vi "WVDIAL_3A_Data_v1.vi"() -> ()   [LabVIEW 2012]
uses:
  C:/H2O_DIAL/LabVIEW-2012/Newport_LabVIEW_v3-0-2/LabVIEW 2009/PowerMeterCommands.dll
  H2O_DIAL/LabVIEW-2012/Newport_LabVIEW_v3-0-2/LabVIEW 2009/PowerMeterCommands.dll
  <vilib>/DAQmx/write.llb/DAQmx Write (Digital 1D Bool NChan 1Samp 1Line).vi
  <vilib>/DAQmx/miscellaneous.llb/DAQmx Fill In Error Info.vi
  <vilib>/Analysis/baseanly.llb/Mean (DBL).vi
  H2O_DIAL/LabVIEW-2012/Scalar_Data.vi
  H2O_DIAL/LabVIEW-2012/Bristol WM V2_31b/CLDevIFace.dll
  <vilib>/Analysis/NI_AALBase.lvlib
panel:
  out "FileHour":i32=18
  out "L_Count":i32=437
  out "sigma_off_total":dbl[](array[numeric])=[4.970068414914426e-25, 4.935109344576291e-25, 4.900296426937575e-25, 4.865629933162525e-25, 4.8311101300892405e-25, 4.796737279795042e-25, 4.762511639263623e-25, 4.728433460005277e-25, 4.694502987714828e-25, 4.66072046190942e-25, 4.627086115623767e-25, 4.5936001750771025e-25, 4.560262859388569e-25, 4.5270743802518285e-25, 4.494034941687391e-25, 4.4611447397771265e-25, 4.428403962379541e-25, 4.395812788908677e-25, 4.363371390116038e-25, 4.331079927877316e-25, 4.298938554952973e-25, 4.2669474148461465e-25, 4.235106641622183e-25, 4.203416359713408e-25, 4.171876683809042e-25, 4.14048771871945e-25, 4.1092495592023437e-25, 4.0781622899252965e-25, 4.047225985294158e-25, 4.016440709475411e-25, 3.9858065161821437e-25, 3.955323448748479e-25, 3.9249915399689097e-25, 3.8948108121823377e-25, 3.864781277119762e-25, 3.8349029359894115e-25, 3.8051757794122746e-25, 3.7755997874807175e-25, 3.7461749297351587e-25, 3.7169011652144367e-25, 3.687778442479969e-25, 3.6588066996856557e-25, 3.629985864619472e-25, 3.6013158547695413e-25, 3.572796577416277e-25, 3.544427929672661e-25, 3.516209798625218e-25, 3.488142061394692e-25, 3.460224585304242e-25, 3.432457227878348e-25, 3.4048398370653397e-25, 3.3773722513359157e-25, 3.350054299768194e-25, 3.3228858022516937e-25, 3.295866569574933e-25, 3.268996403598237e-25, 3.2422750973929355e-25, 3.21570243540853e-25, 3.189278193592863e-25, 3.163002139636937e-25, 3.136874033014969e-25, 3.110893625253726e-25, 3.085060660050822e-25, 3.059374873481082e-25, 3.0338359941112116e-25, 3.008443743235647e-25, 2.9831978349953457e-25, 2.95809797659182e-25, 2.9331438684538516e-25, 2.9083352043781934e-25, 2.8836716717543507e-25, 2.859152951716739e-25, 2.834778719288951e-25, 2.810548643615105e-25, 2.7864623880639067e-25, 2.7625196104499907e-25, 2.738719963159808e-25, 2.7150630933496113e-25, 2.691548643092545e-25, 2.6681762495199362e-25, 2.6449455450241973e-25, 2.6218561573515237e-25, 2.5989077097963764e-25, 2.5760998213569394e-25, 2.553432106812723e-25, 2.5309041769453305e-25, 2.508515638628236e-25, 2.486266094966773e-25, 2.4641551454270873e-25, 2.4421823859627355e-25, 2.4203474091280046e-25, 2.398649804208083e-25, 2.3770891573121883e-25, 2.3556650514992666e-25, 2.334377066857522e-25, 2.3132247806240595e-25, 2.292207767270247e-25, 2.2713255985837977e-25, 2.250577843763165e-25, 2.2299640695179534e-25, 2.209483840081283e-25, 2.1891367173745365e-25, 2.1689222609956e-25, 2.1488400283134808e-25, 2.1288895745535377e-25, 2.1090704528070817e-25, 2.089382214122218e-25, 2.0698244075371163e-25, 2.0503965801268946e-25, 2.0310982770672953e-25, 2.0119290416275883e-25, 1.9928884152720694e-25, 1.9739759376467061e-25, 1.9551911466442564e-25, 1.9365335784015228e-25, 1.9180027673647352e-25, 1.8995982463109612e-25, 1.8813195463488326e-25, 1.8631661969818019e-25, 1.8451377261048445e-25, 1.8272336600511332e-25, 1.8094535235979458e-25, 1.7917968400156795e-25, 1.774263131074251e-25, 1.7568519170769187e-25, 1.7395627168958116e-25, 1.7223950479810698e-25, 1.7053484264204325e-25, 1.6884223669495872e-25, 1.671616383006639e-25, 1.6549299867335668e-25, 1.6383626890674343e-25, 1.6219139997488532e-25, 1.6055834273756572e-25, 1.5893704794600627e-25, 1.573274662463159e-25, 1.5572954818878462e-25, 1.5414324422878638e-25, 1.5256850473874784e-25, 1.510052800101514e-25, 1.4945352026447543e-25, 1.4791317565791618e-25, 1.4638419629201228e-25, 1.448665322199304e-25, 1.4336013345653925e-25, 1.4186494998679763e-25, 1.403809317759688e-25, 1.3890802877992275e-25, 1.374461909533494e-25, 1.3599536826304997e-25, 1.3455551069680852e-25, 1.331265682750014e-25, 1.317084910617463e-25, 1.3030122917788643e-25, 1.2890473280950027e-25, 1.2751895222264232e-25, 1.261438377738064e-25, 1.247793399209599e-25, 1.2342540923695054e-25, 1.2208199641934536e-25, 1.207490523039559e-25, 1.194265278734551e-25, 1.1811437427102546e-25, 1.1681254280970297e-25, 1.1552098498187396e-25, 1.1423965247193127e-25, 1.129684971621386e-25, 1.1170747114439217e-25, 1.1045652672740435e-25, 1.0921561644348792e-25, 1.0798469305651514e-25, 1.0676370956928575e-25, 1.055526192264184e-25, 1.0435137552017687e-25, 1.0315993219529312e-25, 1.0197824325066935e-25, 1.0080626294155857e-25, 9.964394578070562e-26, 9.849124653878678e-26, 9.734812024396337e-26, 9.621452217958014e-26, 9.509040788153638e-26, 9.397573313474797e-26, 9.2870453969155e-26, 9.177452665388814e-26, 9.068790769077486e-26, 8.961055380771591e-26, 8.854242195025276e-26, 8.748346927326784e-26, 8.643365313126359e-26, 8.539293106813325e-26, 8.436126080659389e-26, 8.333860023704058e-26, 8.232490740501524e-26, 8.132014049957187e-26, 8.032425783987688e-26, 7.933721786336048e-26, 7.835897911055001e-26, 7.738950021374666e-26, 7.642873988181704e-26, 7.547665688745864e-26, 7.453321005260971e-26, 7.3598358236196e-26, 7.267206031959588e-26, 7.17542751940349e-26, 7.084496174723345e-26, 6.99440788514668e-26, 6.905158535007224e-26, 6.816744004751336e-26, 6.729160169573299e-26, 6.64240289857379e-26, 6.5564680535091e-26, 6.471351488011949e-26, 6.387049046546095e-26, 6.303556563639124e-26, 6.220869863111731e-26, 6.138984757339889e-26, 6.057897046626043e-26, 5.977602518710106e-26, 5.898096948146685e-26, 5.819376096018969e-26, 5.741435709543367e-26, 5.664271521783085e-26, 5.587879251486328e-26, 5.51225460295526e-26, 5.437393265946454e-26, 5.363290915754907e-26, 5.289943213256812e-26, 5.217345804999475e-26, 5.1454943235195867e-26, 5.074384387521688e-26, 5.0040116022138814e-26, 4.9343715597454284e-26, 4.8654598395691204e-26, 4.7972720089551445e-26, 4.729803623551307e-26, 4.663050227875443e-26, 4.597007356046831e-26, 4.531670532379107e-26, 4.4670352720694333e-26, 4.4030970819662006e-26, 4.3398514613184746e-26, 4.2772939025846054e-26, 4.215419892254647e-26, 4.154224911690283e-26, 4.093704438021407e-26, 4.0338539450472376e-26, 3.9746689041273814e-26, 3.916144785197283e-26, 3.8582770576425204e-26, 3.8010611913639447e-26, 3.74449265772608e-26, 3.6885669306098596e-26, 3.6332794874218655e-26, 3.578625810171199e-26, 3.5246013865492145e-26, 3.4712017109920907e-26, 3.418422285823819e-26, 3.3662586223724155e-26, 3.31470624215432e-26, 3.2637606780392576e-26, 3.2134174754533765e-26, 3.163672193659779e-26, 3.114520407010239e-26, 3.0659577062623985e-26, 3.017979699957737e-26, 2.970582015834633e-26, 2.9237603022681873e-26, 2.877510229831183e-26, 2.831827492878117e-26, 2.786707811220407e-26, 2.7421469318983614e-26, 2.698140631035692e-26, 2.6546847158190514e-26, 2.6117750266015116e-26, 2.56940743913942e-26, 2.527577866977577e-26]
  out "sigma_on_total":dbl[](array[numeric])=[3.533865838600727e-23, 3.533764161681225e-23, 3.5333977469404133e-23, 3.53276568192525e-23, 3.531867144357016e-23, 3.530701403122502e-23, 3.529267819280469e-23, 3.527565846749943e-23, 3.525595033343317e-23, 3.523355021225782e-23, 3.52084554780571e-23, 3.5180664458671094e-23, 3.5150176447433637e-23, 3.511699169858595e-23, 3.508111143749733e-23, 3.5042537860569434e-23, 3.5001274136929736e-23, 3.495732440751245e-23, 3.4910693790546564e-23, 3.486138837361377e-23, 3.4809415218446414e-23, 3.4754782353092596e-23, 3.4697498774262163e-23, 3.463757443779839e-23, 3.4575020259466816e-23, 3.450984810279872e-23, 3.444207077926451e-23, 3.4371702036366597e-23, 3.429875655153695e-23, 3.422324992434722e-23, 3.414519866506169e-23, 3.406462018237782e-23, 3.3981532779195215e-23, 3.3895955634047386e-23, 3.3807908790536376e-23, 3.371741314710812e-23, 3.3624490438242643e-23, 3.352916322385855e-23, 3.3431454873140853e-23, 3.3331389544696416e-23, 3.322899217813418e-23, 3.3124288469010065e-23, 3.301730485625495e-23, 3.2908068501003093e-23, 3.2796607270971934e-23, 3.268294971825446e-23, 3.256712506069342e-23, 3.244916316282518e-23, 3.2329094515384454e-23, 3.2206950210285986e-23, 3.208276192552656e-23, 3.1956561900495705e-23, 3.182838291197626e-23, 3.169825825503171e-23, 3.156622172157982e-23, 3.143230757250406e-23, 3.129655051889506e-23, 3.115898569897651e-23, 3.101964865071464e-23, 3.087857529576123e-23, 3.0735801908728846e-23, 3.059136509681361e-23, 3.0445301776261984e-23, 3.0297649149870386e-23, 3.014844467928977e-23, 2.9997726067801886e-23, 2.984553123065604e-23, 2.969189827592652e-23, 2.9536865479241003e-23, 2.938047126177763e-23, 2.922275416635555e-23, 2.906375283683212e-23, 2.8903505991494374e-23, 2.874205240602245e-23, 2.8579430887383764e-23, 2.8415680253195745e-23, 2.82508393124097e-23, 2.8084946841160186e-23, 2.791804156410952e-23, 2.775016213305788e-23, 2.758134710797806e-23, 2.741163493435856e-23, 2.7241063929107007e-23, 2.706967225870395e-23, 2.6897497917834795e-23, 2.67245787185707e-23, 2.6550952266852455e-23, 2.6376655947539815e-23, 2.6201726909898208e-23, 2.602620204658551e-23, 2.585011798410415e-23, 2.567351106279476e-23, 2.5496417325287913e-23, 2.5318872500516e-23, 2.5140911992175055e-23, 2.4962570863782866e-23, 2.478388382719878e-23, 2.4604885230681298e-23, 2.4425609047468987e-23, 2.4246088864884145e-23, 2.4066357872066157e-23, 2.3886448853935633e-23, 2.3706394178067187e-23, 2.3526225788721896e-23, 2.334597519574035e-23, 2.3165673470495877e-23, 2.2985351233053837e-23, 2.2805038652795363e-23, 2.2624765434766603e-23, 2.2444560819400773e-23, 2.2264453571767302e-23, 2.2084471983084252e-23, 2.1904643861833434e-23, 2.1724996530784972e-23, 2.1545556824440762e-23, 2.136635108601783e-23, 2.1187405163135526e-23, 2.100874440657105e-23, 2.0830393670250524e-23, 2.065237730648886e-23, 2.0474719169339744e-23, 2.0297442610630612e-23, 2.0120570479000407e-23, 1.99441251242831e-23, 1.9768128394698823e-23, 1.9592601638590192e-23, 1.9417565706452558e-23, 1.924304095004353e-23, 1.9069047227470338e-23, 1.8895603902907944e-23, 1.8722729850622773e-23, 1.8550443455314435e-23, 1.8378762617450945e-23, 1.820770475568794e-23, 1.8037286811080227e-23, 1.7867525247724614e-23, 1.7698436060480647e-23, 1.7530034776056003e-23, 1.7362336461037145e-23, 1.7195355721920076e-23, 1.7029106711306976e-23, 1.6863603134193034e-23, 1.6698858252916527e-23, 1.6534884890145584e-23, 1.63716954348968e-23, 1.6209301849331533e-23, 1.60477156721748e-23, 1.588694802641815e-23, 1.5727009624323412e-23, 1.5567910770556656e-23, 1.5409661373460546e-23, 1.5252270946308514e-23, 1.5095748614057346e-23, 1.4940103122680925e-23, 1.4785342840755586e-23, 1.4631475768885227e-23, 1.4478509545243766e-23, 1.4326451449334203e-23, 1.4175308413235602e-23, 1.4025087021701827e-23, 1.3875793525189545e-23, 1.3727433838876403e-23, 1.3580013555586498e-23, 1.343353794787248e-23, 1.3288011974928065e-23, 1.3143440291718864e-23, 1.2999827250041545e-23, 1.2857176909889406e-23, 1.2715493042210399e-23, 1.2574779136743427e-23, 1.2435038406476323e-23, 1.2296273795897267e-23, 1.2158487985896458e-23, 1.2021683398687662e-23, 1.188586220584104e-23, 1.1751026331530729e-23, 1.1617177461950758e-23, 1.1484317046447017e-23, 1.135244630728007e-23, 1.122156624270959e-23, 1.1091677634521571e-23, 1.0962781051059955e-23, 1.0834876854596991e-23, 1.0707965206168882e-23, 1.0582046069909467e-23, 1.0457119219651325e-23, 1.033318424310305e-23, 1.021024054690317e-23, 1.0088287362915885e-23, 9.967323750441938e-24, 9.847348603691572e-24, 9.728360654323054e-24, 9.610358478667504e-24, 9.493340499304087e-24, 9.377304991678786e-24, 9.262250087660485e-24, 9.148173779875396e-24, 9.035073926354827e-24, 8.922948254293509e-24, 8.811794363756489e-24, 8.701609733235274e-24, 8.592391720879678e-24, 8.484137572151639e-24, 8.376844418698043e-24, 8.270509287268366e-24, 8.165129099242811e-24, 8.060700676024721e-24, 7.957220741783683e-24, 7.854685928236838e-24, 7.75309277619759e-24, 7.652437739190472e-24, 7.552717187295178e-24, 7.453927410213606e-24, 7.3560646196222e-24, 7.259124952139626e-24, 7.163104472849435e-24, 7.067999177776843e-24, 6.973804996017076e-24, 6.880517793951143e-24, 6.788133375712249e-24, 6.696647487854966e-24, 6.606055820037511e-24, 6.5163540092020856e-24, 6.427537639899013e-24, 6.339602248315714e-24, 6.2525433236464834e-24, 6.1663563105506496e-24, 6.081036610732605e-24, 5.9965795860817225e-24, 5.912980559342424e-24, 5.8302348176413195e-24, 5.748337612314408e-24, 5.6672841625673986e-24, 5.5870696569818e-24, 5.507689254030517e-24, 5.4291380852561205e-24, 5.351411255705527e-24, 5.274503846722599e-24, 5.198410916550372e-24, 5.123127502086537e-24, 5.0486486205742874e-24, 4.974969270795588e-24, 4.90208443445557e-24, 4.829989077525111e-24, 4.758678151750343e-24, 4.688146595694665e-24, 4.618389335962424e-24, 4.549401288384449e-24, 4.481177359166858e-24, 4.413712446003614e-24, 4.347001439343344e-24, 4.281039222858322e-24, 4.215820675401598e-24, 4.1513406710368785e-24, 4.087594080368749e-24, 4.0245757716323364e-24, 3.9622806110463586e-24, 3.9007034643748235e-24, 3.839839197225054e-24, 3.779682676024476e-24, 3.720228768630579e-24, 3.661472345407886e-24, 3.603408279778253e-24, 3.5460314487618505e-24, 3.489336733660721e-24, 3.433319021017125e-24, 3.377973202932029e-24, 3.3232941781131374e-24, 3.269276851437536e-24, 3.21591613582854e-24, 3.163206951786573e-24, 3.1111442286197847e-24, 3.0597229042579586e-24, 3.0089379262915793e-24, 2.9587842521682336e-24, 2.9092568499034787e-24, 2.8603506978798334e-24]
  out "background start":u32=269
  in  "Tab Control 2":enum32{"WV ND far", "WV ND near"}(tab)
  out "Water Vapor Number Density":dbl[][](graph)=[[0.7439747828579918, 1.8131789067403457, 1.729834500088495, 1.0387417363766693, 0.6183367881896566, 0.6091095409950267, 0.6810075295759752, 0.7659212586949528, 0.8022145297247747, 0.5880760880308791, 0.4305802055614884, 0.5184392448936054, 0.13311923215096755, -0.5099265277358037, -0.4712215809659876, -0.01634168865715292, 0.350144679474652, 0.3991315130339072, 0.25580712571211667, 0.22365563488734505, 0.2740454949683393, 0.3307517543329355, 0.5700258642908436, 1.0196890684218016, 1.3866709744259715, 1.65704424557237, 2.3745736070264782, 3.3112894291607247, 1.0483993923883888, 6.509122898471465, 4.345208749120676, -20.01503487017629, 5.551454849842233, -6.0803419680963815, -1.2151459132208435, 6.716139594512968, -23.69860833719387, 3.512080037255953, 4.673497483582146, -15.030922332981946, -5.469844384586185, -2.1669099779261813, 0.7498420910970466, 0.06843337831190982, -2.1897016922563357, 2.2405490774816887, 5.428632752263166, 6.792937491411026, 2.5053559409822497, 1.5383708256405055, 1.240825229423066, 1.8764254172701609, -0.1985197629707374, -1.6347727626176671, 4.043313035079826, 2.9131590136164447, 1.0298293809226633, 1.3099144696842249, -1.286195249282649, -1.1272409618021992, 2.9842167413436558, 2.061719511311547, -0.8528650966747232, -1.4313233537889116, -2.097215524113984, -0.8447582180717865, -2.3503598510538155, -2.6213429378596436, 0.5334270380975938, 0.20155201777734583, -2.595768905085648, -1.7635156261206875, 1.6742459437289348, 3.6197856740036514, 1.1850754318857877, -3.2521915171548414, -2.5568838707652013, 1.6157908913671968, 0.02435528898435081, 0.3845705314592533, 0.9939377479538306, -1.1637047496471227, -0.08717887603005632, 0.6411905616223332, -0.5723289554676214, 1.917259977443995, 4.402312871132401, 4.437817753147878, 2.016231660477841, -0.34835292580982036, 0.6885983825349437, 2.5777888939441618, -0.8473766569331534, -1.8686815495545002, 2.045891104581793, 5.086437836872098, 0.16199215377137235, -7.141507342331465, -5.2645001784747665, -2.8087586831282954, -2.5692449708616873, -0.9355382771726125, -0.8582448783717992, 0.9491993939359095, -1.4633527537274644, -7.147063550386115, -2.2341695281673752, 2.5555711007833564, 2.3272340744460696, -0.5264109226880953, -1.376362810416861, -0.28169049538621105, 0.27737305169984594, -2.4340096029821336, -0.8850629506045988, 2.117533423011808, -1.2789034896844858, -1.0863518179624383, 2.8066642800093438, 6.814730787546482, 5.4137020975551025, 0.24734223970510483, -7.704161161112219, -9.922411319316524, -3.6008799564723484, -3.572835272935353, -0.3952342529170262, -7.605784685328365, -12.746335553316083, -2.7857807808459363, -7.427033436521031, -10.117791768496497, 18.632132632336372, 10.425040587596978, 4.380676792053731, 3.735063762502258, 2.4013900219549034, 5.910781676835607, 6.5855028943485205, -3.1204952923130156, 3.67306395875442, 9.54228505946667, -9.146612074141558, 2.379755608898987, -3.062830785635178, -3.885890048345421, 7.205797035489026, -3.144468146358709, 11.996065933696075, 7.413029247362674, 1.8471650169286589, -0.13850816976625957, 1.8532319828102617, 0.24087944010728557, 5.280804054484616, 8.915827188675628, -3.889913258806417, 2.893589079216625, -5.7571550550948745, -2.2128143428753613, -6.6305897357939045, -0.9960889646807097, 1.16953044813146, -1.981312747485014, -5.292602716896448, 1.3169420785889991, 1.6760295938618295, 0.3648306991074169, -12.328626800192753, -9.186942372060514, 18.434308239870823, 4.705319759089772, -2.1920706804850303, -4.059967071819086, -7.134306158367519, -8.837074111676458, -12.379854542395988, -9.485796968311545, 7.116377101382049, 3.416423640263124, -15.75980393588494, -17.318914146327707, -2.6873036408670834, -7.24384081619992, 10.856824935856261, 10.85098989334328, -13.376967531177051, 5.089162812882581, -11.464960663387709, 18.063529389635153, 28.957831831841137, 20.11698529067015, -17.834743999270017, 4.971781683382732, -11.636385451734613, -20.05838696514341, 14.983286338818427, 7.900517890395745, 18.480392736239335, -14.37191562761992, -41.775307205543406, -12.530456247555255, 42.43024575182168, -0.7120594990142516, 16.50744401601535, 22.21122371485303, 62.234322576029186, 0.9757230155075491, -38.92617294487387, -31.50777178347162, -7.379649094423733, -16.69670090306499, -4.831754611139989, 20.65063215343611, 12.066912928811204, -6.3884013860598685, -10.241236202775962, -4.160701018297583, 34.51142590392718, 47.10817201518173, 33.4125284772157, 9.982145423615565, 8.383142278161076, -15.634391173698468, -11.884196735494013, -27.976124344969215, -10.316574529474243, 11.248564633808689, -17.532376581278363, -49.793126403148094, -5.051302269078928, 44.70232009697591, -27.768858567793224, -17.916293850831167, -26.425916913974742, 20.16002519520873, -10.268802741102817, 11.373570298339766, -6.35394154173542, -7.21903570553281, 49.69486756487177, -47.53623215885525, 16.99487126005546, 2.7627149195214527, 13.516547770742644, -37.88119720865505, 34.79710949694299, 34.23048773253234, 6.902914859856622, 27.453276837967298, -80.88234649474579, -4.93255276195487, -13.899224055886746, -14.250099183966608, 16.107083983411574, 44.44722285618612, -17.853730845820905, -91.32981904709379, 26.124610427458858, -3.0936150698622367, -23.167534565524495, 26.685349701423544, 18.260971138401164, -61.42035137478399, -50.06846587212657, 0.2813738061771184, -54.16407086468557, 11.407705733747363, -50.99571577991077, 22.977665732742363, 69.98334663450075, 15.472386561952685, 0.462653265199104, 114.4891486062606, 61.367298698998255, 17.34554696705243, 0.0, 0.0, 0.0, 0.0]]
  out "Water Vapor Number Density 2":dbl[][](graph)=[[-10.93662459142193, 19.510484173911763, 17.15483545215336, -11.606996277475266, 1.3304885261452224, -0.5271750850183562, -1.611801991101525, -1.8770890565551748, 0.6482559597852942, 1.1002445378415513, -0.12331444949229987, 0.09388084060187898, 0.3079507951532581, 0.2940020662581854, 0.4277223459374443, 0.5691075298971469, 0.6561873597795664, 0.6642421713978535, 0.585853479624924, 0.5518410763647447, 0.6672223052861218, 0.7936246580645427, 0.8233775544159819, 0.8446454528928528, 0.9261173914931705, 1.1358266563264032, 3.7027410772311002, -15.869586844857418, -14.143911544938991, 1.5960927966186407, -3.147749322042341, 0.6041618099447368, 1.9995101312458199, 4.386829575121968, 4.857157638273741, 2.2335710861286118, -0.43966030721716, -2.560470441673352, -4.113777530723239, -0.6837815147471296, 0.028020530649357955, -0.15368070068094847, -0.7533975836649077, -0.7376955694658232, 0.12837676182705, -0.101970204677087, -0.9113771063971142, -0.7912217527152914, -0.5155498671943642, -0.14221881934053993, -0.9980260835848688, -0.8663253480917944, -0.2078394226712728, 0.15516425152263164, 0.08123800041663636, 0.02964315987322877, 0.7211330433993742, 0.8411882741898078, 0.7509209545060699, -0.08356096341045686, -0.26928881890863515, -0.07806708511630893, 0.14928474853409204, -0.08626943317012713, -0.3025332798674882, 0.15278903019368337, 0.940546369420624, 0.3066205364696119, -1.040462894388828, 0.1800820883306482, 0.1632761734053667, -0.7607345085445149, 0.6682208515118813, 0.5690572371447694, -0.7863643897298066, -1.5303503114174708, -1.737165781994069, 1.2819000477166906, 2.4790847510868086, 0.36202085692407354, 0.7094550613429548, 1.100663607477538, -0.251496985251488, 0.3249046394435906, 1.5284049984028627, 1.8149429088741817, 1.0235046873522649, -0.8459291543413351, -0.9706547517793931, 1.5197354344894316, 1.9715357583225108, 0.7679139915699971, 1.2230921230445164, 0.10483387821173006, -0.9506988329926953, -1.3813530588498386, -0.4269273176512617, -0.2858184079844674, 0.45569562930849056, -0.9132124360706889, -3.704676215174936, -2.7520890636900894, -1.740358811892638, -0.9110124300450704, 0.20878573470425943, 0.9359054582845971, 1.0535639318225485, 0.9714863567986126, -0.124828486138746, -0.7659618364820846, 0.31832082971712666, 2.7857678728202178, 1.4527117557106253, 0.735595298146168, 0.1548941382968119, -0.31631105374500795, -0.7246602682569218, -0.7752206760402915, -0.6509670152727582, -0.43531824099195093, 0.9060751665784867, -1.4567882573076687, -2.3398717301175083, -2.540297886951049, 1.9625173291273508, 2.0426831790277387, -0.8306098968280333, -0.20510587354506535, 0.7417481626631306, -2.329608788881194, -0.5779296048334142, 1.1178194286379437, 0.4763522927574004, 2.406791016605482, -0.6530314577194056, -2.131954310719609, 0.11308511636047595, 0.5588017641449814, -2.3816128846513576, 0.04131161381481335, -1.0359727870472868, -1.7493131131734865, -0.4663315479300367, -0.1993229085950785, -1.4886649689818054, -0.3438795366028828, 0.3269845059610161, 0.9534661787645886, 4.333624235171587, 0.5208678797422068, -0.6419579206233043, 2.890262615412334, 10.893585954884003, -4.567581259006971, -4.509647044472795, -0.5549393385673885, -4.068309709640761, -8.252984385887535, -3.2011446606221976, 3.273186059367117, 2.050751858495942, -1.8492192126482796, -12.914542438448322, 1.1996608358244936, 8.901387929919956, 2.768407451583976, 1.5099997395885625, 3.8402709516838605, -0.7725071125086813, -3.0463961450023813, 0.4602229832193462, -0.16183374142844362, 0.3571415162839249, 1.8377574693684513, -15.41333758103779, -11.700354420145874, -2.857624340980594, -3.5643711537963187, -10.470556100757129, 5.068838949444352, 0.4922173831547322, -2.0196453023744683, -3.374990817101721, -5.350746774413054, 9.02355540080223, 9.041129942972974, 3.9907204311008853, 4.561561218325569, 10.259378359576727, -6.65335088184076, 1.861833783400288, 5.8559196895029295, 6.10358174629942, 12.121875782027866, 6.615528120240944, -3.95740678195961, -11.759351979703954, 9.486261359637128, -0.49459862435445034, -6.760160539443337, -4.025629589831995, -0.8900890038927379, 0.5945445613567323, 1.2933074628983436, 0.32318360398755713, 0.12588777550187805, 1.3233862818167614, -12.665262924294405, -12.05864739203146, -4.5503737980659595, -1.1824704049019195, 1.3491044690681344, 13.041322733477614, 22.26148813395544, 6.350013852401591, 33.90393006921492, 37.349769087497414, 32.97859684100176, 64.52361087397345, 29.31482179739505, 3.0833182266672026, -27.149549611536145, -19.853679397613792, -32.28738556233836, -37.50984572364252, -42.103861631165515, -32.49807551607822, -9.715116346920858, -41.330814789380454, -5.584584877219785, 22.118030629310038, 53.17031031299851, 17.97586430044937, 0.1720044365508073, 24.764414223397644, 4.139662926658314, -7.251766441432914, -20.437140064371427, -30.583873913523718, -15.175335921347479, -34.840723359732436, -43.484920286442964, -11.300080419951712, 4.090066944392005, -7.514494533126683, -27.42923008900803, 72.78750459687346, 32.08792307241346, 33.69894319724674, 1.4215953400804904, 16.143141681823614, 61.498906451567194, 11.698538631681785, -9.51590532608696, -8.13189158363684, 44.746670192850225, -37.28257936831558, 23.445747203451734, -8.375854194474655, -21.435303835433448, -20.20376077939404, -84.26096267020971, -31.360793615818423, 30.091313676028314, 44.892561326924366, -89.29302837497693, 42.92728517164177, -43.139196226653986, 32.88827285512054, 10.46855736494291, 63.8903907956293, 83.74682123645073, 66.7332289135973, 25.994761946655032, 19.952490840030084, 128.44210917845157, 0.0, 0.0, 0.0, 0.0]] caption="Water Vapor Number Density"
  out "RingBuffer offline near":dbl[][](array[numeric])
  out "RingBuffer aerosol near":dbl[][](array[numeric])=[[14734.3, 54666.3, -19.699999999999818, 26.300000000000182, 3.300000000000182, 38.30000000000018, 35.30000000000018, 93.30000000000018, -8.699999999999818, 92.30000000000018, -7.699999999999818, 8.300000000000182, 3.300000000000182, 81.30000000000018, 1268.3000000000002, 4383.3, 6631.3, 7225.3, 6853.3, 6144.3, 5802.3, 4915.3, 3550.3, 2733.3, 2094.3, 2468.3, 4106.3, 3083.3, 237.30000000000018, -46.69999999999982, -78.69999999999982, -70.69999999999982, -67.69999999999982, 4.300000000000182, -65.69999999999982, 43.30000000000018, -62.69999999999982, -50.69999999999982, -31.699999999999818, -34.69999999999982, -6.699999999999818, -91.69999999999982, -18.699999999999818, -64.69999999999982, -52.69999999999982, 81.30000000000018, -1.699999999999818, 9.300000000000182, 5.300000000000182, -40.69999999999982, -29.699999999999818, -47.69999999999982, -44.69999999999982, -2.699999999999818, 43.30000000000018, 8.300000000000182, -68.69999999999982, 53.30000000000018, -102.69999999999982, -85.69999999999982, -40.69999999999982, -75.69999999999982, -5.699999999999818, -86.69999999999982, -23.699999999999818, 12.300000000000182, 65.30000000000018, -3.699999999999818, 26.300000000000182, 16.300000000000182, -10.699999999999818, -24.699999999999818, -14.699999999999818, -47.69999999999982, -69.69999999999982, -47.69999999999982, 68.30000000000018, -100.69999999999982, 0.3000000000001819, -70.69999999999982, -10.699999999999818, -17.699999999999818, 15.300000000000182, -60.69999999999982, 25.300000000000182, 14.300000000000182, 28.300000000000182, -103.69999999999982, -59.69999999999982, -89.69999999999982, -1.699999999999818, -7.699999999999818, 44.30000000000018, -18.699999999999818, -7.699999999999818, -63.69999999999982, -32.69999999999982, -23.699999999999818, -45.69999999999982, -4.699999999999818, -75.69999999999982, -70.69999999999982, -59.69999999999982, -8.699999999999818, -49.69999999999982, -88.69999999999982, 12.300000000000182, -45.69999999999982, -97.69999999999982, 39.30000000000018, 23.300000000000182, 26.300000000000182, -79.69999999999982, -118.69999999999982, -70.69999999999982, -30.699999999999818, -1.699999999999818, 68.30000000000018, -1.699999999999818, -9.699999999999818, -21.699999999999818, 12.300000000000182, -40.69999999999982, -10.699999999999818, -19.699999999999818, 52.30000000000018, 7.300000000000182, 0.3000000000001819, -1.699999999999818, -78.69999999999982, -122.69999999999982, -75.69999999999982, -45.69999999999982, -118.69999999999982, -62.69999999999982, -33.69999999999982, 0.3000000000001819, 4.300000000000182, 22.300000000000182, -2.699999999999818, -18.699999999999818, -28.699999999999818, -2.699999999999818, 3.300000000000182, -74.69999999999982, -26.699999999999818, 54.30000000000018, -123.69999999999982, 92.30000000000018, -29.699999999999818, -47.69999999999982, 3.300000000000182, -29.699999999999818, -40.69999999999982, -84.69999999999982, 16.300000000000182, 25.300000000000182, 27.300000000000182, 10.300000000000182, -2.699999999999818, 12.300000000000182, -19.699999999999818, -115.69999999999982, -18.699999999999818, -57.69999999999982, -8.699999999999818, -75.69999999999982, -28.699999999999818, -20.699999999999818, -1.699999999999818, -54.69999999999982, -93.69999999999982, -52.69999999999982, 6.300000000000182, -52.69999999999982, -97.69999999999982, -40.69999999999982, -55.69999999999982, 14.300000000000182, -19.699999999999818, 14.300000000000182, 0.3000000000001819, -79.69999999999982, 27.300000000000182, 11.300000000000182, 38.30000000000018, -74.69999999999982, 21.300000000000182, -13.699999999999818, -41.69999999999982, 15.300000000000182, -54.69999999999982, -47.69999999999982, -49.69999999999982, -92.69999999999982, -22.699999999999818, -1.699999999999818, -7.699999999999818, -3.699999999999818, -101.69999999999982, -81.69999999999982, -49.69999999999982, 10.300000000000182, -37.69999999999982, -38.69999999999982, 28.300000000000182, -54.69999999999982, -85.69999999999982, -53.69999999999982, 4.300000000000182, -105.69999999999982, 19.300000000000182, -84.69999999999982, 18.300000000000182, 14.300000000000182, -55.69999999999982, -55.69999999999982, -42.69999999999982, -31.699999999999818, 28.300000000000182, -82.69999999999982, -123.69999999999982, -169.69999999999982, 59.30000000000018, -17.699999999999818, -68.69999999999982, -40.69999999999982, 25.300000000000182, -22.699999999999818, 7.300000000000182, -103.69999999999982, -50.69999999999982, 6.300000000000182, 19.300000000000182, 3.300000000000182, 93.30000000000018, -75.69999999999982, 50.30000000000018, -50.69999999999982, -18.699999999999818, 68.30000000000018, -23.699999999999818, -116.69999999999982, -86.69999999999982, 18.300000000000182, -35.69999999999982, 17.300000000000182, -14.699999999999818, -3.699999999999818, -29.699999999999818, 42.30000000000018, -0.6999999999998181, -44.69999999999982, 30.300000000000182, 24.300000000000182, -49.69999999999982, 3.300000000000182, -61.69999999999982, -11.699999999999818, -48.69999999999982, -35.69999999999982, -27.699999999999818, 20.300000000000182, -32.69999999999982, -56.69999999999982, 68.30000000000018, 60.30000000000018, -9.699999999999818, 31.300000000000182, -25.699999999999818, 14.300000000000182, 12.300000000000182, -36.69999999999982, 11.300000000000182, 60.30000000000018, -82.69999999999982, 59.30000000000018, 36.30000000000018, -48.69999999999982], [15122.2, 54960.2, 26.199999999999818, -18.800000000000182, 4.199999999999818, 52.19999999999982, 46.19999999999982, 133.19999999999982, 104.19999999999982, 73.19999999999982, 37.19999999999982, -10.800000000000182, 35.19999999999982, 35.19999999999982, 799.1999999999998, 2369.2, 4881.2, 6292.2, 6622.2, 6164.2, 5398.2, 4772.2, 3455.2, 3068.2, 3604.2, 4025.2, 3889.2, 2118.2, 194.19999999999982, -3.800000000000182, -59.80000000000018, -28.800000000000182, -29.800000000000182, 14.199999999999818, -9.800000000000182, 38.19999999999982, -71.80000000000018, -31.800000000000182, -3.800000000000182, 57.19999999999982, -12.800000000000182, 48.19999999999982, 26.199999999999818, -91.80000000000018, 31.199999999999818, -59.80000000000018, -26.800000000000182, -27.800000000000182, 28.199999999999818, -78.80000000000018, 0.1999999999998181, -0.8000000000001819, 49.19999999999982, -68.80000000000018, -30.800000000000182, -47.80000000000018, 7.199999999999818, 22.199999999999818, -43.80000000000018, -8.800000000000182, -49.80000000000018, 20.199999999999818, 82.19999999999982, -64.80000000000018, 33.19999999999982, -6.800000000000182, -34.80000000000018, 87.19999999999982, 89.19999999999982, -11.800000000000182, 40.19999999999982, -61.80000000000018, -82.80000000000018, -39.80000000000018, 10.199999999999818, 2.199999999999818, -7.800000000000182, -13.800000000000182, -67.80000000000018, -68.80000000000018, -18.800000000000182, -62.80000000000018, -8.800000000000182, 17.199999999999818, -17.800000000000182, 32.19999999999982, 6.199999999999818, -17.800000000000182, -19.800000000000182, 40.19999999999982, -31.800000000000182, 46.19999999999982, -20.800000000000182, -54.80000000000018, -17.800000000000182, -2.800000000000182, 1.199999999999818, -70.80000000000018, -81.80000000000018, 4.199999999999818, -9.800000000000182, 28.199999999999818, -9.800000000000182, -7.800000000000182, 97.19999999999982, 44.19999999999982, 38.19999999999982, 7.199999999999818, 35.19999999999982, 9.199999999999818, -20.800000000000182, 65.19999999999982, -12.800000000000182, 21.199999999999818, 27.199999999999818, -46.80000000000018, 9.199999999999818, -45.80000000000018, -34.80000000000018, 7.199999999999818, -107.80000000000018, 52.19999999999982, 37.19999999999982, -31.800000000000182, -33.80000000000018, -30.800000000000182, -44.80000000000018, -38.80000000000018, 89.19999999999982, 30.199999999999818, 97.19999999999982, 69.19999999999982, -59.80000000000018, 3.199999999999818, 68.19999999999982, -63.80000000000018, -14.800000000000182, 21.199999999999818, 40.19999999999982, 9.199999999999818, 22.199999999999818, 67.19999999999982, -2.800000000000182, 47.19999999999982, 28.199999999999818, 29.199999999999818, -34.80000000000018, -32.80000000000018, -28.800000000000182, -83.80000000000018, -15.800000000000182, 21.199999999999818, 18.199999999999818, 24.199999999999818, 22.199999999999818, 15.199999999999818, 68.19999999999982, 3.199999999999818, -5.800000000000182, 189.19999999999982, -57.80000000000018, -6.800000000000182, 13.199999999999818, 61.19999999999982, -25.800000000000182, 38.19999999999982, 3.199999999999818, 2.199999999999818, 35.19999999999982, -29.800000000000182, 57.19999999999982, -21.800000000000182, 43.19999999999982, -3.800000000000182, -40.80000000000018, 6.199999999999818, 30.199999999999818, -11.800000000000182, -52.80000000000018, 2.199999999999818, -14.800000000000182, 32.19999999999982, -0.8000000000001819, -15.800000000000182, 39.19999999999982, 114.19999999999982, -5.800000000000182, 22.199999999999818, 15.199999999999818, 22.199999999999818, 50.19999999999982, -1.800000000000182, 82.19999999999982, -14.800000000000182, -62.80000000000018, 54.19999999999982, 90.19999999999982, 106.19999999999982, -15.800000000000182, -24.800000000000182, -161.80000000000018, -85.80000000000018, 78.19999999999982, 5.199999999999818, -48.80000000000018, 22.199999999999818, -23.800000000000182, 20.199999999999818, -20.800000000000182, 40.19999999999982, 16.199999999999818, -53.80000000000018, 12.199999999999818, -11.800000000000182, 58.19999999999982, 28.199999999999818, -28.800000000000182, -53.80000000000018, 56.19999999999982, 24.199999999999818, -51.80000000000018, -59.80000000000018, 37.19999999999982, 50.19999999999982, -22.800000000000182, 17.199999999999818, -36.80000000000018, -37.80000000000018, 6.199999999999818, 75.19999999999982, 9.199999999999818, -47.80000000000018, 26.199999999999818, -6.800000000000182, -16.800000000000182, 42.19999999999982, -52.80000000000018, 11.199999999999818, 20.199999999999818, -17.800000000000182, -75.80000000000018, 73.19999999999982, -79.80000000000018, 51.19999999999982, -23.800000000000182, 8.199999999999818, 79.19999999999982, 43.19999999999982, -29.800000000000182, -16.800000000000182, -37.80000000000018, 7.199999999999818, 47.19999999999982, 2.199999999999818, -37.80000000000018, -0.8000000000001819, 25.199999999999818, -16.800000000000182, -14.800000000000182, -64.80000000000018, 43.19999999999982, 107.19999999999982, 56.19999999999982, -6.800000000000182, 49.19999999999982, -25.800000000000182, 39.19999999999982, 119.19999999999982, -21.800000000000182, 40.19999999999982, 9.199999999999818, -116.80000000000018, -19.800000000000182, 10.199999999999818, 81.19999999999982, 42.19999999999982, -19.800000000000182, 40.19999999999982, -66.80000000000018]]
  in  "?":T1(tab)=enum."Raw Counts far"
  out "NRB":dbl[][](graph)=[[0.009791832890775209, 0.02826952822434131, 0.00012561268412980496, 0.0002473866123388622, 0.0006664616070220018, 0.0019180351127190153, 0.0043881080154924935, 0.008718663243067718, 0.013587190857225852, 0.017540758372662547, 0.021927441421116006, 0.027619102663731226, 0.05416724924095812, 0.3379776000970848, 1.2740502813225303, 2.7798844477372495, 4.109139494312893, 4.812805338579539, 4.926028752312164, 4.801513803064729, 4.501416893901011, 3.7785556478790134, 3.060778174380073, 2.816093080630355, 3.0012962074307326, 3.5165972350747987, 3.207267287107378, 1.376890630681026, 0.1330700898278606, 0.0017755012838220781, -0.0005867480475985722, 0.0008657297279965372, 0.001790273896358966, 0.0012488191923237916, 0.0016686021982468316, -0.0004869495028355791, -0.000514377985634188, 0.0009495151047675503, -0.0011429617452732783, -0.003231091091370898, 0.002763499008061912, 0.004557229787494368, 0.0011289796332456172, -0.0005455658173808351, 0.0005706587575732132, 0.0024846840754415094, 0.00031125387294316626, 0.0060605350045499105, 0.0014660249320836813, -0.0041093700977171575, 0.0008551443011271243, 0.004953339208967786, -0.0009235055770099291, -0.002054291560037214, 0.006109755492665881, 0.0060393235416529205, -0.0010681629119634246, -0.00853103367159078, -0.0029427774303289367, 0.00439634897120925, 0.008564274456504177, 0.0030693143117634268, 0.004101255908599104, 0.0055792609012400175, -0.0015874704085496307, 0.0055241918130361336, 0.0023192444411779603, -0.0008687003071111086, -0.007378718372229293, -0.011966108674057474, -0.005918776752260374, 0.003165294980392255, 0.01226525626947346, 0.005915686762253533, 0.009775734910433145, 0.006239774787943098, -0.003341553467610834, -0.001428731312645312, -0.0032242847630790925, -0.003907583251436901, -0.012017071032783095, -0.013894417356206947, -0.007117976236278598, 0.011599791196243216, 0.016289700900799793, -0.01180983494409668, -0.028435408606816, -0.022547713269548665, -0.007068279223175076, 0.00038043564571908886, -0.013222991234730207, -0.006360307831685095, 0.015031169998282006, 0.002490044830576252, -0.001271631942720581, 0.012986234791525842, 0.009280578478009616, -0.004059595795589597, -0.02163345033636912, -0.030055491453871278, -0.02395343937920574, -0.020033026882827633, -0.007473929753235528, 0.0, -0.006731422710483098, -0.015830849257402232, -0.023658117833315485, -0.013147246657756892, 0.008370505939559276, 0.0011366123076664105, 0.0005786848877660362, 0.008248419303465478, 0.01259471852329735, 0.01587081978606539, 0.0031057399503750423, -0.011375470583885713, -0.0019287944225930232, 0.02223646164964081, 0.023945327644043342, 0.022996627962857487, -0.01375244809419117, -0.04263789648861244, -0.029841529716575173, -0.03538305962288628, -0.014676729832097335, -0.017149275980826544, -0.026512012122432017, -0.016928570569776247, -0.021883172821289848, 0.02460757023739853, 0.03627327021874447, 0.022096767252144534, 0.025756408871558736, 0.010120358139587548, -0.0034238890780925505, -0.006080868334772392, -0.006170621635777629, -0.014310692621291459, 0.017242247533730336, 0.009205756856998797, -0.013072250729714768, 0.011364830782281314, -0.017287232310484464, -0.01266056973465556, 0.03357667381382491, 0.05106370522223785, 0.039584580978766604, 0.020576187354226953, -0.020853637056153146, -0.0063405118238991694, 0.026773762572845854, -0.02061678110999078, -0.03188253850020081, 0.05124266220899599, 0.03949617112949877, -0.0342879625781542, -0.011576749419720662, -0.024621354535632446, -0.05817632221164073, -0.016832635112957, 0.0012174410336647534, 0.02588580099658671, 0.052414770677631985, -0.03915793789283991, -0.07926930446325701, 0.023296922250656805, 0.05370876730011426, 0.03579311059025064, 0.017439041268322377, 0.009501603345856934, -0.008240129166339358, -0.020841619174259578, -0.06043957829602475, -0.00426592007731948, 0.09062807280151815, 0.024733371519558768, 0.03825922692194849, 0.06250553630735413, 0.03461368143706455, 0.06239607230534267, 0.05231892560355376, -0.031113727933337096, -0.03460210570136943, -0.02544123132674038, -0.07072225372043169, -0.0779872963692591, -0.016423682520922217, -0.024899479045938026, -0.0436185680976159, 0.022042274072561804, 0.0, -0.03808928378199656, 0.010497021264614626, 0.11667986253714252, 0.06965633262610949, -0.014434145139607717, -0.07290471594643992, -0.05523608172723363, 0.031620165468299544, -0.1634197684072646, -0.16505805158554743, 0.06133012604209659, 0.058067464141057776, -0.11335404380095591, -0.11249470265090368, -0.021923689826313788, 0.020125381406405178, 0.06705984648401497, 0.04513654808352671, -0.03728138025782997, -0.01881895714446527, -0.02533020392111677, -0.09801112796612513, 0.021509532705261073, 0.14330764815015976, 0.08765870981169306, 0.057505465751464535, 0.13170670244486532, 0.08335182614031719, 0.06592681338379318, 0.0734100746500843, 0.0486113327357026, 0.10978444237620111, 0.06598906695351175, 0.002377722785744305, -0.02398856153846616, -0.026621401947877352, -0.026856468374283536, 0.08621097649124015, 0.14412049266079316, 0.030075319151622353, -0.01769553726485668, -0.09433636971607413, -0.06429052565895041, 0.11154090812643745, 0.1779029060250453, 0.03693442792222197, -0.1037486620303255, -0.024144957459378738, 0.13257248285263115, 0.0736571590204205, -0.03300636486374783, -0.12479127291542674, -0.1733471923057657, 0.03101195089813033, 0.045477696169470776, -0.04298020363042193, 0.02310974574169569, 0.1368767763632256, 0.0998117533110134, -0.04142472049810171, 0.14914431969447547, 0.1803997682990584, 0.027271722327032667, 0.0458119812069558, 0.024624744682098215, 0.0186130569278781, -0.059398174247118525, -0.072460984005406, -0.0761963197928983, -0.21753571392433543, -0.08382052541901806, 0.1007148535947112, 0.02291431649802232, 0.029684988226422425, 0.09970204306740478, 0.06696748631736145, 0.013493610749759601, -0.020391367826185235, -0.1335230114753677, -0.07933106433030249, 0.013899411028489283, 0.021002778539839013, 0.08463053120023438, 0.13142932490693454, 0.13238691245104983, 0.007207531054126941, 0.0, 0.0, 0.0]] caption="Water Vapor Number Density"
  out "NRB 2":dbl[][](graph)=[[0.009003987035666773, 0.02630771851003072, 6.0012502719042654e-06, 1.1430974386315947e-05, 0.00011670940587340113, 0.00029500620209249194, 0.000719213893914681, 0.0009821064275591996, 0.001007391795393325, 0.0009290810298112261, 0.00015560764889456882, 0.00024691879385514026, 0.001247971649453338, 0.020471753347035514, 0.09611062415850778, 0.23061733529192172, 0.3615329788775301, 0.43880368123277025, 0.4659004365445802, 0.4685785011455833, 0.45665776097886074, 0.39726945043498113, 0.33063261760477614, 0.3224564196254475, 0.3714355369056685, 0.4795533966539507, 0.4698635006584886, 0.21258791701904534, 0.015271857935818157, -0.008098597518304563, -0.010888445012559565, -0.009604287607502178, -0.004096851752648524, -0.0031379493191144615, 0.000350067668191394, -0.0032711267418540357, -0.014143139839296935, -0.008113582320416127, -0.0009417198364426435, 0.00022861433084478676, -0.005043320876887893, -0.00302434588531786, -0.013117809676089446, -0.01640740258613208, 0.0, -0.000705452462082816, -0.004944415642874659, 0.0016460603116294967, -0.009832867244672274, -0.017736357052581725, -0.009661199474425569, -0.00566608663360105, -0.008962550477879763, -0.008193154302573521, -0.0038897963716928133, -0.0150825491472742, 0.0021664513481574397, -0.011374076466872286, -0.039937799783549686, -0.031709032846236204, -0.025867420326749352, 0.003844851599232184, -0.014175582215912618, -0.02769441215258109, 0.0030184916738865554, 0.007469293514117994, 0.02437851766061618, 0.04384228185003172, 0.02721680643901684, 0.00793528479872414, -0.01368373920212457, -0.045414276378780656, -0.04693817667710909, -0.03832838783538846, -0.028124569435163036, 0.004126581753460058, -0.015247227987540166, -0.05271956379866456, -0.0615056966188698, -0.05149777939442207, -0.03436629380239718, -0.023695112969525183, -0.012139127406301152, -0.01209738354127144, 0.01858384013013691, 0.028536967129696184, -0.03135786644206247, -0.0741066380942612, -0.048654632009177815, -0.03201511928635663, 0.0019720441572373825, 0.02499641492969604, -0.02059467062455846, -0.04165526057510147, -0.03953845592922844, -0.04300790737598615, -0.05645090785223986, -0.10150412674496608, -0.05973593195235647, -0.04095321634599031, -0.0621738844858676, -0.0554864205922489, -0.043447267221461125, 0.015970313608409187, 0.0015752956234773585, 0.0032109063835089823, 0.006543624386111873, -0.056097848614096384, -0.007921900209639756, 0.029393882015032447, 0.05517093181216938, -0.0005974409591926791, -0.11550882719380107, -0.08725161819463319, -0.07619773269565003, -0.04485559713124112, 0.019560377579083438, -0.009284112323796308, -0.02630185977198872, -0.09050830745381522, -0.04532009405779588, 0.04324730616972267, -0.03314288186141005, -0.07029039853595398, -0.023812426173858883, -0.012097838318380355, -0.05837390686001438, 0.03823981536444931, 0.030912606872874022, -0.059554938903178985, -0.026153282916453902, -0.0929253549018978, -0.18611224378511224, -0.09405291442094861, -0.07984358551913442, -0.09864252549733134, 0.009833374149225645, 0.07983116257623142, 0.06350307964437059, 0.009335208009060807, 0.039772378898988256, 0.03169402042364584, 0.04383097085631169, 0.003950463062753777, -0.044056757200984495, 0.022336036823138204, -0.14096236454621985, -0.09700413118928798, -0.052864178810940264, -0.18961429677533168, -0.04234931888010131, 0.014305429630439409, -0.031216039414959408, -0.08922032705767895, -0.035469866076225084, 0.14491756547697646, 0.14560691258142733, 0.041616979433440705, 0.2300611734366377, 0.1719625840719941, -0.08887615139092415, -0.161203403919816, -0.07591668672985523, -0.05251675078690418, -0.07001278157543954, -0.05642990182716854, -0.13147618404017714, -0.016130572370540424, -0.02312427989828, -0.0399146138224489, -0.15733965423698074, -0.17608592376477414, -0.009978018307030528, -0.13119744342177753, -0.2697469808099955, -0.15045340209128844, -0.11636898052067614, -0.15992601300506407, -0.0854492274312221, -0.027775544783718655, 0.049933615924179296, -0.07571895210554036, -0.11004104613598209, 0.09998565971878416, 0.3310282127293433, 0.11865251014208833, -0.06161897899128249, 0.07575733942713485, -0.03062253812404982, 0.07909742615139889, 0.015637825249847543, -0.03862486224347781, -0.05321954381529302, -0.3941906747738139, -0.224517117206729, 0.21960950139913274, 0.3457693607511479, 0.14753047221691562, -0.27529581090018845, -0.7044003072373299, -0.728755430758407, -0.09133179533357066, 0.10992224387263219, -0.2377953702625985, -0.07405237759468807, -0.056588656013209344, -0.2937956826824701, -0.288403280914405, -0.062409269870219726, -0.09450921017755665, -0.26287249375833743, -0.22899601447091647, -0.1425965543226115, 0.17233714686373505, 0.09907998571240687, -0.24882491725797423, -0.4057981600258323, -0.16294703980179315, 0.1759144774586769, -0.18899575223189471, -0.7392850285299075, -0.7413015482172156, -0.05447265597357274, 0.16491540418383818, -0.2217877375531512, -0.31373361753576134, -0.22084141614644487, -0.07179658425419322, 0.16486503038613814, -0.030233392800509795, -0.49032440164945135, -0.1691709524093597, 0.11636459371207912, -0.0026078983706596254, 0.3209629665888635, 0.018568957616586026, -0.1792159123503127, 0.0836374301067613, -0.1822534161078569, -0.12069770343765551, 0.11619232125306259, -0.4099093691000163, -0.6521852095531759, -0.11624915507321264, -0.09433632083766913, 0.1989002829956384, 0.3633002856749201, -0.01464633788159616, -0.23620176738652152, -0.12501288767780724, 0.03300721427755153, 0.027221415385168122, 0.10670810913936495, 0.05838433118852432, -0.19818366537466053, -0.06866642176618278, -0.1572733726536549, -0.33281490486794535, -0.447170406966975, -0.34121318265188527, 0.28231311876681764, 0.510169292181838, 0.1218998556812824, -0.15600090205785072, 0.11707067700341987, 0.47866020101041, 0.7099033462709033, 0.4071678418634072, 0.0827170731512027, 0.13194772654610157, -0.28328086908230116, -0.5671422955924135, -0.12422944121900566, 0.5830174846937568, 0.3638555341370515, -0.00362808215142391, 0.4240059962729776, 0.0, 0.0, 0.0]] caption="Water Vapor Number Density"
  out "raw counts":dbl[][](graph)=[[16219.5, 58650.5, 70.5, 67.5, 95.5, 184.5, 330.5, 589.5, 785.5, 913.5, 912.5, 982.5, 1074.5, 2283.5, 17690.5, 41023.5, 50013.5, 51542.5, 49176.5, 44809.5, 42448.5, 36019.5, 26981.5, 21378.5, 16798.5, 17359.5, 24672.5, 18550.5, 2062.5, 45.5, -1.5, -2.5, 13.5, 24.5, 4.5, 19.5, 4.5, 0.5, 18.5, -9.5, -6.5, 21.5, -11.5, -1.5, -11.5, 28.5, 13.5, 27.5, 37.5, 14.5, 8.5, -11.5, 27.5, -7.5, 7.5, 19.5, 8.5, -14.5, -18.5, -6.5, 12.5, 3.5, -12.5, 9.5, -5.5, 2.5, 7.5, 2.5, 14.5, -32.5, -25.5, -7.5, 22.5, 2.5, 17.5, 10.5, 11.5, 4.5, -8.5, -17.5, 0.5, -1.5, -11.5, -12.5, 4.5, 22.5, -16.5, -10.5, -8.5, -1.5, 4.5, 0.5, 19.5, 2.5, -21.5, -5.5, 12.5, -12.5, -12.5, -24.5, -3.5, -19.5, -16.5, 1.5, -7.5, -16.5, 2.5, -21.5, 6.5, 15.5, -9.5, 2.5, 10.5, 34.5, 15.5, -1.5, -22.5, 4.5, 25.5, -12.5, 14.5, -30.5, -18.5, -2.5, -13.5, 10.5, -11.5, -26.5, -25.5, 4.5, 11.5, 8.5, 15.5, -12.5, -1.5, -4.5, -5.5, -15.5, -19.5, 22.5, -15.5, -2.5, 14.5, -11.5, 16.5, 28.5, 5.5, -18.5, 15.5, 14.5, 25.5, -3.5, 0.5, -15.5, 18.5, -0.5, -2.5, 10.5, -23.5, -4.5, 6.5, -12.5, 15.5, -7.5, -22.5, -6.5, 30.5, 11.5, 8.5, 4.5, -10.5, -11.5, 13.5, -28.5, 43.5, 0.5, 16.5, 21.5, 14.5, 6.5, 11.5, 17.5, -12.5, -17.5, -32.5, -30.5, -13.5, 9.5, -2.5, -9.5, 7.5, -38.5, 4.5, 19.5, 27.5, 11.5, 25.5, -24.5, 34.5, -5.5, -39.5, 2.5, 58.5, -27.5, -24.5, -2.5, 3.5, 1.5, -8.5, 16.5, -5.5, -12.5, -20.5, 3.5, 23.5, 30.5, 11.5, 9.5, 38.5, 9.5, 8.5, -11.5, 30.5, 24.5, 0.5, -5.5, -6.5, -4.5, 3.5, 31.5, 4.5, 21.5, -4.5, -6.5, 19.5, 14.5, 7.5, -13.5, -25.5, 6.5, 26.5, -0.5, -12.5, -17.5, -9.5, 38.5, -1.5, 2.5, -4.5, 18.5, -6.5, -5.5, 32.5, -6.5, 10.5, -17.5, 13.5, -7.5, -8.5, -27.5, -23.5, -32.5, 3.5, 13.5, 15.5, 29.5, 6.5, 18.5, -10.5, 0.5, -30.5, 19.5, 2.5, -13.5, 13.5, 14.5, 2.5, 7.5, -16.5, 0.0]] caption="Water Vapor Number Density"
  out "raw counts near":dbl[][](graph)=[[14734.3, 54666.3, -19.699999999999818, 26.300000000000182, 3.300000000000182, 38.30000000000018, 35.30000000000018, 93.30000000000018, -8.699999999999818, 92.30000000000018, -7.699999999999818, 8.300000000000182, 3.300000000000182, 81.30000000000018, 1268.3000000000002, 4383.3, 6631.3, 7225.3, 6853.3, 6144.3, 5802.3, 4915.3, 3550.3, 2733.3, 2094.3, 2468.3, 4106.3, 3083.3, 237.30000000000018, -46.69999999999982, -78.69999999999982, -70.69999999999982, -67.69999999999982, 4.300000000000182, -65.69999999999982, 43.30000000000018, -62.69999999999982, -50.69999999999982, -31.699999999999818, -34.69999999999982, -6.699999999999818, -91.69999999999982, -18.699999999999818, -64.69999999999982, -52.69999999999982, 81.30000000000018, -1.699999999999818, 9.300000000000182, 5.300000000000182, -40.69999999999982, -29.699999999999818, -47.69999999999982, -44.69999999999982, -2.699999999999818, 43.30000000000018, 8.300000000000182, -68.69999999999982, 53.30000000000018, -102.69999999999982, -85.69999999999982, -40.69999999999982, -75.69999999999982, -5.699999999999818, -86.69999999999982, -23.699999999999818, 12.300000000000182, 65.30000000000018, -3.699999999999818, 26.300000000000182, 16.300000000000182, -10.699999999999818, -24.699999999999818, -14.699999999999818, -47.69999999999982, -69.69999999999982, -47.69999999999982, 68.30000000000018, -100.69999999999982, 0.3000000000001819, -70.69999999999982, -10.699999999999818, -17.699999999999818, 15.300000000000182, -60.69999999999982, 25.300000000000182, 14.300000000000182, 28.300000000000182, -103.69999999999982, -59.69999999999982, -89.69999999999982, -1.699999999999818, -7.699999999999818, 44.30000000000018, -18.699999999999818, -7.699999999999818, -63.69999999999982, -32.69999999999982, -23.699999999999818, -45.69999999999982, -4.699999999999818, -75.69999999999982, -70.69999999999982, -59.69999999999982, -8.699999999999818, -49.69999999999982, -88.69999999999982, 12.300000000000182, -45.69999999999982, -97.69999999999982, 39.30000000000018, 23.300000000000182, 26.300000000000182, -79.69999999999982, -118.69999999999982, -70.69999999999982, -30.699999999999818, -1.699999999999818, 68.30000000000018, -1.699999999999818, -9.699999999999818, -21.699999999999818, 12.300000000000182, -40.69999999999982, -10.699999999999818, -19.699999999999818, 52.30000000000018, 7.300000000000182, 0.3000000000001819, -1.699999999999818, -78.69999999999982, -122.69999999999982, -75.69999999999982, -45.69999999999982, -118.69999999999982, -62.69999999999982, -33.69999999999982, 0.3000000000001819, 4.300000000000182, 22.300000000000182, -2.699999999999818, -18.699999999999818, -28.699999999999818, -2.699999999999818, 3.300000000000182, -74.69999999999982, -26.699999999999818, 54.30000000000018, -123.69999999999982, 92.30000000000018, -29.699999999999818, -47.69999999999982, 3.300000000000182, -29.699999999999818, -40.69999999999982, -84.69999999999982, 16.300000000000182, 25.300000000000182, 27.300000000000182, 10.300000000000182, -2.699999999999818, 12.300000000000182, -19.699999999999818, -115.69999999999982, -18.699999999999818, -57.69999999999982, -8.699999999999818, -75.69999999999982, -28.699999999999818, -20.699999999999818, -1.699999999999818, -54.69999999999982, -93.69999999999982, -52.69999999999982, 6.300000000000182, -52.69999999999982, -97.69999999999982, -40.69999999999982, -55.69999999999982, 14.300000000000182, -19.699999999999818, 14.300000000000182, 0.3000000000001819, -79.69999999999982, 27.300000000000182, 11.300000000000182, 38.30000000000018, -74.69999999999982, 21.300000000000182, -13.699999999999818, -41.69999999999982, 15.300000000000182, -54.69999999999982, -47.69999999999982, -49.69999999999982, -92.69999999999982, -22.699999999999818, -1.699999999999818, -7.699999999999818, -3.699999999999818, -101.69999999999982, -81.69999999999982, -49.69999999999982, 10.300000000000182, -37.69999999999982, -38.69999999999982, 28.300000000000182, -54.69999999999982, -85.69999999999982, -53.69999999999982, 4.300000000000182, -105.69999999999982, 19.300000000000182, -84.69999999999982, 18.300000000000182, 14.300000000000182, -55.69999999999982, -55.69999999999982, -42.69999999999982, -31.699999999999818, 28.300000000000182, -82.69999999999982, -123.69999999999982, -169.69999999999982, 59.30000000000018, -17.699999999999818, -68.69999999999982, -40.69999999999982, 25.300000000000182, -22.699999999999818, 7.300000000000182, -103.69999999999982, -50.69999999999982, 6.300000000000182, 19.300000000000182, 3.300000000000182, 93.30000000000018, -75.69999999999982, 50.30000000000018, -50.69999999999982, -18.699999999999818, 68.30000000000018, -23.699999999999818, -116.69999999999982, -86.69999999999982, 18.300000000000182, -35.69999999999982, 17.300000000000182, -14.699999999999818, -3.699999999999818, -29.699999999999818, 42.30000000000018, -0.6999999999998181, -44.69999999999982, 30.300000000000182, 24.300000000000182, -49.69999999999982, 3.300000000000182, -61.69999999999982, -11.699999999999818, -48.69999999999982, -35.69999999999982, -27.699999999999818, 20.300000000000182, -32.69999999999982, -56.69999999999982, 68.30000000000018, 60.30000000000018, -9.699999999999818, 31.300000000000182, -25.699999999999818, 14.300000000000182, 12.300000000000182, -36.69999999999982, 11.300000000000182, 60.30000000000018, -82.69999999999982, 59.30000000000018, 36.30000000000018, -48.69999999999982, 0.0]] caption="Water Vapor Number Density"
  out "Aerosol Smoothed 2":dbl[](array[numeric])=[34870.75, 27408.25, 3.5, 3.75, 24.5, 43.0, 77.0, 80.5, 65.25, 48.75, 6.75, 9.0, 38.75, 546.0, 2205.0, 4566.25, 6257.5, 6748.25, 6446.0, 5877.25, 5222.0, 4173.25, 3201.75, 2875.0, 3048.0, 3622.25, 3299.25, 1408.25, 95.25, -47.25, -59.5, -49.25, -19.75, -14.25, 1.5, -13.25, -54.25, -29.5, -3.25, 0.75, -15.75, -9.0, -37.25, -44.5, 0.0, -1.75, -11.75, 3.75, -21.5, -37.25, -19.5, -11.0, -16.75, -14.75, -6.75, -25.25, 3.5, -17.75, -60.25, -46.25, -36.5, 5.25, -18.75, -35.5, 3.75, 9.0, 28.5, 49.75, 30.0, 8.5, -14.25, -46.0, -46.25, -36.75, -26.25, 3.75, -13.5, -45.5, -51.75, -42.25, -27.5, -18.5, -9.25, -9.0, 13.5, 20.25, -21.75, -50.25, -32.25, -20.75, 1.25, 15.5, -12.5, -24.75, -23.0, -24.5, -31.5, -55.5, -32.0, -21.5, -32.0, -28.0, -21.5, 7.75, 0.75, 1.5, 3.0, -25.25, -3.5, 12.75, 23.5, -0.25, -47.5, -35.25, -30.25, -17.5, 7.5, -3.5, -9.75, -33.0, -16.25, 15.25, -11.5, -24.0, -8.0, -4.0, -19.0, 12.25, 9.75, -18.5, -8.0, -28.0, -55.25, -27.5, -23.0, -28.0, 2.75, 22.0, 17.25, 2.5, 10.5, 8.25, 11.25, 1.0, -11.0, 5.5, -34.25, -23.25, -12.5, -44.25, -9.75, 3.25, -7.0, -19.75, -7.75, 31.25, 31.0, 8.75, 47.75, 35.25, -18.0, -32.25, -15.0, -10.25, -13.5, -10.75, -24.75, -3.0, -4.25, -7.25, -28.25, -31.25, -1.75, -22.75, -46.25, -25.5, -19.5, -26.5, -14.0, -4.5, 8.0, -12.0, -17.25, 15.5, 50.75, 18.0, -9.25, 11.25, -4.5, 11.5, 2.25, -5.5, -7.5, -55.0, -31.0, 30.0, 46.75, 19.75, -36.5, -92.5, -94.75, -11.75, 14.0, -30.0, -9.25, -7.0, -36.0, -35.0, -7.5, -11.25, -31.0, -26.75, -16.5, 19.75, 11.25, -28.0, -45.25, -18.0, 19.25, -20.5, -79.5, -79.0, -5.75, 17.25, -23.0, -32.25, -22.5, -7.25, 16.5, -3.0, -48.25, -16.5, 11.25, -0.25, 30.5, 1.75, -16.75, 7.75, -16.75, -11.0, 10.5, -36.75, -58.0, -10.25, -8.25, 17.25, 31.25, -1.25, -20.0, -10.5, 2.75, 2.25, 8.75, 4.75, -16.0, -5.5, -12.5, -26.25, -35.0, -26.5, 21.75, 39.0, 9.25, -11.75, 8.75, 35.5, 52.25, 29.75, 6.0, 9.5, -20.25, -40.25, -8.75, 40.75, 25.25, -0.25, 29.0]
  out "Off-Line Smoothed 2":dbl[](array[numeric])=[34722.059832635976, 27387.011715481163, 1.1414225941422613, 3.9761506276150644, 14.497071129707113, 23.70418410041841, 32.783682008368196, 36.51171548117155, 38.804602510460256, 45.254393305439336, 65.00753138075316, 98.90920502092057, 149.83807531380756, 289.2606694560668, 711.7062761506274, 1412.2355648535572, 2049.0179916318, 2399.231380753138, 2696.1330543933054, 3255.471966527196, 4027.992887029287, 4863.963598326357, 5577.482426778241, 6068.105857740584, 5915.072384937235, 4583.29832635983, 2636.2899581589954, 999.5661087866114, 166.68953974895382, -9.166108786610879, -17.398326359832637, -15.74769874476987, -15.620083682008365, -15.862761506276147, -16.08870292887029, -18.33765690376569, -20.992468619246864, -19.502928870292884, -18.93389121338912, -19.47154811715481, -18.49037656903765, -18.973640167364017, -17.233054393305437, -14.875313807531377, -16.009205020920497, -19.467364016736397, -22.71213389121339, -21.189121338912134, -17.64728033472803, -15.10962343096234, -15.14728033472803, -13.207949790794977, -10.779079497907947, -9.940167364016734, -11.268619246861922, -17.427615062761507, -18.406694560669457, -18.128451882845187, -16.55523012552301, -16.166108786610877, -16.875313807531377, -15.291631799163177, -15.094979079497906, -13.17238493723849, -13.381589958158994, -12.919246861924684, -12.65983263598326, -15.13054393305439, -14.10962343096234, -12.314644351464432, -13.335564853556482, -16.25397489539749, -18.92761506276151, -15.38786610878661, -10.230962343096234, -13.77071129707113, -13.638912133891214, -10.061506276150626, -16.82510460251046, -15.348117154811717, -9.276987447698744, -8.11380753138075, -8.699581589958157, -14.450627615062757, -16.05941422594142, -13.50502092050209, -13.864853556485354, -13.760251046025102, -13.898326359832634, -13.400418410041839, -12.846025104602507, -13.490376569037654, -12.04267782426778, -10.843933054393304, -11.228870292887027, -13.329288702928867, -11.57196652719665, -11.927615062761504, -15.383682008368199, -15.860669456066944, -12.71004184100418, -8.733054393305437, -8.203765690376567, -10.350209205020917, -12.27280334728033, -10.927615062761504, -7.695397489539747, -7.318828451882844, -10.965271966527194, -13.320920502092047, -14.96317991631799, -13.11799163179916, -11.01757322175732, -10.779079497907947, -11.337656903765689, -10.07196652719665, -7.651464435146442, -11.01757322175732, -9.120083682008365, -5.458995815899581, -9.015481171548116, -9.210041841004182, -7.310460251046024, -9.756066945606694, -9.789539748953974, -9.10543933054393, -9.61380753138075, -10.58451882845188, -10.371129707112969, -5.816736401673639, -9.136820083682007, -12.04686192468619, -7.651464435146442, -7.327196652719664, -5.791631799163179, -4.722594142259412, -7.875313807531379, -8.5092050209205, -7.0761506276150605, -9.103347280334726, -11.51757322175732, -9.128451882845185, -7.929707112970709, -8.308368200836819, -6.084518828451881, -5.486192468619246, -5.691213389121337, -4.509205020920501, -5.827196652719664, -8.664016736401672, -8.237238493723847, -8.91715481171548, -8.998744769874476, -8.469456066945604, -6.823012552301253, -4.764435146443513, -5.452719665271965, -7.172384937238491, -6.5970711297071105, -2.6828451882845172, -3.785355648535563, -4.680753138075312, -3.0531380753138055, -2.343933054393304, -5.40041841004184, -6.837656903765689, -4.346025104602509, -4.153556485355647, -3.469456066945605, -3.4004184100418393, -7.379497907949789, -9.394142259414224, -5.45062761506276, -3.808368200836818, -5.339748953974894, -5.0573221757322155, -6.000836820083681, -5.617991631799161, -4.151464435146442, -3.9548117154811697, -0.5824267782426762, 0.7146443514644368, -1.4527196652719647, 1.0451882845188303, 0.5033472803347299, -5.247698744769872, -6.239330543933052, -5.670292887029287, -2.7916317991631785, -2.538493723849371, -3.561506276150626, -3.2518828451882826, -4.921338912133889, -5.634728033472801, -3.5405857740585756, -2.9338912133891197, -5.661924686192467, -5.0510460251046005, -3.49246861924686, -8.132635983263595, -8.519665271966524, -1.4129707112970693, -0.23723849372384775, -2.764435146443513, -2.563598326359831, -1.799999999999998, -4.412970711297069, -4.189121338912132, -4.603347280334726, -6.237238493723847, -1.9297071129707095, 1.635146443514646, -0.8313807531380737, -2.3167364016736385, -0.4234309623430945, -0.3146443514644334, -3.4757322175732197, -5.130543933054391, -6.03012552301255, -4.753974895397487, -2.9192468619246847, -2.3920502092050193, -2.50502092050209, -6.174476987447697, -4.979916317991631, -4.230962343096232, -4.354393305439329, -0.8188284518828436, -2.4548117154811697, -3.9987447698744756, 0.4698744769874492, 0.8987447698744786, -1.7560669456066929, -3.9757322175732197, -4.519665271966526, -4.772803347280333, -5.274895397489538, -5.519665271966526, -5.927615062761504, -3.9317991631799147, -2.841841004184099, -1.9192468619246845, -1.5426778242677806, 2.283682008368203, 1.0619246861924703, -2.4276150627615047, -1.6179916317991614, -1.8125523012552285, -2.8857740585774043, -1.8941422594142243, 2.3903765690376586, -0.3125523012552285, -6.197489539748952, -5.5364016736401656, -2.076150627615061, 1.0138075313807549, -1.561506276150626, -7.287447698744768, -6.283263598326358, -2.1263598326359814, -1.2539748953974879, -3.634728033472802, -2.785355648535563, 0.6769874476987465, 2.5786610878661103, 1.8108786610878678, -1.2058577405857724, -0.7539748953974879, 1.4071129707112988, 2.9970711297071144, 4.775313807531383, 0.04100418410041984, -5.312552301255229, -2.586610878661086, 2.9635983263598344, -0.3753138075313789, -2.4631799163179897]
  out "Off-Line Bin Readings 2":dbl[](array[numeric])=[16870.0, 56802.0, 2116.0, 2162.0, 2139.0, 2174.0, 2171.0, 2229.0, 2127.0, 2228.0, 2128.0, 2144.0, 2139.0, 2217.0, 3404.0, 6519.0, 8767.0, 9361.0, 8989.0, 8280.0, 7938.0, 7051.0, 5686.0, 4869.0, 4230.0, 4604.0, 6242.0, 5219.0, 2373.0, 2089.0, 2057.0, 2065.0, 2068.0, 2140.0, 2070.0, 2179.0, 2073.0, 2085.0, 2104.0, 2101.0, 2129.0, 2044.0, 2117.0, 2071.0, 2083.0, 2217.0, 2134.0, 2145.0, 2141.0, 2095.0, 2106.0, 2088.0, 2091.0, 2133.0, 2179.0, 2144.0, 2067.0, 2189.0, 2033.0, 2050.0, 2095.0, 2060.0, 2130.0, 2049.0, 2112.0, 2148.0, 2201.0, 2132.0, 2162.0, 2152.0, 2125.0, 2111.0, 2121.0, 2088.0, 2066.0, 2088.0, 2204.0, 2035.0, 2136.0, 2065.0, 2125.0, 2118.0, 2151.0, 2075.0, 2161.0, 2150.0, 2164.0, 2032.0, 2076.0, 2046.0, 2134.0, 2128.0, 2180.0, 2117.0, 2128.0, 2072.0, 2103.0, 2112.0, 2090.0, 2131.0, 2060.0, 2065.0, 2076.0, 2127.0, 2086.0, 2047.0, 2148.0, 2090.0, 2038.0, 2175.0, 2159.0, 2162.0, 2056.0, 2017.0, 2065.0, 2105.0, 2134.0, 2204.0, 2134.0, 2126.0, 2114.0, 2148.0, 2095.0, 2125.0, 2116.0, 2188.0, 2143.0, 2136.0, 2134.0, 2057.0, 2013.0, 2060.0, 2090.0, 2017.0, 2073.0, 2102.0, 2136.0, 2140.0, 2158.0, 2133.0, 2117.0, 2107.0, 2133.0, 2139.0, 2061.0, 2109.0, 2190.0, 2012.0, 2228.0, 2106.0, 2088.0, 2139.0, 2106.0, 2095.0, 2051.0, 2152.0, 2161.0, 2163.0, 2146.0, 2133.0, 2148.0, 2116.0, 2020.0, 2117.0, 2078.0, 2127.0, 2060.0, 2107.0, 2115.0, 2134.0, 2081.0, 2042.0, 2083.0, 2142.0, 2083.0, 2038.0, 2095.0, 2080.0, 2150.0, 2116.0, 2150.0, 2136.0, 2056.0, 2163.0, 2147.0, 2174.0, 2061.0, 2157.0, 2122.0, 2094.0, 2151.0, 2081.0, 2088.0, 2086.0, 2043.0, 2113.0, 2134.0, 2128.0, 2132.0, 2034.0, 2054.0, 2086.0, 2146.0, 2098.0, 2097.0, 2164.0, 2081.0, 2050.0, 2082.0, 2140.0, 2030.0, 2155.0, 2051.0, 2154.0, 2150.0, 2080.0, 2080.0, 2093.0, 2104.0, 2164.0, 2053.0, 2012.0, 1966.0, 2195.0, 2118.0, 2067.0, 2095.0, 2161.0, 2113.0, 2143.0, 2032.0, 2085.0, 2142.0, 2155.0, 2139.0, 2229.0, 2060.0, 2186.0, 2085.0, 2117.0, 2204.0, 2112.0, 2019.0, 2049.0, 2154.0, 2100.0, 2153.0, 2121.0, 2132.0, 2106.0, 2178.0, 2135.0, 2091.0, 2166.0, 2160.0, 2086.0, 2139.0, 2074.0, 2124.0, 2087.0, 2100.0, 2108.0, 2156.0, 2103.0, 2079.0, 2204.0, 2196.0, 2126.0, 2167.0, 2110.0, 2150.0, 2148.0, 2099.0, 2147.0, 2196.0, 2053.0, 2195.0, 2172.0, 2087.0]
  out "On-Line Smoothed 2":dbl[](array[numeric])=[34971.88117154811, 27711.998326359826, -3.6062761506276173, 0.5234309623430939, 7.62175732217573, 10.498326359832634, 14.998326359832635, 17.086192468619238, 21.006694560669445, 25.76192468619246, 32.89163179916319, 50.20125523012554, 76.79330543933054, 145.38744769874472, 353.25355648535555, 688.4523012552303, 972.845606694561, 1102.5589958158996, 1195.9481171548116, 1396.6552301255233, 1681.749372384938, 1971.1991631799167, 2173.950209205021, 2266.351882845189, 2118.525523012553, 1569.7514644351468, 858.7974895397488, 304.8330543933054, 37.2305439330544, -14.026778242677826, -16.388702928870295, -20.480753138075315, -20.235983263598328, -19.411715481171548, -17.04560669456067, -14.449372384937242, -13.673221757322178, -12.292468619246865, -12.88242677824268, -15.823849372384938, -18.905439330543935, -16.505857740585775, -17.068619246861925, -17.623012552301255, -16.773640167364018, -18.365690376569034, -14.725523012552301, -14.528870292887033, -17.39288702928871, -17.551882845188285, -14.522594142259415, -12.089539748953978, -16.415899581589958, -16.99958158995816, -15.037238493723851, -17.648117154811715, -19.369874476987448, -18.93682008368201, -18.07071129707113, -17.48075313807531, -15.702510460251046, -13.934728033472805, -16.36150627615063, -15.110460251046028, -12.610460251046028, -13.589539748953978, -15.005857740585776, -16.361506276150628, -14.392887029288705, -13.805020920502095, -14.240167364016738, -13.964016736401675, -13.648117154811718, -15.371966527196655, -15.072803347280336, -13.411715481171552, -14.980753138075316, -14.930543933054395, -13.016317991631801, -13.526778242677826, -13.654393305439331, -13.192050209205023, -13.043514644351468, -8.681589958158998, -8.595815899581591, -11.409623430962345, -11.426359832635987, -12.894979079497912, -11.999581589958161, -10.447280334728035, -10.173221757322178, -10.505857740585776, -11.756903765690378, -9.131380753138078, -8.89497907949791, -6.380334728033475, -4.576987447698746, -8.286192468619248, -8.38242677824268, -11.792468619246865, -14.026778242677826, -11.068619246861926, -9.143933054393308, -9.566527196652721, -8.26945606694561, -7.41589958158996, -11.438912133891215, -13.248535564853558, -11.246443514644355, -13.786192468619248, -15.363598326359833, -12.035146443514648, -8.635564853556488, -7.29874476987448, -8.169037656903768, -8.970292887029292, -9.953556485355652, -7.901255230125525, -5.876150627615065, -4.428451882845191, -8.677405857740588, -9.225523012552303, -7.166945606694563, -8.489121338912136, -8.692050209205023, -9.217154811715485, -9.31966527196653, -11.758995815899585, -13.447280334728035, -9.85732217573222, -5.110460251046027, -6.834309623430965, -9.401255230125525, -6.805020920502095, -4.240167364016738, -8.880334728033475, -8.938912133891215, -6.9995815899581615, -7.920083682008371, -7.899163179916321, -7.9682008368200865, -9.30292887029289, -9.292468619246865, -6.758995815899584, -8.217154811715483, -9.671129707112973, -8.227615062761508, -5.771548117154814, -7.28200836820084, -8.076987447698748, -8.430543933054395, -9.968200836820085, -9.802928870292888, -5.763179916317994, -3.464016736401676, -7.114644351464438, -8.767364016736405, -4.830125523012554, -0.7903765690376592, -6.422175732217576, -9.738075313807533, -5.765271966527199, -7.5267782426778265, -8.809205020920505, -5.685774058577408, -5.28200836820084, -4.5560669456066964, -4.235983263598328, -6.231799163179918, -6.217154811715483, -3.4096234309623457, -6.9723849372384965, -9.480753138075316, -6.34058577405858, -6.4933054393305465, -6.9682008368200865, -5.88661087866109, -5.9870292887029315, -6.712970711297073, -5.0602510460251064, -3.8845188284518852, -3.9430962343096256, -4.0518828451882865, -3.1418410041841023, -3.4347280334728056, -3.4702928870292915, -6.212970711297073, -8.941004184100422, -7.834309623430965, -7.78200836820084, -5.620920502092053, -4.325941422594145, -7.42008368200837, -8.367782426778245, -4.86569037656904, -5.388702928870295, -4.625104602510462, -3.6000000000000023, -4.0100418410041865, -4.5435146443514665, -5.445188284518831, -3.049790794979082, -1.549790794979082, -1.2213389121338936, -3.666945606694563, -7.185774058577408, -6.187866108786613, -3.5769874476987473, -5.0184100418410065, -3.32384937238494, -1.2945606694560692, -3.271548117154814, -3.8489539748954, -4.742259414225944, -2.275732217573224, -1.8510460251046046, -5.704602510460253, -4.177405857740588, -1.8092050209205044, -0.2966527196652743, -1.1104602510460273, -0.15230125523012772, 0.23682008368200602, -0.43682008368201064, 0.04016736401673415, -1.0205020920502115, -3.9493723849372406, -6.443096234309626, -4.181589958158998, -5.252719665271969, -4.717154811715483, -2.834309623430965, -3.4368200836820106, -0.8866108786610901, -2.1104602510460273, -2.284100418410044, 0.8518828451882823, -0.4912133891213412, -2.2108786610878686, -4.635564853556488, -2.9974895397489565, -3.4933054393305465, -4.31548117154812, -2.551882845188287, -4.658577405857743, -3.6564853556485377, -3.7569037656903785, -4.5560669456066964, -2.830125523012555, -1.7966527196652744, -4.411715481171551, -3.342677824267785, -0.16276150627615288, -0.8468619246861947, 0.9313807531380731, 1.2912133891213367, 1.1949790794979056, 0.4125523012552278, -2.851046025104605, -3.1481171548117177, -3.0372384937238515, -2.1251046025104623, -0.8301255230125546, -0.035146443514646575, -1.7966527196652744, -6.0539748953974915, -2.4514644351464456, 4.15523012552301, 3.3456066945606673, 0.9836820083681985, 1.1740585774058556, 1.6573221757322152, -0.267364016736404, -1.480753138075316, -0.5121338912133915, 0.6573221757322153, 0.28075313807531155]
  out "On-Line Bin Readings 2":dbl[](array[numeric])=[17219.0, 57790.0, 2182.0, 2091.0, 2180.0, 2175.0, 2207.0, 2176.0, 2087.0, 2209.0, 2192.0, 2127.0, 2072.0, 2137.0, 2821.0, 4264.0, 5283.0, 5554.0, 5275.0, 5009.0, 4689.0, 4098.0, 3427.0, 3181.0, 2837.0, 2962.0, 3611.0, 3028.0, 2212.0, 2105.0, 2132.0, 2105.0, 2149.0, 2117.0, 2091.0, 2128.0, 2135.0, 2123.0, 2183.0, 2110.0, 2129.0, 2120.0, 2176.0, 2124.0, 2119.0, 2101.0, 2000.0, 2126.0, 2001.0, 2192.0, 2091.0, 2243.0, 2071.0, 2138.0, 2155.0, 2068.0, 2080.0, 2098.0, 2126.0, 2052.0, 2120.0, 2136.0, 2115.0, 2171.0, 2143.0, 2211.0, 2132.0, 2127.0, 2125.0, 2125.0, 2105.0, 2074.0, 2155.0, 2043.0, 2214.0, 2075.0, 2157.0, 2070.0, 2035.0, 2102.0, 2129.0, 2154.0, 2197.0, 2125.0, 2124.0, 2159.0, 2040.0, 2178.0, 2104.0, 2166.0, 2077.0, 2004.0, 2115.0, 2135.0, 2052.0, 2039.0, 2159.0, 2110.0, 2122.0, 2159.0, 2118.0, 2171.0, 2144.0, 2046.0, 2251.0, 2080.0, 2150.0, 2144.0, 2043.0, 2035.0, 2174.0, 2223.0, 2090.0, 2153.0, 2076.0, 2151.0, 2093.0, 2165.0, 2118.0, 2180.0, 2101.0, 2085.0, 2171.0, 2117.0, 2060.0, 2270.0, 2141.0, 2145.0, 2149.0, 2139.0, 2135.0, 2053.0, 2127.0, 2130.0, 2096.0, 2115.0, 2095.0, 2141.0, 2091.0, 2078.0, 2126.0, 2141.0, 2115.0, 2071.0, 2156.0, 2085.0, 2128.0, 2108.0, 2131.0, 2029.0, 2159.0, 2082.0, 2077.0, 2160.0, 2127.0, 2141.0, 2148.0, 2138.0, 2120.0, 2130.0, 2114.0, 2115.0, 2113.0, 2026.0, 2192.0, 2142.0, 2148.0, 2172.0, 2137.0, 2080.0, 2155.0, 2226.0, 2150.0, 2130.0, 2089.0, 2146.0, 2082.0, 2093.0, 2045.0, 2114.0, 2066.0, 2101.0, 2058.0, 2180.0, 2248.0, 2198.0, 2190.0, 2098.0, 2184.0, 2077.0, 2124.0, 2080.0, 2093.0, 2027.0, 2105.0, 2068.0, 2077.0, 2137.0, 2200.0, 2157.0, 2025.0, 2077.0, 2172.0, 2187.0, 2104.0, 2081.0, 2136.0, 2155.0, 2106.0, 2136.0, 2125.0, 2191.0, 2124.0, 2145.0, 2135.0, 2176.0, 2142.0, 2051.0, 2210.0, 2104.0, 2085.0, 2114.0, 2167.0, 2057.0, 2123.0, 2094.0, 2122.0, 2103.0, 2212.0, 2175.0, 2161.0, 2067.0, 2107.0, 2039.0, 2126.0, 2113.0, 2131.0, 2280.0, 2087.0, 2069.0, 2115.0, 2134.0, 2101.0, 2085.0, 2155.0, 2168.0, 2224.0, 2087.0, 2108.0, 2065.0, 2039.0, 2071.0, 2050.0, 2178.0, 2087.0, 2180.0, 2045.0, 2067.0, 2146.0, 2171.0, 2122.0, 2134.0, 2186.0, 2201.0, 2161.0, 2150.0, 2144.0, 2060.0, 2050.0, 2130.0, 2103.0, 2144.0, 2153.0, 2086.0, 2203.0, 2122.0, 2041.0, 2103.0, 2140.0]
  in  "stop":bool
  in  "Reset Average":bool=TRUE
  in  "Save Data?":bool=TRUE
  in  "Collect Data?":bool=TRUE
  in  "ILX Address":i32=6 min=0 step=1
  in  "Lambda On DBR Current":dbl=158.08
  in  "Lambda Off DBR Current":dbl=160.0
  in  "Tab Control":T2(tab)=enum."OD"
  out "Water Vapor Number Density  2":cluster{"Y":dbl[], "Y":dbl[]}[](graph)
  out "Absolute Humidity":cluster{"Y":dbl[], "Y":dbl[]}[](graph)
  out "NRB plot":cluster{"Y":dbl[], "Y":dbl[]}[](graph)
  in  "background length":i32=10
  out "Correction":cluster{"Y":dbl[], "Y":dbl[]}[](graph)
  in  "dead time":dbl=3.7e-08
  out "Optical Depth":cluster{"Y":dbl[], "Y":dbl[]}[](graph) caption="XY Graph"
  out "RingBuffer offline far":dbl[][](array[numeric])
  out "RingBuffer aerosol far":dbl[][](array[numeric])=[[16219.5, 58650.5, 70.5, 67.5, 95.5, 184.5, 330.5, 589.5, 785.5, 913.5, 912.5, 982.5, 1074.5, 2283.5, 17690.5, 41023.5, 50013.5, 51542.5, 49176.5, 44809.5, 42448.5, 36019.5, 26981.5, 21378.5, 16798.5, 17359.5, 24672.5, 18550.5, 2062.5, 45.5, -1.5, -2.5, 13.5, 24.5, 4.5, 19.5, 4.5, 0.5, 18.5, -9.5, -6.5, 21.5, -11.5, -1.5, -11.5, 28.5, 13.5, 27.5, 37.5, 14.5, 8.5, -11.5, 27.5, -7.5, 7.5, 19.5, 8.5, -14.5, -18.5, -6.5, 12.5, 3.5, -12.5, 9.5, -5.5, 2.5, 7.5, 2.5, 14.5, -32.5, -25.5, -7.5, 22.5, 2.5, 17.5, 10.5, 11.5, 4.5, -8.5, -17.5, 0.5, -1.5, -11.5, -12.5, 4.5, 22.5, -16.5, -10.5, -8.5, -1.5, 4.5, 0.5, 19.5, 2.5, -21.5, -5.5, 12.5, -12.5, -12.5, -24.5, -3.5, -19.5, -16.5, 1.5, -7.5, -16.5, 2.5, -21.5, 6.5, 15.5, -9.5, 2.5, 10.5, 34.5, 15.5, -1.5, -22.5, 4.5, 25.5, -12.5, 14.5, -30.5, -18.5, -2.5, -13.5, 10.5, -11.5, -26.5, -25.5, 4.5, 11.5, 8.5, 15.5, -12.5, -1.5, -4.5, -5.5, -15.5, -19.5, 22.5, -15.5, -2.5, 14.5, -11.5, 16.5, 28.5, 5.5, -18.5, 15.5, 14.5, 25.5, -3.5, 0.5, -15.5, 18.5, -0.5, -2.5, 10.5, -23.5, -4.5, 6.5, -12.5, 15.5, -7.5, -22.5, -6.5, 30.5, 11.5, 8.5, 4.5, -10.5, -11.5, 13.5, -28.5, 43.5, 0.5, 16.5, 21.5, 14.5, 6.5, 11.5, 17.5, -12.5, -17.5, -32.5, -30.5, -13.5, 9.5, -2.5, -9.5, 7.5, -38.5, 4.5, 19.5, 27.5, 11.5, 25.5, -24.5, 34.5, -5.5, -39.5, 2.5, 58.5, -27.5, -24.5, -2.5, 3.5, 1.5, -8.5, 16.5, -5.5, -12.5, -20.5, 3.5, 23.5, 30.5, 11.5, 9.5, 38.5, 9.5, 8.5, -11.5, 30.5, 24.5, 0.5, -5.5, -6.5, -4.5, 3.5, 31.5, 4.5, 21.5, -4.5, -6.5, 19.5, 14.5, 7.5, -13.5, -25.5, 6.5, 26.5, -0.5, -12.5, -17.5, -9.5, 38.5, -1.5, 2.5, -4.5, 18.5, -6.5, -5.5, 32.5, -6.5, 10.5, -17.5, 13.5, -7.5, -8.5, -27.5, -23.5, -32.5, 3.5, 13.5, 15.5, 29.5, 6.5, 18.5, -10.5, 0.5, -30.5, 19.5, 2.5, -13.5, 13.5, 14.5, 2.5, 7.5, -16.5], [16628.0, 58873.0, 63.0, 96.0, 70.0, 217.0, 400.0, 580.0, 930.0, 919.0, 964.0, 972.0, 1024.0, 2357.0, 12044.0, 27782.0, 43023.0, 49336.0, 49327.0, 45523.0, 40639.0, 35812.0, 28256.0, 23674.0, 25407.0, 26388.0, 23473.0, 13118.0, 1238.0, 2.0, -4.0, -5.0, 12.0, -15.0, 9.0, -4.0, -28.0, 15.0, -20.0, -5.0, -22.0, 42.0, 3.0, 23.0, -16.0, 5.0, -22.0, -16.0, 7.0, -46.0, -12.0, 22.0, 1.0, -28.0, 13.0, 3.0, 10.0, -11.0, -10.0, 17.0, 3.0, 30.0, -4.0, 29.0, -4.0, -1.0, 18.0, -17.0, -4.0, -11.0, 17.0, -9.0, 7.0, 17.0, -14.0, 23.0, -22.0, -6.0, 5.0, 10.0, -6.0, -32.0, 1.0, 1.0, 42.0, -21.0, -19.0, -34.0, -9.0, 0.0, -2.0, -37.0, 1.0, 14.0, 11.0, 13.0, 10.0, 11.0, 5.0, -15.0, -21.0, -6.0, 1.0, -1.0, 7.0, 4.0, -20.0, -5.0, -4.0, -3.0, -1.0, 9.0, -8.0, -16.0, -8.0, -1.0, 7.0, 8.0, -4.0, 27.0, 5.0, -9.0, -3.0, -18.0, -15.0, -2.0, -20.0, 23.0, 7.0, -14.0, 29.0, -4.0, 7.0, 21.0, 5.0, -3.0, 6.0, 8.0, 11.0, 5.0, -2.0, 6.0, -6.0, -15.0, -3.0, -8.0, 25.0, 27.0, -4.0, -46.0, 0.0, 3.0, -19.0, 5.0, 38.0, -21.0, -6.0, -12.0, 4.0, -25.0, 9.0, -2.0, 20.0, 14.0, -15.0, -18.0, 12.0, -13.0, 20.0, -20.0, 33.0, -17.0, 0.0, -28.0, 10.0, 9.0, -9.0, -3.0, 9.0, -7.0, 30.0, -25.0, 0.0, 8.0, 26.0, -7.0, 3.0, -9.0, -13.0, -1.0, 16.0, 15.0, -3.0, -15.0, 34.0, -34.0, -11.0, -30.0, -10.0, -2.0, -40.0, -10.0, -19.0, 18.0, -24.0, -6.0, -6.0, 11.0, 29.0, -15.0, -14.0, 23.0, -2.0, -27.0, 10.0, 2.0, -4.0, 9.0, 2.0, -13.0, 24.0, 11.0, -9.0, 1.0, 2.0, 4.0, -2.0, 2.0, -12.0, 12.0, 10.0, -24.0, 0.0, -26.0, -12.0, 21.0, 25.0, -5.0, 5.0, 5.0, 11.0, -10.0, 11.0, -26.0, -9.0, -9.0, -12.0, -4.0, 14.0, 19.0, 3.0, -5.0, 28.0, 6.0, -1.0, 23.0, -11.0, 11.0, -14.0, 27.0, 0.0, -12.0, 15.0, -1.0, -21.0, -15.0, 9.0, -14.0, 10.0, -6.0, -3.0, -9.0, -9.0, 26.0, -2.0, 11.0, 9.0, -17.0, 0.0]]
  in  "Weather":T3(tab)=enum."Pulse Energy (Micro Joule)"
  in  "Temperature (C)":dbl=15.0
  out "Temperature (C)":dbl(graph)=15.0
  in  "Pressure (mbar or hPa)":dbl=832.0
  out "Pressure (mb)":dbl(graph)=832.0
  out "Relative Humdity (%)":dbl(graph)=40.0
  out "Pulse Energy (Micro Joule)":T4(graph)
  in  "PRF (kHz)":dbl=7.0
  out "?":cluster{"mean":dbl, "mean":dbl}(graph)={"mean"=53100.0, "mean"=427139.99999999994}
  out "Index":i32=438
  out "Aerosol Smoothed":dbl[](array[numeric])=[37592.75, 29414.25, 74.25, 82.25, 141.75, 283.0, 475.0, 721.25, 887.0, 927.25, 957.75, 1013.25, 1684.75, 8593.75, 24635.0, 40460.5, 48478.75, 49845.5, 47209.0, 43355.0, 38729.75, 31767.25, 25072.5, 21814.5, 21488.25, 22973.25, 19953.5, 8742.25, 837.0, 10.5, -3.25, 4.5, 8.75, 5.75, 7.25, -2.0, -2.0, 3.5, -4.0, -10.75, 8.75, 13.75, 3.25, -1.5, 1.5, 6.25, 0.75, 14.0, 3.25, -8.75, 1.75, 9.75, -1.75, -3.75, 10.75, 10.25, -1.75, -13.5, -4.5, 6.5, 12.25, 4.25, 5.5, 7.25, -2.0, 6.75, 2.75, -1.0, -8.25, -13.0, -6.25, 3.25, 12.25, 5.75, 9.25, 5.75, -3.0, -1.25, -2.75, -3.25, -9.75, -11.0, -5.5, 8.75, 12.0, -8.5, -20.0, -15.5, -4.75, 0.25, -8.5, -4.0, 9.25, 1.5, -0.75, 7.5, 5.25, -2.25, -11.75, -16.0, -12.5, -10.25, -3.75, 0.0, -3.25, -7.5, -11.0, -6.0, 3.75, 0.5, 0.25, 3.5, 5.25, 6.5, 1.25, -4.5, -0.75, 8.5, 9.0, 8.5, -5.0, -15.25, -10.5, -12.25, -5.0, -5.75, -8.75, -5.5, -7.0, 7.75, 11.25, 6.75, 7.75, 3.0, -1.0, -1.75, -1.75, -4.0, 4.75, 2.5, -3.5, 3.0, -4.5, -3.25, 8.5, 12.75, 9.75, 5.0, -5.0, -1.5, 6.25, -4.75, -7.25, 11.5, 8.75, -7.5, -2.5, -5.25, -12.25, -3.5, 0.25, 5.25, 10.5, -7.75, -15.5, 4.5, 10.25, 6.75, 3.25, 1.75, -1.5, -3.75, -10.75, -0.75, 15.75, 4.25, 6.5, 10.5, 5.75, 10.25, 8.5, -5.0, -5.5, -4.0, -11.0, -12.0, -2.5, -3.75, -6.5, 3.25, 0.0, -5.5, 1.5, 16.5, 9.75, -2.0, -10.0, -7.5, 4.25, -21.75, -21.75, 8.0, 7.5, -14.5, -14.25, -2.75, 2.5, 8.25, 5.5, -4.5, -2.25, -3.0, -11.5, 2.5, 16.5, 10.0, 6.5, 14.75, 9.25, 7.25, 8.0, 5.25, 11.75, 7.0, 0.25, -2.5, -2.75, -2.75, 8.75, 14.5, 3.0, -1.75, -9.25, -6.25, 10.75, 17.0, 3.5, -9.75, -2.25, 12.25, 6.75, -3.0, -11.25, -15.5, 2.75, 4.0, -3.75, 2.0, 11.75, 8.5, -3.5, 12.5, 15.0, 2.25, 3.75, 2.0, 1.5, -4.75, -5.75, -6.0, -17.0, -6.5, 7.75, 1.75, 2.25, 7.5, 5.0, 1.0, -1.5, -9.75, -5.75, 1.0, 1.5, 6.0, 9.25, 9.25, 0.5]
  out "Off-Line  Bin Readings":dbl[](array[numeric])=[16485.0, 58916.0, 336.0, 333.0, 361.0, 450.0, 596.0, 855.0, 1051.0, 1179.0, 1178.0, 1248.0, 1340.0, 2549.0, 17956.0, 41289.0, 50279.0, 51808.0, 49442.0, 45075.0, 42714.0, 36285.0, 27247.0, 21644.0, 17064.0, 17625.0, 24938.0, 18816.0, 2328.0, 311.0, 264.0, 263.0, 279.0, 290.0, 270.0, 285.0, 270.0, 266.0, 284.0, 256.0, 259.0, 287.0, 254.0, 264.0, 254.0, 294.0, 279.0, 293.0, 303.0, 280.0, 274.0, 254.0, 293.0, 258.0, 273.0, 285.0, 274.0, 251.0, 247.0, 259.0, 278.0, 269.0, 253.0, 275.0, 260.0, 268.0, 273.0, 268.0, 280.0, 233.0, 240.0, 258.0, 288.0, 268.0, 283.0, 276.0, 277.0, 270.0, 257.0, 248.0, 266.0, 264.0, 254.0, 253.0, 270.0, 288.0, 249.0, 255.0, 257.0, 264.0, 270.0, 266.0, 285.0, 268.0, 244.0, 260.0, 278.0, 253.0, 253.0, 241.0, 262.0, 246.0, 249.0, 267.0, 258.0, 249.0, 268.0, 244.0, 272.0, 281.0, 256.0, 268.0, 276.0, 300.0, 281.0, 264.0, 243.0, 270.0, 291.0, 253.0, 280.0, 235.0, 247.0, 263.0, 252.0, 276.0, 254.0, 239.0, 240.0, 270.0, 277.0, 274.0, 281.0, 253.0, 264.0, 261.0, 260.0, 250.0, 246.0, 288.0, 250.0, 263.0, 280.0, 254.0, 282.0, 294.0, 271.0, 247.0, 281.0, 280.0, 291.0, 262.0, 266.0, 250.0, 284.0, 265.0, 263.0, 276.0, 242.0, 261.0, 272.0, 253.0, 281.0, 258.0, 243.0, 259.0, 296.0, 277.0, 274.0, 270.0, 255.0, 254.0, 279.0, 237.0, 309.0, 266.0, 282.0, 287.0, 280.0, 272.0, 277.0, 283.0, 253.0, 248.0, 233.0, 235.0, 252.0, 275.0, 263.0, 256.0, 273.0, 227.0, 270.0, 285.0, 293.0, 277.0, 291.0, 241.0, 300.0, 260.0, 226.0, 268.0, 324.0, 238.0, 241.0, 263.0, 269.0, 267.0, 257.0, 282.0, 260.0, 253.0, 245.0, 269.0, 289.0, 296.0, 277.0, 275.0, 304.0, 275.0, 274.0, 254.0, 296.0, 290.0, 266.0, 260.0, 259.0, 261.0, 269.0, 297.0, 270.0, 287.0, 261.0, 259.0, 285.0, 280.0, 273.0, 252.0, 240.0, 272.0, 292.0, 265.0, 253.0, 248.0, 256.0, 304.0, 264.0, 268.0, 261.0, 284.0, 259.0, 260.0, 298.0, 259.0, 276.0, 248.0, 279.0, 258.0, 257.0, 238.0, 242.0, 233.0, 269.0, 279.0, 281.0, 295.0, 272.0, 284.0, 255.0, 266.0, 235.0, 285.0, 268.0, 252.0, 279.0, 280.0, 268.0, 273.0, 249.0]
  out "Off-Line Smoothed":dbl[](array[numeric])=[37746.776569037655, 29454.479497907945, 47.42928870292886, 64.74518828451886, 126.95648535564857, 247.73682008368195, 450.3037656903766, 702.0548117154812, 929.1008368200837, 1151.820502092051, 1575.4753138075316, 2264.0861924686187, 3237.048535564853, 5451.531799163178, 10476.71380753138, 17234.289121338916, 23026.07154811716, 26134.548535564856, 27512.186610878656, 29537.99414225941, 33176.94184100417, 37749.17196652718, 40948.366527196646, 42027.971129707104, 40860.44602510459, 33468.356066945606, 20582.893723849378, 8585.125941422591, 1755.6845188284515, 68.99205020920499, 9.324686192468617, 3.182426778242678, 2.636401673640168, 0.598744769874478, -0.8887029288702915, -0.46192468619246724, -1.5560669456066938, -2.112552301255229, -1.3092050209205008, -1.1041841004184088, -1.2025104602510448, -0.6878661087866096, -0.3635983263598313, -0.10627615062761375, -1.7589958158995807, -2.941004184100417, -1.4075313807531367, -0.8405857740585763, -1.9682008368200832, -2.2715481171548113, -1.0456066945606681, -2.505857740585772, -4.631380753138073, -4.085355648535563, -3.3154811715481167, -2.874058577405857, -2.17949790794979, -2.0623430962343092, -2.6836820083682014, -1.1753138075313803, -0.7380753138075304, -2.6167364016736396, -3.0539748953974897, -3.3280334728033476, -2.371966527196652, -1.499581589958158, -2.7882845188284513, -3.3656903765690376, -1.790376569037656, -1.0728033472803333, -2.6167364016736396, -3.420083682008369, -2.959832635983264, -2.556066945606695, -2.6041841004184105, -2.888702928870293, -2.1062761506276146, -1.643933054393304, -2.1334728033472796, -2.5999999999999996, -2.6460251046025105, -1.3133891213389113, -0.9640167364016725, -2.8510460251046017, -3.1209205020920505, -3.1418410041841005, -2.2527196652719654, -1.4598326359832632, -3.687866108786611, -3.6857740585774064, -2.5728033472803356, -2.2882845188284517, -2.4744769874476984, -4.420083682008367, -4.401255230125522, -2.3175732217573217, -3.886610878661087, -4.748535564853556, -2.3866108786610876, -2.1209205020920496, -2.6146443514644355, -2.905439330543933, -2.1899581589958146, -1.3866108786610867, -1.7401673640167354, -1.7213389121338898, -1.8050209205020902, -2.014225941422593, -1.6313807531380746, -2.388702928870292, -2.539330543933054, -1.1481171548117144, -1.8656903765690374, -2.512133891213389, -1.309205020920501, -0.9933054393305427, -1.3991631799163167, -1.7527196652719652, -1.6502092050209192, -1.0184100418410027, -1.6941422594142255, -2.223430962343096, -1.1606694560669446, -1.6983263598326357, -3.127196652719665, -2.6041841004184088, -3.0769874476987438, -2.3343096234309617, 0.1364016736401687, 0.04853556485355792, -0.8154811715481157, -0.9347280334728016, -1.066527196652718, -0.2757322175732203, -0.08953974895397371, -1.5790794979079494, -0.6209205020920496, -0.024686192468617696, -1.1962343096234296, -1.0728033472803333, -1.947280334728033, -2.2820083682008363, -1.3824267782426767, -1.1690376569037646, -1.0811715481171533, -1.3615062761506258, -2.319665271966526, -2.3447698744769863, -1.8782426778242662, -1.392887029288702, -1.2882845188284506, -1.1376569037656892, -0.8928870292887015, -0.6648535564853543, -0.7882845188284505, -1.7589958158995807, -2.022594142259414, -1.677405857740585, -2.1209205020920496, -2.3677824267782417, -2.3635983263598317, -2.7736401673640168, -2.053974895397489, -0.7255230125522999, -2.1606694560669446, -2.3719665271966517, -0.46401673640167224, -1.1941422594142244, -1.8468619246861913, -1.6732217573221744, -1.522594142259413, -1.5602510460251038, -1.2841004184100409, -1.5058577405857734, -0.5016736401673632, 0.42928870292887167, -1.332217573221757, -1.3573221757322171, -0.8071129707112957, -0.5790794979079485, -0.15230125523012428, -0.9995815899581576, -0.46820083682008234, -0.2861924686192456, -1.3071129707112958, -1.3594142259414215, -1.451464435146442, -0.17112970711296926, 0.7723849372384951, -0.3092050209205008, -2.12928870292887, -2.152301255230125, 0.10083682008368328, 0.9794979079497921, 0.15732217573221885, -0.5100418410041827, -0.8677824267782412, -0.4075313807531368, 0.05899581589958289, 0.6301255230125538, 0.2933054393305454, -0.4493723849372371, 0.5234309623430977, -1.0539748953974886, -2.7046025104602505, -1.1836820083681998, -0.20460251046024977, 0.27029288702929, 1.161506276150629, 0.09456066945606834, -1.3615062761506262, -1.7715481171548104, -1.9953974895397475, -1.116736401673639, -0.05606694560669328, 0.06527196652719794, -0.12092050209204892, 0.10502092050209341, 0.9000000000000014, -0.07489539748953855, -0.9682008368200825, 0.6426778242677837, 0.6970711297071143, -0.6397489539748942, -0.9744769874476975, -1.7443514644351468, -1.4158995815899582, -0.36778242677824136, -0.7694560669456056, -1.4284518828451866, -0.9891213389121322, -0.018410041841002894, -0.6062761506276139, -1.4012552301255217, -0.2694560669456053, -0.11255230125522875, -2.1899581589958155, -1.8447698744769871, -0.1669456066945594, 0.15941422594142388, -0.4200836820083671, -1.3677824267782417, -2.1585774058577396, -0.8008368200836811, 0.26192468619246995, -0.03514644351464313, 0.876987447698746, -0.3573221757322167, -0.9138075313807522, 0.3079497907949804, 0.4523012552301268, -0.03514644351464308, -1.4619246861924675, -2.2066945606694546, 0.38953974895397625, 1.000418410041842, -0.28828451882845046, -0.2736401673640153, 0.16987447698744923, 0.008786610878662615, 0.4836820083682023, 1.3246861924686206, 0.6238493723849385, 0.0861924686192482, -1.2087866108786598, -0.6146443514644341, 0.029707112970712435, -0.6753138075313795, -0.846861924686191, -0.0037656903765675986, 0.22845188284518958, 0.2514644351464448, 0.667782426778244, 0.32677824267782557, 0.21380753138075442, -0.10418410041840882, -0.40543933054393183]
  out "On-Line  Smoothed":dbl[](array[numeric])=[37703.43472803346, 29509.706694560657, 43.83012552301257, 53.66694560669459, 97.91589958159001, 184.22133891213386, 325.5686192468618, 489.87615062761483, 625.6251046025103, 741.9577405857742, 975.6941422594149, 1371.685774058578, 1916.7527196652723, 3129.231799163179, 6118.123012552298, 10431.04979079498, 14121.120920502097, 15844.980753138081, 16271.277824267789, 17183.702510460265, 19109.478661087887, 21459.468200836833, 22928.926359832643, 23092.443096234318, 21578.650209205036, 16563.65020920503, 9431.40753138075, 3587.0205020920484, 631.4807531380759, 20.579079497907937, 3.0142259414225934, 0.49121338912133766, -0.5485355648535578, -0.6949790794979093, 0.10627615062761378, 0.9807531380753125, -0.21171548117154937, -2.278661087866111, -1.891631799163182, -0.8414225941422606, -1.0924686192468633, -2.3079497907949817, -2.9146443514644376, -2.086192468619248, -2.24100418410042, -2.9836820083682025, -2.931380753138077, -2.6384937238493746, -2.0129707112970725, -1.7347280334728046, -2.7849372384937245, -2.8602510460251054, -2.7012552301255246, -2.966945606694562, -1.2974895397489552, -1.4209205020920523, -2.473221757322178, -2.5841004184100433, -2.9899581589958175, -1.9167364016736415, -0.2953974895397502, -0.7786610878661099, -1.1238493723849383, -1.3309623430962358, -1.6887029288702942, -1.2430962343096246, -0.8184100418410054, -1.634309623430964, -2.8100418410041863, -3.1196652719665283, -2.6719665271966533, -1.5297071129707125, -3.1029288702928874, -3.2577405857740587, -1.492050209205022, -2.201255230125524, -1.9543933054393317, -1.7326359832636005, -1.6259414225941442, -1.584100418410043, -1.6364016736401685, -2.2953974895397504, -2.8351464435146454, -1.8623430962343108, -1.8205020920502104, -2.0757322175732216, -1.406276150627615, -2.406276150627616, -2.939748953974896, -1.7933054393305452, -2.0297071129707125, -1.8372384937238508, -1.2535564853556498, -0.5401673640167377, -1.20334728033473, -1.722175732217575, -1.8644351464435163, -2.8121338912133913, -2.510878661087868, -2.040167364016737, -0.9627615062761514, -0.36652719665272093, -1.0338912133891225, -2.28702928870293, -3.1468619246861937, -3.3602510460251063, -2.1615062761506287, -1.678242677824269, -2.2556485355648546, -1.6552301255230137, -1.6175732217573235, -1.7807531380753152, -1.9543933054393319, -1.7577405857740598, -1.073640167364018, -2.180334728033474, -2.5631799163179925, -1.628033472803348, -2.052719665271969, -1.5527196652719688, -1.485774058577407, -1.772384937238495, -1.7974895397489559, -1.7138075313807548, -1.1510460251046037, -0.7284518828451896, -1.0966527196652733, -1.983682008368202, -1.4732217573221769, -1.1845188284518842, -2.031799163179917, -2.117573221757323, -1.8456066945606708, -2.314225941422596, -1.2033472803347296, -1.1426778242677833, -1.9230125523012562, 0.34267782426778093, 0.09372384937238365, -1.469037656903767, -1.567364016736403, -1.9836820083682025, -1.3142259414225959, -1.9523012552301269, -2.345606694560671, -2.211715481171549, -2.7410041841004196, -2.6615062761506287, -1.6154811715481183, -1.0799163179916325, -2.1761506276150637, -2.4878661087866125, 0.1711297071129696, 2.1648535564853546, 0.11255230125522886, -0.5297071129707126, -1.533891213389123, -1.8811715481171565, -1.2117154811715491, -1.7305439330543946, -1.2179916317991646, -0.8518828451882858, -0.962761506276152, -1.1050209205020933, -1.1133891213389133, -1.1866108786610892, -1.2619246861924702, -1.552719665271968, -0.8665271966527209, -1.7765690376569054, -2.1949790794979096, -0.4167364016736415, -0.4690376569037671, -2.002510460251047, -2.4460251046025117, -1.169874476987449, -0.1322175732217586, 0.7464435146443502, -0.5799163179916333, -1.1824267782426794, -0.6824267782426792, -1.3184100418410054, -1.4543933054393317, -1.764016736401675, -1.8225941422594156, -2.0213389121338934, -2.2326359832636005, -1.5338912133891225, -0.9523012552301269, -1.9104602510460271, -1.807949790794981, -0.6175732217573234, -2.058995815899584, -2.623849372384939, -1.167782426778244, -0.06527196652719791, -0.02552301255230255, 0.18995815899581464, -0.7786610878661104, -1.6782426778242694, -1.1907949790794992, -2.079916317991633, -1.190794979079499, -0.9753138075313821, -1.6468619246861937, -1.1405857740585787, -1.5025104602510468, -0.6803347280334736, 0.08326359832635857, -0.2556485355648548, -0.7326359832635996, -0.5589958158995829, 0.003765690376567682, -0.849790794979081, -2.3225941422594154, -1.8163179916318002, -1.529707112970713, -1.3832635983263617, -0.15313807531380882, 0.022594142259412933, 0.1690376569037644, -0.4418410041841017, 0.007949790794977818, 0.7673640167364004, 0.9535564853556472, 0.36778242677824136, -0.5359832635983276, 1.2359832635983246, -0.0673640167364038, -1.7535564853556502, -0.5422594142259427, -0.13430962343096356, -0.02761506276150763, -0.5945606694560683, -1.0464435146443527, -1.6175732217573233, -1.4125523012552315, -0.1510460251046039, -0.169874476987449, -0.7472803347280348, -1.8728033472803358, -1.7368200836820096, 0.32175732217573083, -0.16987447698744895, -1.3456066945606708, -0.5945606694560682, -0.019246861924687414, -1.048535564853558, -0.29958158995816053, 0.9723849372384924, 0.6753138075313795, 0.49330543933054266, -0.0317991631799176, -0.06736401673640295, -0.9941422594142273, -2.038075313807533, -1.2765690376569052, -0.9209205020920516, -0.14686192468619375, 0.05397489539748829, 0.2841004184100406, 1.1041841004184088, -0.061087866108787914, -0.5778242677824281, -0.7263598326359846, -1.3874476987447704, -0.3623430962343102, 0.5330543933054381, -0.3184100418410054, 0.3615062761506263, 1.7297071129707107, 0.24016736401673577, -1.2828451882845195, 1.1502092050209194, 1.5853556485355633, 0.09163179916317865, -0.19497907949790916]
  out "On-Line Bin Readings":dbl[](array[numeric])=[16808.0, 59286.0, 293.0, 344.0, 381.0, 425.0, 541.0, 665.0, 829.0, 937.0, 897.0, 835.0, 838.0, 1573.0, 10396.0, 27362.0, 34889.0, 35728.0, 32533.0, 27558.0, 24714.0, 19555.0, 12779.0, 9363.0, 6887.0, 6779.0, 9610.0, 7139.0, 915.0, 279.0, 254.0, 293.0, 252.0, 243.0, 240.0, 273.0, 282.0, 259.0, 253.0, 265.0, 265.0, 289.0, 263.0, 260.0, 262.0, 245.0, 287.0, 272.0, 263.0, 259.0, 263.0, 287.0, 249.0, 245.0, 258.0, 282.0, 250.0, 255.0, 279.0, 269.0, 257.0, 267.0, 266.0, 247.0, 290.0, 270.0, 259.0, 276.0, 301.0, 283.0, 268.0, 272.0, 292.0, 279.0, 272.0, 257.0, 290.0, 253.0, 247.0, 287.0, 261.0, 254.0, 254.0, 267.0, 267.0, 278.0, 258.0, 298.0, 278.0, 246.0, 299.0, 280.0, 307.0, 278.0, 249.0, 286.0, 289.0, 271.0, 245.0, 258.0, 252.0, 265.0, 232.0, 275.0, 263.0, 268.0, 284.0, 263.0, 278.0, 277.0, 243.0, 251.0, 295.0, 267.0, 275.0, 286.0, 273.0, 277.0, 249.0, 255.0, 236.0, 263.0, 261.0, 263.0, 257.0, 273.0, 280.0, 246.0, 250.0, 271.0, 273.0, 269.0, 246.0, 239.0, 275.0, 279.0, 279.0, 265.0, 262.0, 257.0, 248.0, 251.0, 265.0, 274.0, 260.0, 266.0, 258.0, 260.0, 275.0, 263.0, 293.0, 255.0, 268.0, 236.0, 273.0, 272.0, 268.0, 247.0, 277.0, 264.0, 265.0, 255.0, 263.0, 270.0, 269.0, 279.0, 258.0, 259.0, 267.0, 284.0, 277.0, 266.0, 269.0, 261.0, 252.0, 258.0, 277.0, 268.0, 284.0, 302.0, 265.0, 254.0, 263.0, 269.0, 318.0, 268.0, 273.0, 274.0, 258.0, 263.0, 305.0, 256.0, 288.0, 260.0, 244.0, 296.0, 248.0, 246.0, 246.0, 230.0, 239.0, 280.0, 250.0, 292.0, 260.0, 306.0, 283.0, 260.0, 260.0, 287.0, 241.0, 267.0, 274.0, 254.0, 270.0, 233.0, 259.0, 260.0, 271.0, 263.0, 262.0, 291.0, 298.0, 279.0, 262.0, 220.0, 241.0, 314.0, 280.0, 274.0, 250.0, 275.0, 272.0, 278.0, 269.0, 240.0, 262.0, 273.0, 252.0, 264.0, 294.0, 255.0, 277.0, 261.0, 262.0, 280.0, 255.0, 279.0, 265.0, 293.0, 258.0, 239.0, 254.0, 268.0, 279.0, 276.0, 288.0, 293.0, 250.0, 297.0, 267.0, 298.0, 305.0, 268.0, 267.0, 259.0, 252.0, 271.0, 289.0, 244.0, 275.0, 257.0, 268.0, 250.0, 283.0, 271.0, 250.0, 251.0, 275.0]
  out "Range Corrected Altitude Array":dbl[](array[numeric])=[5625.0, 22500.0, 50625.0, 90000.0, 140625.0, 202500.0, 275625.0, 360000.0, 455625.0, 562500.0, 680625.0, 810000.0, 950625.0, 1102500.0, 1265625.0, 1440000.0, 1625625.0, 1822500.0, 2030625.0, 2250000.0, 2480625.0, 2722500.0, 2975625.0, 3240000.0, 3515625.0, 3802500.0, 4100625.0, 4410000.0, 4730625.0, 5062500.0, 5405625.0, 5760000.0, 6125625.0, 6502500.0, 6890625.0, 7290000.0, 7700625.0, 8122500.0, 8555625.0, 9000000.0, 9455625.0, 9922500.0, 10400625.0, 10890000.0, 11390625.0, 11902500.0, 12425625.0, 12960000.0, 13505625.0, 14062500.0, 14630625.0, 15210000.0, 15800625.0, 16402500.0, 17015625.0, 17640000.0, 18275625.0, 18922500.0, 19580625.0, 20250000.0, 20930625.0, 21622500.0, 22325625.0, 23040000.0, 23765625.0, 24502500.0, 25250625.0, 26010000.0, 26780625.0, 27562500.0, 28355625.0, 29160000.0, 29975625.0, 30802500.0, 31640625.0, 32490000.0, 33350625.0, 34222500.0, 35105625.0, 36000000.0, 36905625.0, 37822500.0, 38750625.0, 39690000.0, 40640625.0, 41602500.0, 42575625.0, 43560000.0, 44555625.0, 45562500.0, 46580625.0, 47610000.0, 48650625.0, 49702500.0, 50765625.0, 51840000.0, 52925625.0, 54022500.0, 55130625.0, 56250000.0, 57380625.0, 58522500.0, 59675625.0, 60840000.0, 62015625.0, 63202500.0, 64400625.0, 65610000.0, 66830625.0, 68062500.0, 69305625.0, 70560000.0, 71825625.0, 73102500.0, 74390625.0, 75690000.0, 77000625.0, 78322500.0, 79655625.0, 81000000.0, 82355625.0, 83722500.0, 85100625.0, 86490000.0, 87890625.0, 89302500.0, 90725625.0, 92160000.0, 93605625.0, 95062500.0, 96530625.0, 98010000.0, 99500625.0, 101002500.0, 102515625.0, 104040000.0, 105575625.0, 107122500.0, 108680625.0, 110250000.0, 111830625.0, 113422500.0, 115025625.0, 116640000.0, 118265625.0, 119902500.0, 121550625.0, 123210000.0, 124880625.0, 126562500.0, 128255625.0, 129960000.0, 131675625.0, 133402500.0, 135140625.0, 136890000.0, 138650625.0, 140422500.0, 142205625.0, 144000000.0, 145805625.0, 147622500.0, 149450625.0, 151290000.0, 153140625.0, 155002500.0, 156875625.0, 158760000.0, 160655625.0, 162562500.0, 164480625.0, 166410000.0, 168350625.0, 170302500.0, 172265625.0, 174240000.0, 176225625.0, 178222500.0, 180230625.0, 182250000.0, 184280625.0, 186322500.0, 188375625.0, 190440000.0, 192515625.0, 194602500.0, 196700625.0, 198810000.0, 200930625.0, 203062500.0, 205205625.0, 207360000.0, 209525625.0, 211702500.0, 213890625.0, 216090000.0, 218300625.0, 220522500.0, 222755625.0, 225000000.0, 227255625.0, 229522500.0, 231800625.0, 234090000.0, 236390625.0, 238702500.0, 241025625.0, 243360000.0, 245705625.0, 248062500.0, 250430625.0, 252810000.0, 255200625.0, 257602500.0, 260015625.0, 262440000.0, 264875625.0, 267322500.0, 269780625.0, 272250000.0, 274730625.0, 277222500.0, 279725625.0, 282240000.0, 284765625.0, 287302500.0, 289850625.0, 292410000.0, 294980625.0, 297562500.0, 300155625.0, 302760000.0, 305375625.0, 308002500.0, 310640625.0, 313290000.0, 315950625.0, 318622500.0, 321305625.0, 324000000.0, 326705625.0, 329422500.0, 332150625.0, 334890000.0, 337640625.0, 340402500.0, 343175625.0, 345960000.0, 348755625.0, 351562500.0, 354380625.0, 357210000.0, 360050625.0, 362902500.0, 365765625.0, 368640000.0, 371525625.0, 374422500.0, 377330625.0, 380250000.0, 383180625.0, 386122500.0, 389075625.0, 392040000.0, 395015625.0, 398002500.0, 401000625.0, 404010000.0, 407030625.0, 410062500.0, 413105625.0, 416160000.0, 419225625.0, 422302500.0, 425390625.0, 428490000.0, 431600625.0, 434722500.0, 437855625.0, 441000000.0]
  out "Altitude Array (km)":dbl[](array[numeric])=[0.075, 0.15, 0.22499999999999998, 0.3, 0.375, 0.45, 0.5249999999999999, 0.6, 0.6749999999999999, 0.7499999999999999, 0.825, 0.8999999999999999, 0.9749999999999999, 1.05, 1.125, 1.2, 1.275, 1.3499999999999999, 1.4249999999999998, 1.5, 1.575, 1.65, 1.7249999999999999, 1.7999999999999998, 1.8749999999999998, 1.95, 2.025, 2.1, 2.1750000000000003, 2.25, 2.325, 2.4, 2.475, 2.5500000000000003, 2.625, 2.7, 2.775, 2.85, 2.9250000000000003, 3.0, 3.075, 3.15, 3.225, 3.3000000000000003, 3.375, 3.45, 3.525, 3.6, 3.675, 3.75, 3.825, 3.9, 3.975, 4.05, 4.125, 4.2, 4.275, 4.35, 4.425, 4.5, 4.575, 4.65, 4.725, 4.8, 4.875, 4.95, 5.025, 5.1, 5.175, 5.25, 5.325, 5.4, 5.475, 5.55, 5.625, 5.7, 5.775, 5.85, 5.925, 6.0, 6.075, 6.15, 6.225, 6.3, 6.375, 6.45, 6.525, 6.6, 6.675, 6.75, 6.825, 6.9, 6.975, 7.05, 7.125, 7.2, 7.2749999999999995, 7.35, 7.425, 7.5, 7.575, 7.6499999999999995, 7.725, 7.8, 7.875, 7.95, 8.024999999999999, 8.1, 8.174999999999999, 8.249999999999998, 8.325, 8.399999999999999, 8.475, 8.549999999999999, 8.624999999999998, 8.7, 8.774999999999999, 8.85, 8.924999999999999, 8.999999999999998, 9.075, 9.149999999999999, 9.225, 9.299999999999999, 9.374999999999998, 9.45, 9.524999999999999, 9.6, 9.674999999999999, 9.749999999999998, 9.825, 9.899999999999999, 9.975, 10.049999999999999, 10.124999999999998, 10.2, 10.274999999999999, 10.35, 10.424999999999999, 10.499999999999998, 10.575, 10.649999999999999, 10.725, 10.799999999999999, 10.874999999999998, 10.95, 11.024999999999999, 11.1, 11.174999999999999, 11.249999999999998, 11.325, 11.399999999999999, 11.475, 11.549999999999999, 11.624999999999998, 11.7, 11.774999999999999, 11.85, 11.924999999999999, 11.999999999999998, 12.075, 12.149999999999999, 12.225, 12.299999999999999, 12.374999999999998, 12.45, 12.524999999999999, 12.6, 12.674999999999999, 12.749999999999998, 12.825, 12.899999999999999, 12.975, 13.049999999999999, 13.124999999999998, 13.2, 13.274999999999999, 13.35, 13.424999999999999, 13.499999999999998, 13.575, 13.649999999999999, 13.725, 13.799999999999999, 13.874999999999998, 13.95, 14.024999999999999, 14.1, 14.174999999999999, 14.249999999999998, 14.325, 14.399999999999999, 14.474999999999998, 14.549999999999999, 14.624999999999998, 14.7, 14.774999999999999, 14.849999999999998, 14.924999999999999, 14.999999999999998, 15.075, 15.149999999999999, 15.224999999999998, 15.299999999999999, 15.374999999999998, 15.45, 15.524999999999999, 15.599999999999998, 15.674999999999999, 15.749999999999998, 15.825, 15.899999999999999, 15.974999999999998, 16.05, 16.125, 16.2, 16.275, 16.349999999999998, 16.424999999999997, 16.5, 16.575, 16.65, 16.724999999999998, 16.799999999999997, 16.875, 16.95, 17.025, 17.099999999999998, 17.174999999999997, 17.25, 17.325, 17.4, 17.474999999999998, 17.549999999999997, 17.625, 17.7, 17.775, 17.849999999999998, 17.924999999999997, 18.0, 18.075, 18.15, 18.224999999999998, 18.299999999999997, 18.375, 18.45, 18.525, 18.599999999999998, 18.674999999999997, 18.75, 18.825, 18.9, 18.974999999999998, 19.049999999999997, 19.125, 19.2, 19.275, 19.349999999999998, 19.424999999999997, 19.5, 19.575, 19.65, 19.724999999999998, 19.799999999999997, 19.875, 19.95, 20.025, 20.099999999999998, 20.174999999999997, 20.25, 20.325, 20.4, 20.474999999999998, 20.549999999999997, 20.625, 20.7, 20.775, 20.849999999999998, 20.924999999999997, 21.0]
  out "Offline Pulse Energy":dbl
  out "Online Pulse Energy":dbl
  in  "Instrument Control":T5(tab)=enum."Wavemeter"
  out "Readings":T6={"OnLineTEC"=19.601099, "OnLineLD"=0.147824228, "OffLineTEC"=17.2473392, "OffLineLD"=0.153939456, "EtalonTEC"=25.8745461, "TSOA-TEC"=18.0106449, "Pro8000"=TRUE, "OnLine TEC"=TRUE, "OnLine LD"=TRUE, "OffLine TEC"=TRUE, "OffLine LD"=TRUE, "Etalon TEC"=TRUE, "TSOA TEC"=TRUE} {"OffLineLD" format="%.4g"; "OnLineLD" format="%.4g"; "TSOA-TEC" format="%.3g"; "EtalonTEC" format="%.3g"; "OffLineTEC" format="%.3g"; "OnLineTEC" format="%.3g"}
  in  "Settings":T7={"Module"=enum."On Line LD", "OnLineTEC"=19.62, "OnLineLD"=0.14766400000000265, "OffLineTEC"=17.36, "OffLineLD"=0.15419200000000619, "EtalonTEC"=26.6, "TSOA-TEC"=18.0} {"OffLineLD" min=0.0 max=0.175 step=0.001 format="%.3p"; "OnLineLD" min=0.0 max=0.175 step=0.001 format="%.3p"; "TSOA-TEC" format="%.2g"; "EtalonTEC" format="%.2g"; "OffLineTEC" min=0.0 max=30.0 step=0.1 format="%.2g"; "OnLineTEC" min=0.0 max=30.0 step=0.1 format="%.2g"}
  in  "Pulse B Polarity":enum32{"Low", "High"}(ring)=enum."High"
  in  "Pulse A Delay(ns)":u32=1040 min=80 max=327600
  in  "Pulse B Delay(ns)":u32=170000 min=80 max=327600 step=1
  in  "Accumulation Delay(ns)":u32=10 min=10 max=1270 step=1
  in  "Sync Pulse Polarity":enum32{"Low", "High"}(ring)=enum."High"
  in  "Pulse A Polarity":enum32{"Low", "High"}(ring)=enum."High"
  in  "Number of Bins":u32=280 min=2 max=4095 step=1
  in  "Number of Accumulates":u32=10000 min=1 max=32767 step=1
  in  "Time Resolution Per Bin(ns)":u32=500 min=5 max=1063 step=1
  in  "Cancel online":bool
  in  "Cancel Offline":bool
  in  "Lambda On Set (nm)":dbl=828.193 format="%.5f"
  out "Lambda On Read (nm)":dbl=828.1929788577258 format="%.5f"
  out "Lambda Off Read (nm)":dbl=828.292405520674 format="%.5f"
  in  "Lambda Off Set (nm)":dbl=828.29245 format="%#.5f"
  in  "Bristol In":i32=5
  out "Bristol Out":i32=1
  in  "AB_DIF":dbl=5e-05 format="%#_15g"
  in  "NONAB_DIF":dbl=5e-05 format="%#_15g"
  out "Wavelength Lock Online":bool=TRUE
  out "Wavelength Lock Offline":bool=TRUE
  out "WL Difference":dbl=-2.1142274135854677e-05 format="%_7g"
  out "WL Difference off":dbl=-4.4479325993052043e-05 format="%_7g"
  in  "calculate absorption cross sections":bool
  in  "Smoothing Range":dbl=150.0
  in  "Total DIAL Integration Time (Minutes)":i32=4
  in  "Data Reads (number of loops)":i32=1
  in  "Total Aerosol Integration Time (Minutes)":dbl=0.05
  in  "Scalar Wait Time":u32=1300
  out "Smoothed Bins":dbl=2.0
  in  "NewportIn":string
  in  "logging":bool
  out "Newport Device Key":string
  in  "SampleSize":i32=2
  out "NewportRef":refnum<k24>
  in  "Switch Comm Port":refnum<visa-resource-name>="COM3"
  out "FF_On_Ref":refnum<file>
  out "FF_On_Ptr":i64=1999712 format="%.2p"
  out "FF_Off_Ref":refnum<file>
  out "FF_Off_Ptr":i64=1999712 format="%.2p"
  out "NF_On_Ref":refnum<file>
  out "NF_On_Ptr":i64=1999712 format="%.2p"
  out "NF_Off_Ref":refnum<file>
  out "NF_Off_Ptr":i64=1999712 format="%.2p"
  out "DataOpen":bool=TRUE
  out "File Path_Far Field (out)":string="D:\\Micropulse_DIAL_data\\160307FF\\18"
  out "File Path_Near Field (out)":string="D:\\Micropulse_DIAL_data\\160307NF\\18"
  in  "Data File DIR (in)":string="D:\\Micropulse_DIAL_data\\"
  in  "bins":u32=280 min=2 max=4095 step=1
  out "y offset":u32=10
  in  "ns scale":u32=500
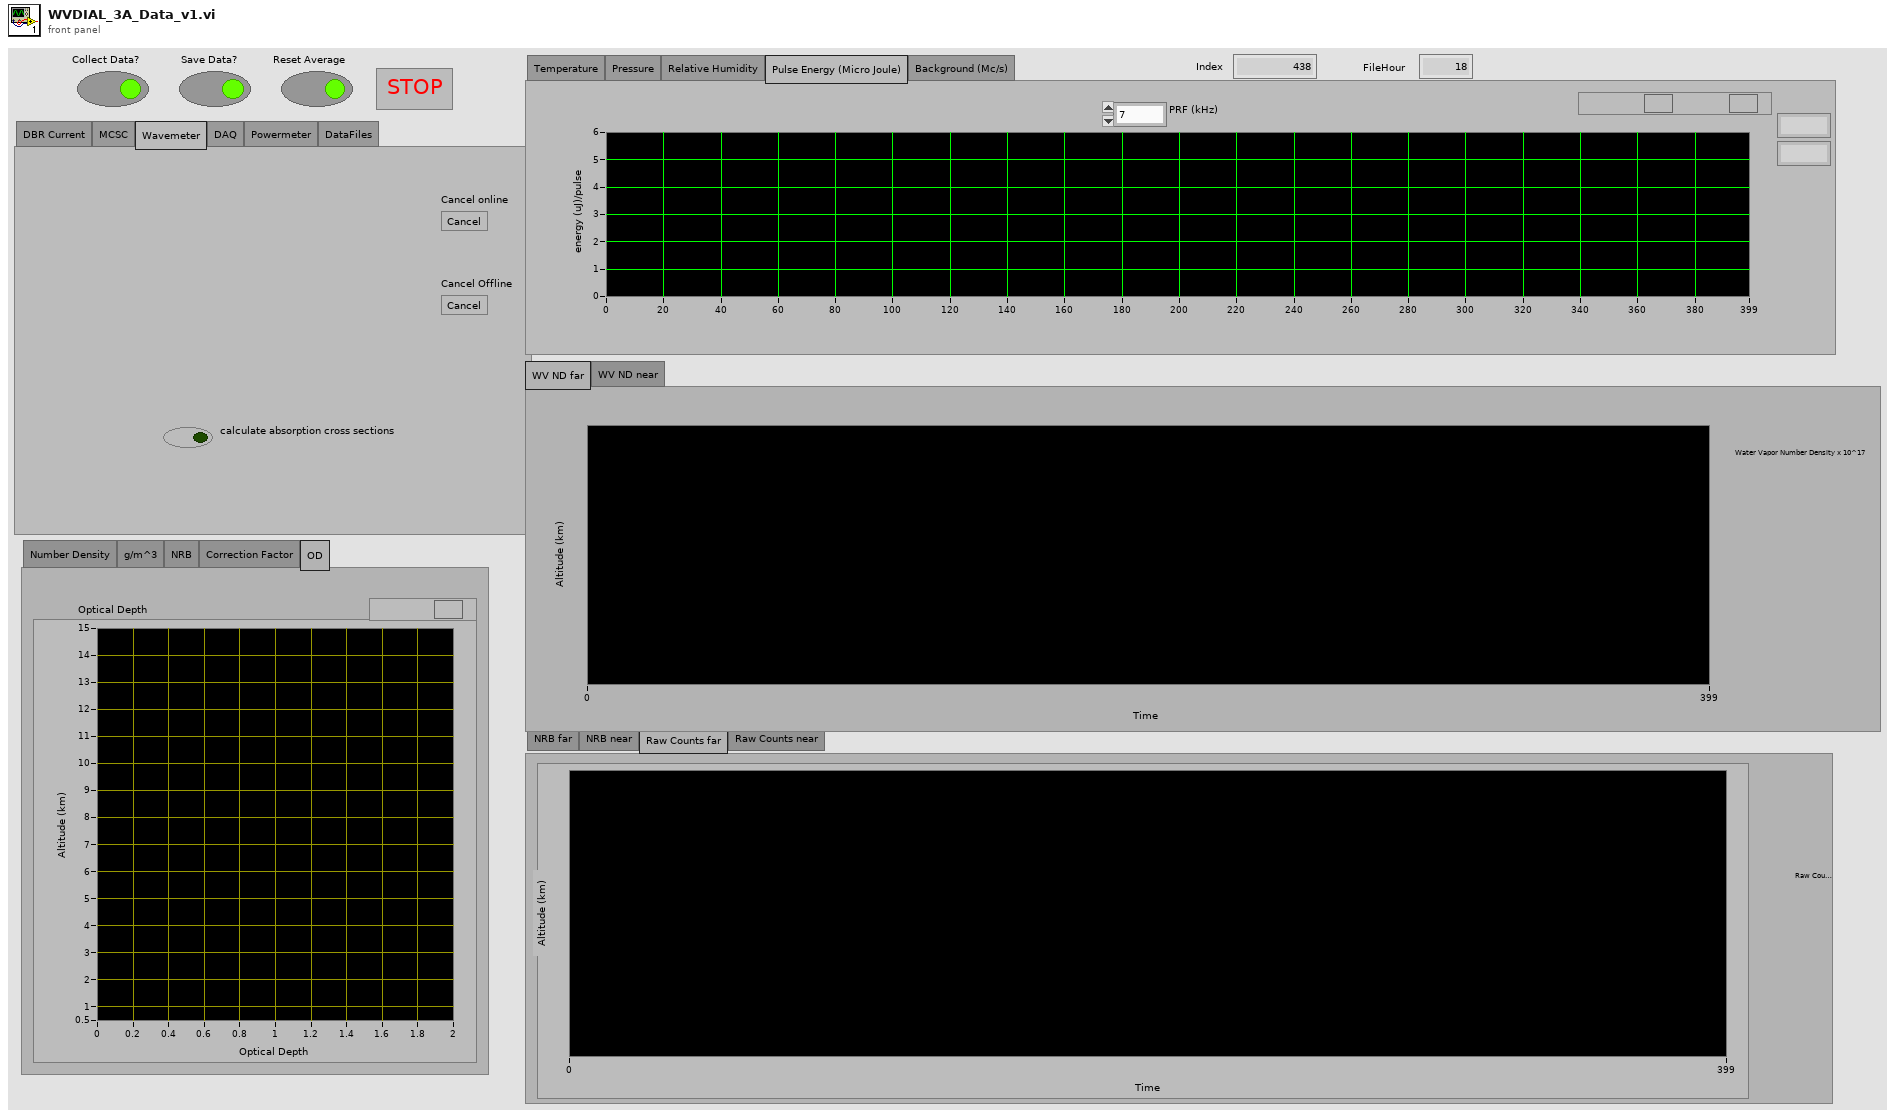
[diagram p1: front panel]
types:
  T1 = enum32{"NRB far", "NRB near", "Raw Counts far", "Raw Counts near"}
  T2 = enum32{"Number Density", "g/m^3", "NRB", "Correction Factor", "OD"}
  T3 = enum32{"Temperature", "Pressure", "Relative Humidity", "Pulse Energy (Micro Joule)", "Background (Mc/s)"}
  T4 = cluster{"Online Pulse Energy":dbl, "Pulse Energy Offline":dbl}
  T5 = enum32{"DBR Current", "MCSC", "Wavemeter", "DAQ", "Powermeter", "DataFiles"}
  T6 = cluster{"OnLineTEC":dbl, "OnLineLD":dbl, "OffLineTEC":dbl, "OffLineLD":dbl, "EtalonTEC":dbl, "TSOA-TEC":dbl, "Pro8000":bool, "OnLine TEC":bool, "OnLine LD":bool, "OffLine TEC":bool, "OffLine LD":bool, "Etalon TEC":bool, "TSOA TEC":bool}
  T7 = cluster{"Module":enum16{"On Line TEC", "On Line LD", "Off Line TEC", "Off Line LD", "Etalon TEC", "TSOA TEC"}, "OnLineTEC":dbl, "OnLineLD":dbl, "OffLineTEC":dbl, "OffLineLD":dbl, "EtalonTEC":dbl, "TSOA-TEC":dbl}
  T8 = enum16{"Open_TL", "Close_TL", "Verify_ID", "TEC_Sensor", "SET", "READ", "ON", "OFF", "Set_Limits", "Read_Limits", "Enable_Status", "Read_Status"}
  T9 = enum16{"Initialize ILX", "Set ON T", "Set Off T", "Set ON I", "Set Off I", "Set On Lim", "Set Off Lim", "Read ILX", "TEC ON/OFF", "LASER ON/OFF", "Status?", "ILX OFF"}
  T10 = enum16{"open", "replace", "create", "open or create", "replace or create", "replace or create with confirmation"}
  T11 = enum16{"On Line TEC", "On Line LD", "Off Line TEC", "Off Line LD", "Etalon TEC", "TSOA TEC"}
  T12 = typedef "LVDateTimeRec.ctl" = cluster{"fractional second":dbl, "second":i32, "minute":i32, "hour":i32, "day of month":i32, "month":i32, "year":i32, "day of week":i32, "day of year":i32, "DST":i32}
  T13 = cluster{"Online Pulse Energy":dbl, "Offline Pulse Energy":dbl}
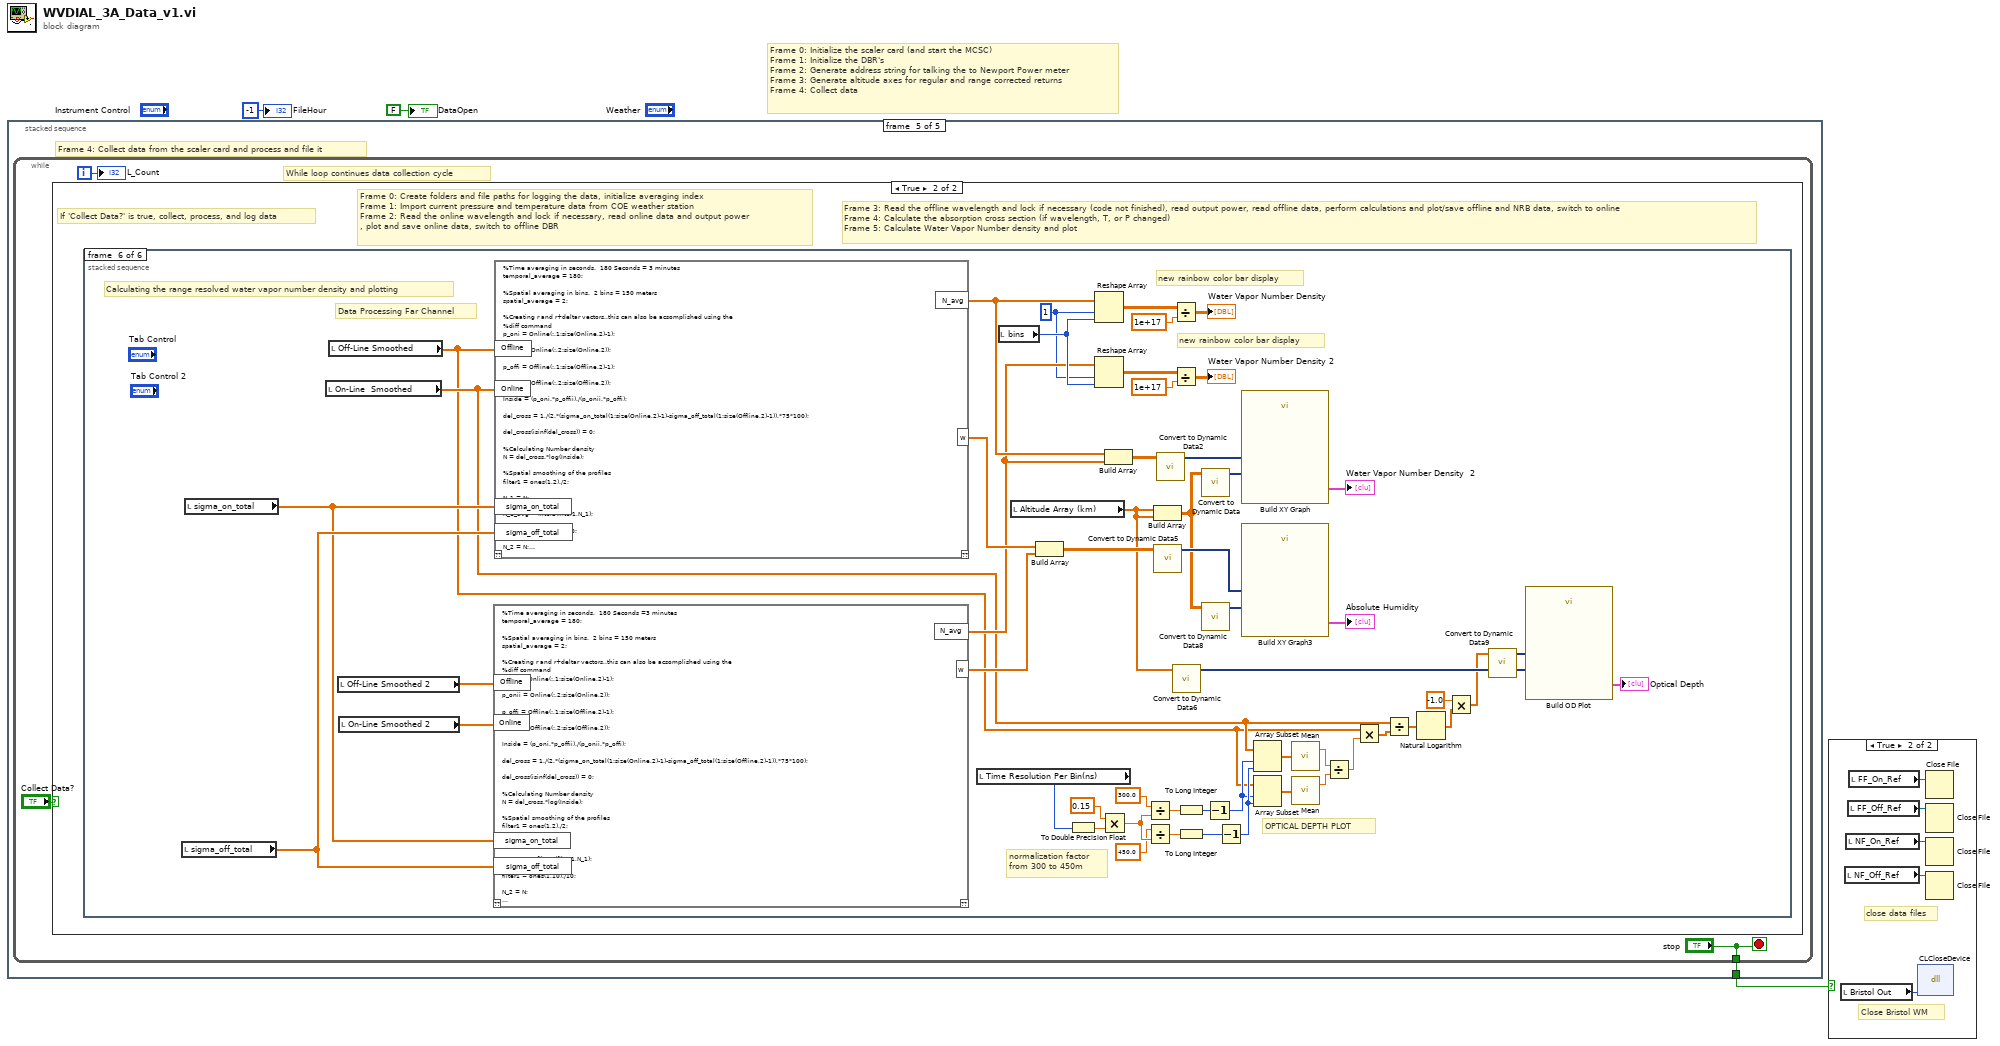
[diagram p0: block diagram]
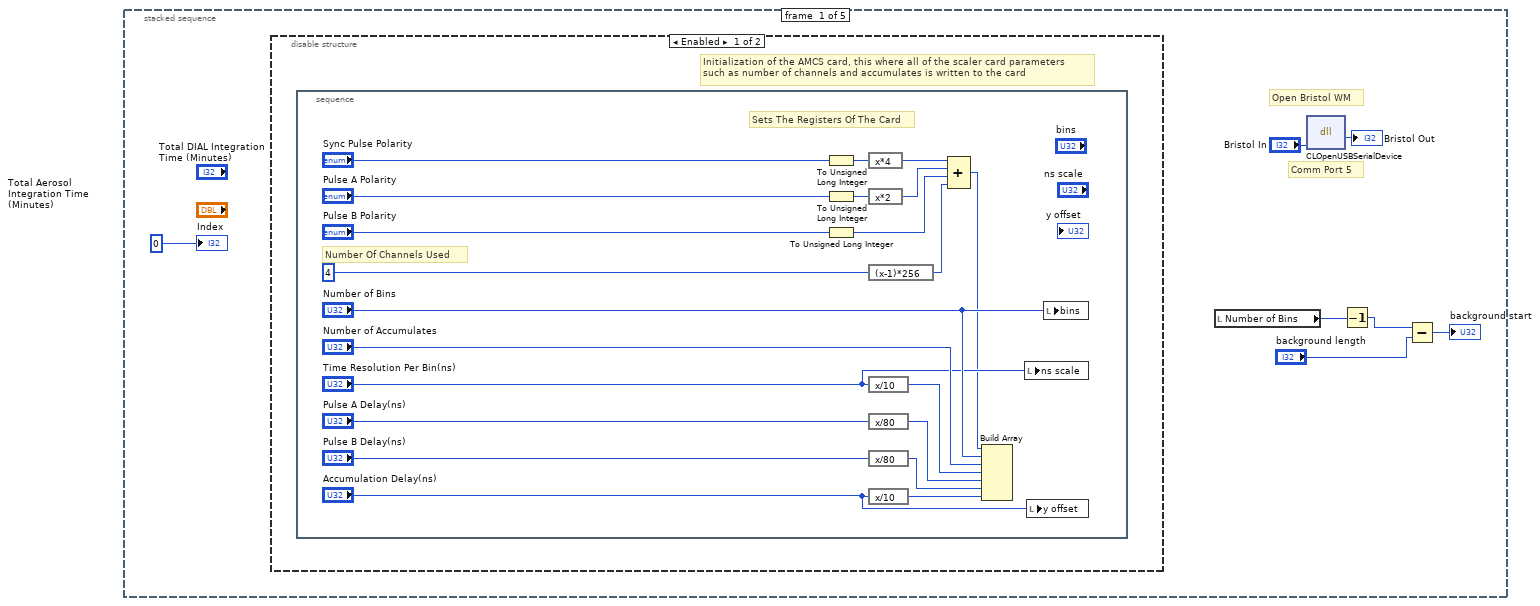
[diagram p3: hidden frame]
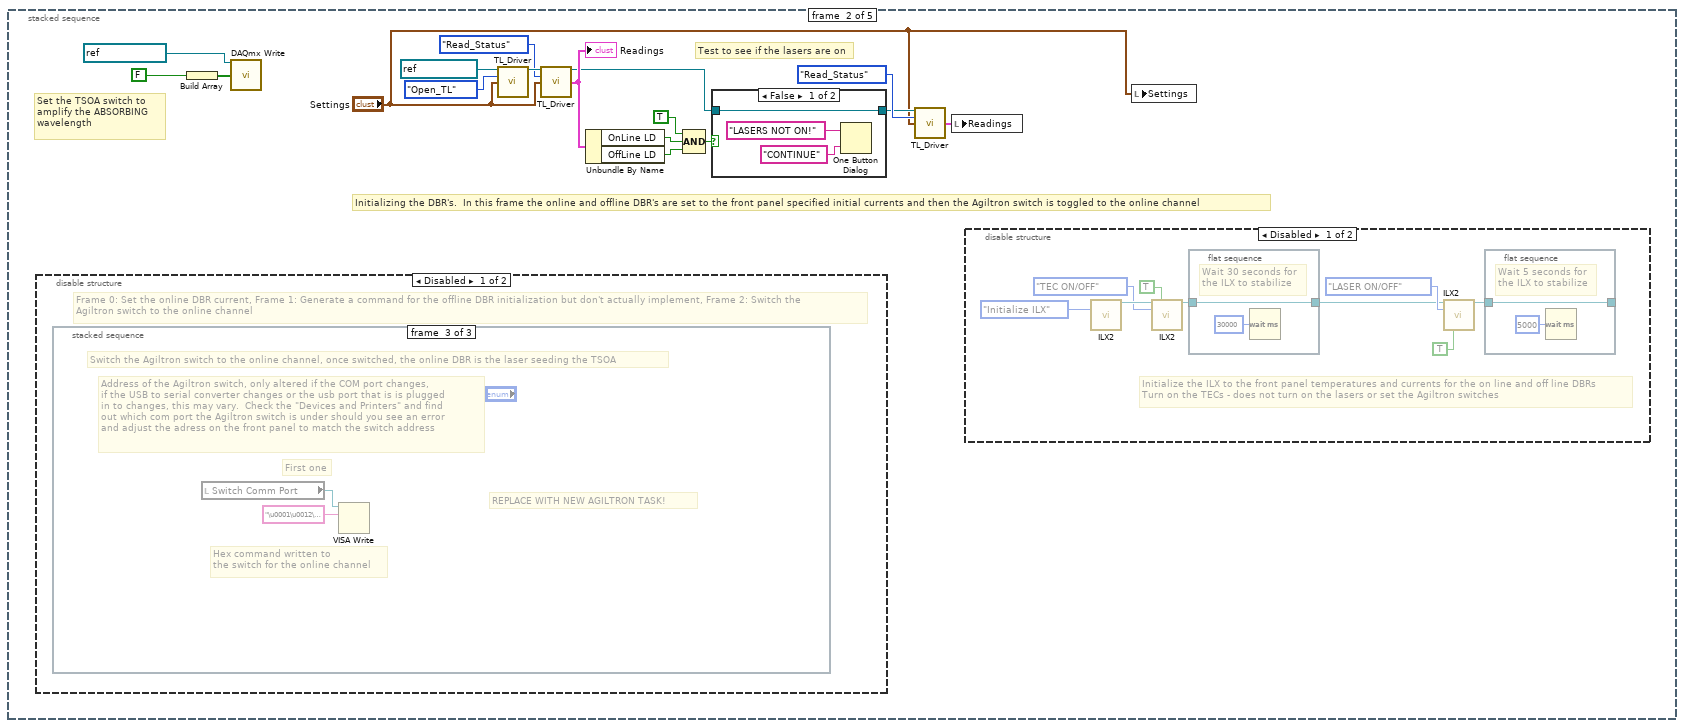
[diagram p5: hidden frame]
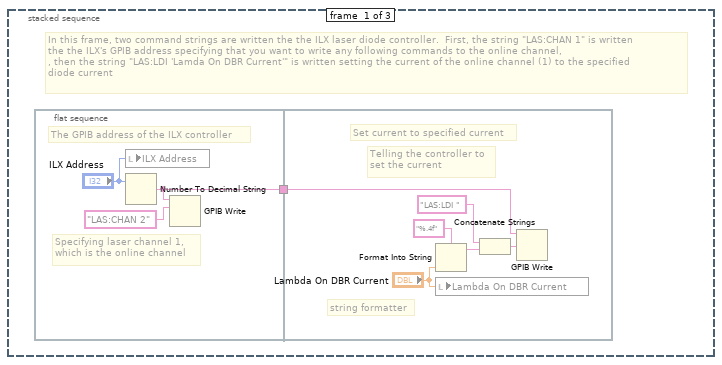
[diagram p8: hidden frame]
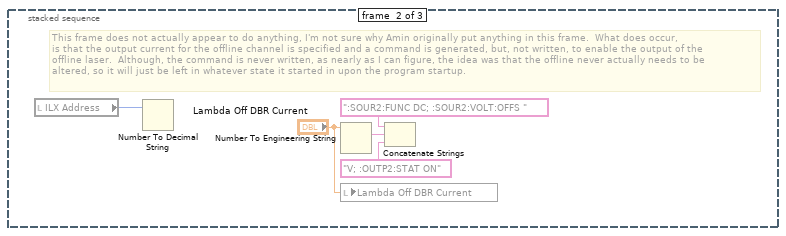
[diagram p9: hidden frame]
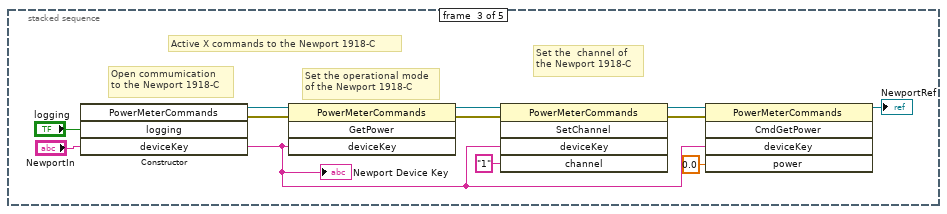
[diagram p11: hidden frame]
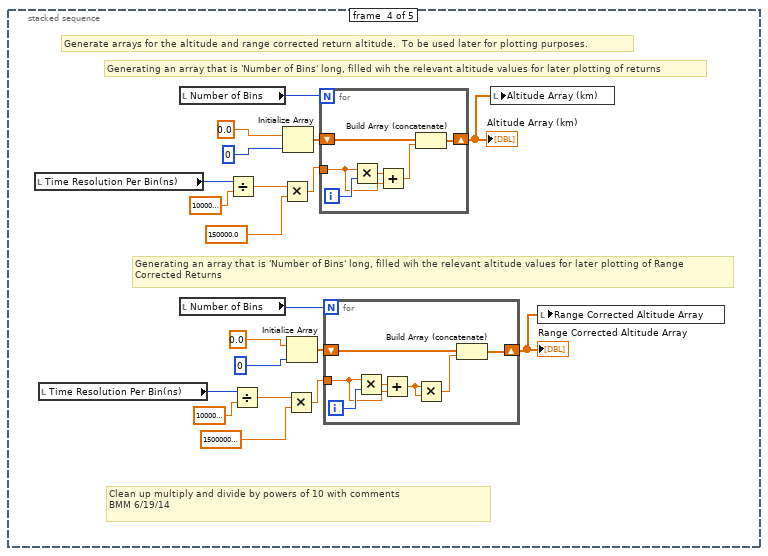
[diagram p12: hidden frame]
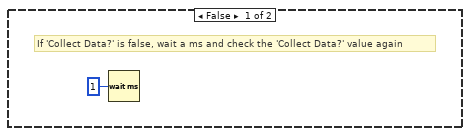
[diagram p13: hidden frame]
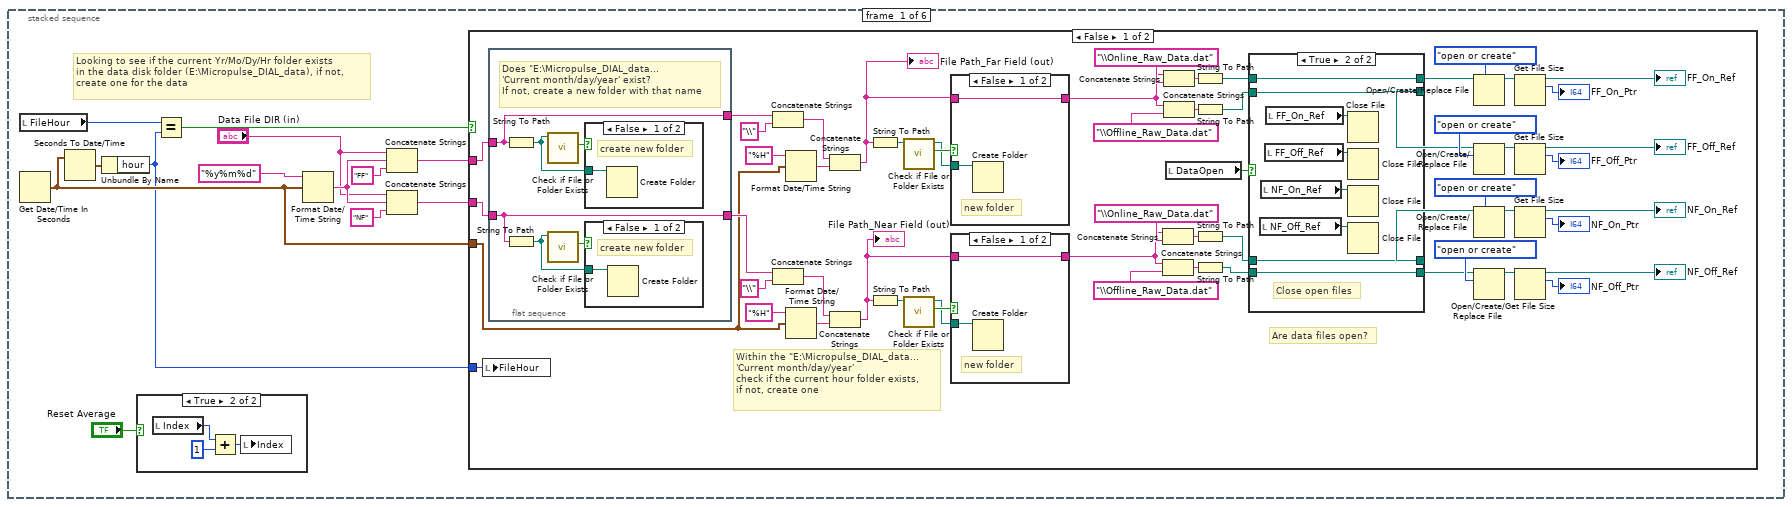
[diagram p14: hidden frame]
diagram:
  # "Frame 0: Initialize the scaler card (and start the MCSC)\nFrame 1: Initialize the DBR's\nFrame 2: Generate address string for talking the to Newport Power meter\nFrame 3: Generate altitude axes for regular and range corrected returns\nFrame 4: Collect data"
  n1 = stacked-sequence {
    tunnel: [_ _ _ _ w128] -> w3
    frame #0 {
      # "Comm Port 5"
      # "Open Bristol WM"
      n2 = disable-structure shown="Enabled" {
        frame Enabled {
          # "Initialization of the AMCS card, this where all of the scaler card parameters\nsuch as number of channels and accumulates is written to the card"
          n3 = stacked-sequence {
            frame #0 {
              # "Sets The Registers Of The Card"
              # "Number Of Channels Used"
              n4 = To Unsigned Long Integer(number="Sync Pulse Polarity") -> (unsigned 32bit integer=w11:u32)
              n5 = To Unsigned Long Integer(number="Pulse A Polarity") -> (unsigned 32bit integer=w15:u32)
              n6 = To Unsigned Long Integer(number="Pulse B Polarity") -> (unsigned 32bit integer=w13:u32)
              n7 = expression code="x*4"(w11) -> (w20:u32)
              n8 = expression code="x*2"(w15) -> (w19:u32)
              n9 = expression code="(x-1)*256"(u32 4 ("Number of Channels Used")) -> (w18:u32)
              n10 = expression code="x/10"("Time Resolution Per Bin(ns)") -> (w22:u32)
              n11 = expression code="x/80"("Pulse A Delay(ns)") -> (w29:u32)
              n12 = expression code="x/80"("Pulse B Delay(ns)") -> (w31:u32)
              n13 = expression code="x/10"("Accumulation Delay(ns)") -> (w30:u32)
              n14 = Compound Arithmetic op=ADD(w20, w19, w13, w18) -> (w17:u32)
              n15 = Build Array(w17, "Number of Bins", "Number of Accumulates", w22, w29, w31, w30) -> ()  [unwired: 1 out]
              n16 = local write "ns scale"("Time Resolution Per Bin(ns)") -> ()
              n17 = local write "y offset"("Accumulation Delay(ns)") -> ()
              n18 = local write "bins"("Number of Bins") -> ()
            }
          }
        }
        frame Disabled {
        }
      }
      n19 = local read "Number of Bins"() -> (w7:u32)
      n20 = dll-call lib="C:/H2O_DIAL/LabVIEW-2012/Bristol WM V2_31b/CLDevIface.dll" fn="CLOpenUSBSerialDevice"("commPort"="Bristol In") -> ("return type"=→"Bristol Out":i32)  [unwired: 4 in, 2 out]
      n21 = Decrement(x=w7) -> (x-1=w6:u32)
      n22 = Subtract(x=w6, y="background length") -> (x-y=→"background start":u32)
      "Index" <- 0 ("Index")
    }
    frame #1 {
      # "Test to see if the lasers are on"
      # "Set the TSOA switch to\namplify the ABSORBING\nwavelength"
      # "Initializing the DBR's.  In this frame the online and offline DBR's are set to the front panel specified initial currents and then the Agiltron switch is toggled to the online channel"
      n23 = disable-structure shown="Disabled" {
        frame Disabled {
          # "Frame 0: Set the online DBR current, Frame 1: Generate a command for the offline DBR initialization but don't actually implement, Frame 2: Switch the \nAgiltron switch to the online channel"
          n24 = stacked-sequence {
            frame #0 {
              # "In this frame, two command strings are written the the ILX laser diode controller.  First, the string \"LAS:CHAN 1\" is written\nthe the ILX's GPIB address specifying that you want to write any following commands to the online channel,\n, then the string \"LAS:LDI 'Lamda On DBR Current'\" is written setting the current of the online channel (1) to the specified \ndiode current"
              n25 = flat-sequence {
                tunnel: [w68] -> w66
                tunnel: w66 -> [w70]
                frame #0 {
                  # "The GPIB address of the ILX controller"
                  # "Specifying laser channel 1,\nwhich is the online channel"
                  n26 = local write "ILX Address"("ILX Address") -> ()
                  n27 = Number To Decimal String(number="ILX Address") -> (decimal integer string=w68:string)  [unwired: 1 in]
                  n28 = GPIB Write(0:w68, 1:"LAS:CHAN 2") -> ()  [unwired: 3 in, 2 out]
                }
                frame #1 {
                  # "Telling the controller to\nset the current"
                  # "string formatter"
                  # "Set current to specified current"
                  n29 = Format Into String(format string="%.4f" ("Format String"), "Lambda On DBR Current") -> (resulting string=w73:string)  [unwired: 2 in, 1 out]
                  n30 = local write "Lambda On DBR Current"("Lambda On DBR Current") -> ()
                  n31 = Concatenate Strings("LAS:LDI ", w73) -> (w74:string)
                  n32 = GPIB Write(0:w70, 1:w74) -> ()  [unwired: 3 in, 2 out]
                }
              }
            }
            frame #1 {
              # "This frame does not actually appear to do anything, I'm not sure why Amin originally put anything in this frame.  What does occur, \nis that the output current for the offline channel is specified and a command is generated, but, not written, to enable the output of the\noffline laser.  Although, the command is never written, as nearly as I can figure, the idea was that the offline never actually needs to be \naltered, so it will just be left in whatever state it started in upon the program startup."
              n33 = local read "ILX Address"() -> (w76:i32)
              n34 = Number To Decimal String(number=w76) -> ()  [unwired: 1 in, 1 out]
              n35 = Number To Engineering String(4:"Lambda Off DBR Current") -> (0:w80:string)  [unwired: 3 in]
              n36 = local write "Lambda Off DBR Current"("Lambda Off DBR Current") -> ()
              n37 = Concatenate Strings(":SOUR2:FUNC DC; :SOUR2:VOLT:OFFS ", w80, "V; :OUTP2:STAT ON") -> ()  [unwired: 1 out]
            }
            frame #2 {
              # "REPLACE WITH NEW AGILTRON TASK!"
              # "First one"
              # "Address of the Agiltron switch, only altered if the COM port changes,\nif the USB to serial converter changes or the usb port that is is plugged\nin to changes, this may vary.  Check the \"Devices and Printers\" and find \nout which com port the Agiltron switch is under should you see an error \nand adjust the adress on the front panel to match the switch address"
              # "Hex command written to \nthe switch for the online channel"
              # "Switch the Agiltron switch to the online channel, once switched, the online DBR is the laser seeding the TSOA"
              n38 = local read "Switch Comm Port"() -> (w81:refnum<visa-resource-name>)
              n39 = VISA Write(VISA resource name=w81, write buffer="\u0001\u0012\u0000\u0002") -> ()  [unwired: 1 in, 3 out]
            }
          }
        }
        frame Enabled {
        }
      }
      n40 = Build Array(FALSE ("Boolean")) -> (w33:bool[])
      n41 = call-poly <vilib>:"DAQmx Write.vi"("task/channels in"=refnum<k21> "BristolWM", "data"=w33) -> ()  [unwired: 11 in, 3 out]
      n42 = call "TL_Driver.vi"("Device In"=refnum<visa-resource-name> "ThorLabs", "Commands"=T8."Open_TL", "Settings"="Settings") -> ("Device Out"=w46:refnum<visa-resource-name>)  [unwired: 9 in, 3 out]
      n43 = call "TL_Driver.vi"("Device In"=w46, "Commands"=T8."Read_Status", "Settings"="Settings") -> ("Device Out"=w43:refnum<visa-resource-name>, "Readings"=w44:T6)  [unwired: 9 in, 2 out]
      "Readings" <- w44
      n44 = Unbundle By Name(w44) -> ("OnLine LD"=w38:bool, "OffLine LD"=w39:bool)
      n45 = Compound Arithmetic op=AND(TRUE, w38, w39) -> (w37:bool)
      n46 = case shown="False" w37 {
        tunnel: w43 -> [w49 w52]
        tunnel: [w49 w52] -> w41
        frame False {
          n47 = One Button Dialog(message="LASERS NOT ON!", button name ("OK")="CONTINUE") -> ()  [unwired: 1 out]
        }
        frame True {
        }
      }
      n48 = call "TL_Driver.vi"("Device In"=w41, "Commands"=T8."Read_Status", "Settings"="Settings") -> ("Readings"=w32:T6)  [unwired: 9 in, 3 out]
      n49 = local write "Readings"(w32) -> ()
      n50 = disable-structure shown="Disabled" {
        frame Disabled {
          # "Initialize the ILX to the front panel temperatures and currents for the on line and off line DBRs\nTurn on the TECs - does not turn on the lasers or set the Agiltron switches"
          n51 = call "ILX2.vi"("ILX Command"=T9."Initialize ILX") -> ("Device Out"=w60:refnum<visa-resource-name>)  [unwired: 10 in, 4 out]
          n52 = call "ILX2.vi"("Device In"=w60, "TEC Control"=TRUE, "ILX Command"=T9."TEC ON/OFF") -> ("Device Out"=w57:refnum<visa-resource-name>)  [unwired: 8 in, 4 out]
          n53 = flat-sequence {
            tunnel: w57 -> [w64]
            tunnel: [w64] -> w54
            frame #0 {
              # "Wait 30 seconds for\nthe ILX to stabilize"
              n54 = Wait (ms)(milliseconds to wait=u32 30000) -> ()  [unwired: 1 out]
            }
          }
          n55 = call "ILX2.vi"("Device In"=w54, "ILX Command"=T9."LASER ON/OFF", "Laser Control"=TRUE ("TEC Control")) -> ("Device Out"=w53:refnum<visa-resource-name>)  [unwired: 8 in, 4 out]
          n56 = flat-sequence {
            tunnel: w53 -> [w62]
            tunnel: [w62] -> _
            frame #0 {
              # "Wait 5 seconds for\nthe ILX to stabilize"
              n57 = Wait (ms)(milliseconds to wait=u32 5000) -> ()  [unwired: 1 out]
            }
          }
        }
        frame Enabled {
        }
      }
      n58 = local write "Settings"("Settings") -> ()
    }
    frame #2 {
      # "Active X commands to the Newport 1918-C"
      # "Set the  channel of\nthe Newport 1918-C"
      # "Set the operational mode\nof the Newport 1918-C"
      # "Open commumication\nto the Newport 1918-C"
      n59 = constructor class="PowerMeterCommands"("logging"="logging", "deviceKey"="NewportIn") -> (reference out=w94:refnum<k24>, error out=w91:errorcluster, "deviceKey"=w86:string)  [unwired: 3 in, 2 out]
      "Newport Device Key" <- w86
      n60 = invoke class="PowerMeterCommands" method="GetPower"(reference=w94, error in=w91, "deviceKey"=w86) -> (reference out=w93:refnum<k24>, error out=w90:errorcluster)  [unwired: 1 in, 2 out]
      n61 = invoke class="PowerMeterCommands" method="SetChannel"(reference=w93, error in=w90, "deviceKey"=w86, "channel"="1") -> (reference out=w87:refnum<k24>, error out=w89:errorcluster)  [unwired: 1 in, 3 out]
      n62 = invoke class="PowerMeterCommands" method="CmdGetPower"(reference=w87, error in=w89, "deviceKey"=w86, "power"=sgl 0.0) -> (reference out=→"NewportRef":refnum<k24>)  [unwired: 1 in, 4 out]
    }
    frame #3 {
      # "Clean up multiply and divide by powers of 10 with comments\nBMM 6/19/14"
      # "Generating an array that is 'Number of Bins' long, filled wih the relevant altitude values for later plotting of Range \nCorrected Returns"
      # "Generating an array that is 'Number of Bins' long, filled wih the relevant altitude values for later plotting of returns"
      # "Generate arrays for the altitude and range corrected return altitude.  To be used later for plotting purposes."
      n63 = local read "Time Resolution Per Bin(ns)"() -> (w107:u32)
      n64 = local read "Time Resolution Per Bin(ns)"() -> (w97:u32)
      n65 = local read "Number of Bins"() -> (w110:u32)
      n66 = local read "Number of Bins"() -> (w100:u32)
      n67 = Divide(x=w107, y=1000000000.0) -> (x/y=w105:dbl)
      n68 = Divide(x=w97, y=1000000000.0) -> (x/y=w95:dbl)
      n69 = Multiply(x=w105, y=150000.0) -> (x*y=w108:dbl)
      n70 = Initialize Array(0.0, 0) -> (w113:dbl[])
      n71 = Multiply(x=w95, y=150000000.0) -> (x*y=w98:dbl)
      n72 = Initialize Array(0.0, 0) -> (w103:dbl[])
      n73 = for {
        N: w110 -> [_]
        shift-right: [w126] -> w111
        shift-left: w113 -> [w127]
        tunnel: w108 -> [w123]
        i -> [w125]
        n74 = Multiply(x=w123, y=w125) -> (x*y=w124:dbl)
        n75 = Add(x=w124, y=w123) -> (x+y=w122:dbl)
        n76 = Build Array (concatenate)(w127, w122) -> (w126:dbl[])
      }
      "Altitude Array (km)" <- w111
      n77 = for {
        N: w100 -> [_]
        shift-right: [w120] -> w101
        shift-left: w103 -> [w121]
        tunnel: w98 -> [w116]
        i -> [w119]
        n78 = Multiply(x=w116, y=w119) -> (x*y=w117:dbl)
        n79 = Add(x=w117, y=w116) -> (x+y=w115:dbl)
        n80 = Multiply(x=w115, y=w115) -> (x*y=w118:dbl)
        n81 = Build Array (concatenate)(w121, w118) -> (w120:dbl[])
      }
      "Range Corrected Altitude Array" <- w101
      n82 = local write "Altitude Array (km)"(w111) -> ()
      n83 = local write "Range Corrected Altitude Array"(w101) -> ()
    }
    frame #4 {
      # "Frame 4: Collect data from the scaler card and process and file it"
      n84 = while {
        tunnel: ["stop"] -> w128
        i -> [w129]
        stop <- "stop" stop-if-true
        # "While loop continues data collection cycle"
        n85 = case shown="True" "Collect Data?" {
          frame False {
            # "If 'Collect Data?' is false, wait a ms and check the 'Collect Data?' value again"
            n86 = Wait (ms)(milliseconds to wait=u32 1) -> ()  [unwired: 1 out]
          }
          frame True {
            # "Frame 3: Read the offline wavelength and lock if necessary (code not finished), read output power, read offline data, perform calculations and plot/save offline and NRB data, switch to online\nFrame 4: Calculate the absorption cross section (if wavelength, T, or P changed)\nFrame 5: Calculate Water Vapor Number density and plot"
            # "Frame 0: Create folders and file paths for logging the data, initialize averaging index\nFrame 1: Import current pressure and temperature data from COE weather station\nFrame 2: Read the online wavelength and lock if necessary, read online data and output power\n, plot and save online data, switch to offline DBR"
            # "If 'Collect Data?' is true, collect, process, and log data"
            n87 = stacked-sequence {
              frame #0 {
                # "Looking to see if the current Yr/Mo/Dy/Hr folder exists\nin the data disk folder (E:\\Micropulse_DIAL_data), if not,\ncreate one for the data"
                n88 = local read "FileHour"() -> (w142:i32)
                n89 = Get Date/Time In Seconds() -> (seconds since 1Jan1904=w134:timestamp)
                n90 = Seconds To Date/Time(time stamp (now)=w134) -> (date time rec=w144:T12)  [unwired: 1 in]
                n91 = Unbundle By Name(w144) -> ("hour"=w133:i32)
                n92 = case shown="True" "Reset Average" {
                  frame False {
                    n93 = local write "Index"(0 ("Index")) -> ()
                  }
                  frame True {
                    n94 = local read "Index"() -> (w232:i32)
                    n95 = Add(x=w232, y=1) -> (x+y=w231:i32)
                    n96 = local write "Index"(w231) -> ()
                  }
                }
                n97 = Equal?(x=w142, y=w133) -> (x = y?=w143:bool)
                n98 = Format Date/Time String(time format string (%c)="%y%m%d", seconds (now)=w134) -> (date/time string=w138:string)  [unwired: 1 in]
                n99 = Concatenate Strings("Data File DIR (in)", w138, "FF" ("string")) -> (w140:string)
                n100 = Concatenate Strings("Data File DIR (in)", w138, "NF" ("string")) -> (w135:string)
                n101 = case shown="False" w143 {
                  tunnel: w140 -> [w202 _]
                  tunnel: w135 -> [w201 _]
                  tunnel: w134 -> [w188 _]
                  tunnel: w133 -> [w164 _]
                  frame False {
                    # "Are data files open?"
                    # "Within the \"E:\\Micropulse_DIAL_data...\n'Current month/day/year' \ncheck if the current hour folder exists,\nif not, create one"
                    n102 = local write "FileHour"(w164) -> ()
                    n103 = flat-sequence {
                      tunnel: [w222] -> w189
                      tunnel: w202 -> [w221]
                      tunnel: w201 -> [w222]
                      tunnel: [w221] -> w190
                      frame #0 {
                        # "Does \"E:\\Micropulse_DIAL_data...\n'Current month/day/year' exist?\nIf not, create a new folder with that name"
                        n104 = String To Path(string=w221) -> (path=w226:path)
                        n105 = String To Path(string=w222) -> (path=w224:path)
                        n106 = call <vilib>:"Check if File or Folder Exists.vi"("path"=w226) -> ("file or folder exists?"=w225:bool)  [unwired: 8 in, 2 out]
                        n107 = call <vilib>:"Check if File or Folder Exists.vi"("path"=w224) -> ("file or folder exists?"=w223:bool)  [unwired: 8 in, 2 out]
                        n108 = case shown="False" w225 {
                          tunnel: w226 -> [w228 _]
                          frame False {
                            # "create new folder"
                            n109 = Create Folder(path (use dialog)=w228) -> ()  [unwired: 2 in, 3 out]
                          }
                          frame True {
                            # "Folder exists\ndo nothing"
                          }
                        }
                        n110 = case shown="False" w223 {
                          tunnel: w224 -> [w227 _]
                          frame False {
                            # "create new folder"
                            n111 = Create Folder(path (use dialog)=w227) -> ()  [unwired: 2 in, 3 out]
                          }
                          frame True {
                            # "Folder exists\ndo nothing"
                          }
                        }
                      }
                    }
                    n112 = Concatenate Strings(w190, "\\" ("string")) -> (w197:string)
                    n113 = Concatenate Strings(w189, "\\" ("string")) -> (w192:string)
                    n114 = Format Date/Time String(time format string (%c)="%H", seconds (now)=w188) -> (date/time string=w200:string)  [unwired: 1 in]
                    n115 = Format Date/Time String(time format string (%c)="%H", seconds (now)=w188) -> (date/time string=w195:string)  [unwired: 1 in]
                    n116 = Concatenate Strings(w197, w200) -> (w160:string)
                    "File Path_Far Field (out)" <- w160
                    n117 = Concatenate Strings(w192, w195) -> (w161:string)
                    "File Path_Near Field (out)" <- w161
                    n118 = String To Path(string=w160) -> (path=w198:path)
                    n119 = String To Path(string=w161) -> (path=w193:path)
                    n120 = call <vilib>:"Check if File or Folder Exists.vi"("path"=w198) -> ("file or folder exists?"=w187:bool, "dup path"=w185:path)  [unwired: 8 in, 1 out]
                    n121 = call <vilib>:"Check if File or Folder Exists.vi"("path"=w193) -> ("file or folder exists?"=w186:bool, "dup path"=w184:path)  [unwired: 8 in, 1 out]
                    n122 = case shown="False" w187 {
                      tunnel: w185 -> [w219 _]
                      tunnel: w160 -> [w218 w220]
                      tunnel: [w218 w220] -> w158
                      frame False {
                        # "new folder"
                        n123 = Create Folder(path (use dialog)=w219) -> ()  [unwired: 2 in, 3 out]
                      }
                      frame True {
                        # "Folder exists\ndo nothing"
                      }
                    }
                    n124 = case shown="False" w186 {
                      tunnel: w184 -> [w216 _]
                      tunnel: w161 -> [w215 w217]
                      tunnel: [w215 w217] -> w159
                      frame False {
                        # "new folder"
                        n125 = Create Folder(path (use dialog)=w216) -> ()  [unwired: 2 in, 3 out]
                      }
                      frame True {
                        # "Folder exists\ndo nothing"
                      }
                    }
                    n126 = Concatenate Strings(w159, "\\Online_Raw_Data.dat" ("string")) -> (w178:string)
                    n127 = Concatenate Strings(w159, "\\Offline_Raw_Data.dat" ("string")) -> (w177:string)
                    n128 = Concatenate Strings(w158, "\\Online_Raw_Data.dat" ("string")) -> (w183:string)
                    n129 = Concatenate Strings(w158, "\\Offline_Raw_Data.dat" ("string")) -> (w182:string)
                    n130 = local read "DataOpen"() -> (w175:bool)
                    n131 = String To Path(string=w183) -> (path=w174:path)
                    n132 = String To Path(string=w182) -> (path=w173:path)
                    n133 = String To Path(string=w178) -> (path=w172:path)
                    n134 = String To Path(string=w177) -> (path=w171:path)
                    n135 = case shown="True" w175 {
                      tunnel: w174 -> [w206 w210]
                      tunnel: [w206 w210] -> w168
                      tunnel: w173 -> [w205 w209]
                      tunnel: [w205 w209] -> w167
                      tunnel: w172 -> [w204 w208]
                      tunnel: [w204 w208] -> w166
                      tunnel: [w203 w207] -> w165
                      tunnel: w171 -> [w203 w207]
                      frame False {
                        # "No files open\ndo nothing"
                      }
                      frame True {
                        # "Close open files"
                        n136 = local read "NF_Off_Ref"() -> (w212:refnum<file>)
                        n137 = local read "NF_On_Ref"() -> (w211:refnum<file>)
                        n138 = local read "FF_Off_Ref"() -> (w214:refnum<file>)
                        n139 = local read "FF_On_Ref"() -> (w213:refnum<file>)
                        n140 = Close File(refnum=w213) -> ()  [unwired: 1 in, 2 out]
                        n141 = Close File(refnum=w214) -> ()  [unwired: 1 in, 2 out]
                        n142 = Close File(refnum=w211) -> ()  [unwired: 1 in, 2 out]
                        n143 = Close File(refnum=w212) -> ()  [unwired: 1 in, 2 out]
                      }
                    }
                    n144 = Open/Create/Replace File(file path (use dialog)=w168, operation (0:open)=T10."open or create") -> (refnum out=w154:refnum<file>)  [unwired: 4 in, 2 out]
                    n145 = Open/Create/Replace File(file path (use dialog)=w167, operation (0:open)=T10."open or create") -> (refnum out=w155:refnum<file>)  [unwired: 4 in, 2 out]
                    n146 = Open/Create/Replace File(file path (use dialog)=w166, operation (0:open)=T10."open or create") -> (refnum out=w156:refnum<file>)  [unwired: 4 in, 2 out]
                    n147 = Open/Create/Replace File(file path (use dialog)=w165, operation (0:open)=T10."open or create") -> (refnum out=w157:refnum<file>)  [unwired: 4 in, 2 out]
                    n148 = Get File Size(file=w154) -> (refnum out=→"FF_On_Ref":refnum<file>, size (in bytes)=→"FF_On_Ptr":i64)  [unwired: 1 in, 1 out]
                    n149 = Get File Size(file=w155) -> (refnum out=→"FF_Off_Ref":refnum<file>, size (in bytes)=→"FF_Off_Ptr":i64)  [unwired: 1 in, 1 out]
                    n150 = Get File Size(file=w156) -> (refnum out=→"NF_On_Ref":refnum<file>, size (in bytes)=→"NF_On_Ptr":i64)  [unwired: 1 in, 1 out]
                    n151 = Get File Size(file=w157) -> (refnum out=→"NF_Off_Ref":refnum<file>, size (in bytes)=→"NF_Off_Ptr":i64)  [unwired: 1 in, 1 out]
                  }
                  frame True {
                    # "Don't need to do anything!"
                  }
                }
              }
              frame #1 {
                # "Writing and plotting retrieved\nweather parameters"
                # "Matlab script goes online and retrieves most recent press, temp, and relative humidity data \nfrom the weather station on the roof of Cobleigh"
                # "Importing the current weather conditions from the COE weather station"
                n152 = disable-structure shown="Disabled" {
                  frame Disabled {
                    n153 = script code="%try\n%s=urlread('http://www.coe.montana.edu/ee/weather/mostCurrentCSV.php');\n%amin=textscan(s,'%s %s %s %s %s %s %s %s %s %s %s %s %s');\n%data=amin{1}{2};\n%[test remain]=strtok(data,',');\n%remain=str2num(remain);\n%press=remain(3)./1000;\n%temp=remain(5);\n%RH=remain(7);\n%catch\npress=.850;\ntemp=20;\nRH=40;\n%end"() -> ()  [unwired: 1 in, 4 out]
                  }
                  frame Enabled {
                  }
                }
                "Temperature (C)" <- "Temperature (C)"
                "Pressure (mb)" <- "Pressure (mbar or hPa)"
                "Relative Humdity (%)" <- 40.0 ("Real")
              }
              frame #2 {
                # "Frame 3: Read, process, and plot online data\nFrame 4: Switch to the offline DBR seed\nFrame 5: Write the data to the folders from Frame 0 of outter sequence"
                # "Frame 0: Read the online wavelength and adjust to locking tolerance if out of range\nFrame 1: Read the output power from the Newport meter, calculate and plot the output pulse energy\nFrame 2: Wait 'Scalar Wait Time' for buffer to clear other wavelength data"
                # "Online"
                n154 = stacked-sequence {
                  frame #0 {
                    # "Read the online wavelength and continue adjusting the online DBR if outside the wavelength tolerance\nuntil it is within tolerance"
                    n155 = while {
                      i -> [w239]
                      stop <- w237 stop-if-true
                      # "Frame 2: Decrement DBR current if above tolerance\nFrame 3: Increment DBR current if below tolerance"
                      # "Frame 0: Read the current wavelength from the wavemeter\nFrame 1: Calculate the difference between desired and actual wavelength"
                      # "Continue reading and adjusting online DBR current until within locking tolerance"
                      n156 = stacked-sequence {
                        tunnel: w239 -> [w241 _ _ _ _]
                        tunnel: [_ _ w248 _ _] -> w238
                        frame #0 {
                          n157 = Equal To 0?(x=w241) -> (x = 0?=w240:bool)
                          n158 = case shown="True" w240 {
                            frame False {
                            }
                            frame True {
                              # "SWITCH to ABSORBING"
                              n159 = Build Array(FALSE ("Boolean")) -> (w242:bool[])
                              n160 = call-poly <vilib>:"DAQmx Write.vi"("task/channels in"=refnum<k21> "BristolWM", "data"=w242) -> ()  [unwired: 11 in, 3 out]
                            }
                          }
                        }
                        frame #1 {
                          # "Read Bristol WM"
                          n161 = local read "Bristol Out"() -> (w245:i32)
                          n162 = dll-call lib="C:/H2O_DIAL/LabVIEW-2012/Bristol WM V2_31b/CLDevIface.dll" fn="CLGetLambdaReading"("devHandle"=w245) -> ("return type"=→"Lambda On Read (nm)":dbl)  [unwired: 4 in, 2 out]
                        }
                        frame #2 {
                          # "If WL difference is within tolerance, stop looping, and illuminate 'Wavelength Lock Online' indicator"
                          # "Calculating the difference between the actual and desired online wavelength"
                          n163 = local read "Lambda On Read (nm)"() -> (w255:dbl)
                          n164 = local read "AB_DIF"() -> (w252:dbl)
                          n165 = Subtract(x=w255, y="Lambda On Set (nm)") -> (x-y=w247:dbl)
                          "WL Difference" <- w247
                          n166 = Multiply(x=-1.0, y=w252) -> (x*y=w253:dbl)
                          n167 = Greater?(x=w247, y=w253) -> (0:w249:bool)
                          n168 = Less?(x=w247, y=w252) -> (x < y?=w250:bool)
                          n169 = And(x=w249, y=w250) -> (x .and. y?=w248:bool)
                          "Wavelength Lock Online" <- w248
                        }
                        frame #3 {
                          # "If the wavelength difference is greater that 0.0002 nm, decrement the \nDBR current by 0.01 mA"
                          n170 = local read "WL Difference"() -> (w258:dbl)
                          n171 = Greater Or Equal?(x=w258, y="AB_DIF") -> (x >= y?=w256:bool)
                          n172 = case shown="True" w256 {
                            frame False {
                              # "Wavelength difference is not greater than 0.0002 nm, do nothing"
                            }
                            frame True {
                              # "Generating a command string\nto decrement the current"
                              # "WL difference is greater than 0.0002 nm,\ndecrement the DBR current by 0.01 mA"
                              n173 = local read "Settings"() -> (w263:T7)
                              n174 = Unbundle By Name(w263) -> ("OnLineLD"=w265:dbl)
                              n175 = Subtract(x=w265, y=3e-06) -> (x-y=w266:dbl)
                              n176 = Bundle By Name(cluster=w263, "OnLineLD"=w266, "Module"=T11."On Line LD") -> (w261:T7)
                              n177 = call "TL_Driver.vi"("Device In"=refnum<visa-resource-name> "ThorLabs", "Commands"=T8."SET", "Settings"=w261) -> ("Readings"=w259:T6)  [unwired: 9 in, 3 out]
                              n178 = local write "Settings"(w261) -> ()
                              n179 = local write "Readings"(w259) -> ()
                            }
                          }
                        }
                        frame #4 {
                          # "If the wavelength difference is less that 0.0002 nm, increment the \nDBR current by 0.01 mA"
                          n180 = local read "WL Difference"() -> (w272:dbl)
                          n181 = local read "AB_DIF"() -> (w270:dbl)
                          n182 = Multiply(x=-1.0, y=w270) -> (x*y=w268:dbl)
                          n183 = Less Or Equal?(x=w272, y=w268) -> (x <= y?=w271:bool)
                          n184 = case shown="True" w271 {
                            frame False {
                              # "WL difference is no <= to -0.0002 nm, do nothing"
                            }
                            frame True {
                              # "WL difference is < -0.0002,\nincrement the DBR current by 0.01 mA"
                              # "Generating a command string\nto decrement the current"
                              n185 = local read "Settings"() -> (w277:T7)
                              n186 = Unbundle By Name(w277) -> ("OnLineLD"=w279:dbl)
                              n187 = Add(x=w279, y=3e-06) -> (x+y=w280:dbl)
                              n188 = Bundle By Name(cluster=w277, "OnLineLD"=w280, "Module"=T11."On Line LD") -> (w274:T7)
                              n189 = call "TL_Driver.vi"("Device In"=refnum<visa-resource-name> "ThorLabs", "Commands"=T8."SET", "Settings"=w274) -> ("Readings"=w273:T6)  [unwired: 9 in, 3 out]
                              n190 = local write "Settings"(w274) -> ()
                              n191 = local write "Readings"(w273) -> ()
                            }
                          }
                        }
                      }
                      n192 = Or(x=w238, y="Cancel online") -> (x .or. y?=w237:bool)
                    }
                  }
                  frame #1 {
                    # "Converting to pulse energy, assumes 5 percent pickoff"
                    # "Reading the Newport Power meter"
                    # "Reading the output power of the laser transmitter from the Newport power meter, once read, convert to corresponding pulse energy and plot"
                    n193 = local read "Newport Device Key"() -> (w286:string)
                    n194 = local read "NewportRef"() -> (w282:refnum<k24>)
                    n195 = Number To Decimal String(number="SampleSize") -> (decimal integer string=w284:string)  [unwired: 1 in]
                    n196 = disable-structure shown="Disabled" {
                      frame Disabled {
                        # "Plotting the online and offling pulse energies"
                        n197 = local read "Online Pulse Energy"() -> (w297:dbl)
                        n198 = local read "Offline Pulse Energy"() -> (w296:dbl)
                        n199 = Bundle("Online Pulse Energy"=w297, "Offline Pulse Energy"=w296) -> (→"Pulse Energy (Micro Joule)":T13)  [unwired: 1 in]
                      }
                      frame Enabled {
                      }
                    }
                    n200 = invoke class="PowerMeterCommands" method="PerformDAQ"(reference=w282, "deviceKey"=w286, "interval"="1", "sampleSize"=w284) -> ("PerformDAQ"=w287:dbl[])  [unwired: 2 in, 5 out]
                    n201 = call-poly <vilib>:"Mean.vi"("X"=w287) -> ("mean"=w285:dbl)  [unwired: 1 out]
                    n202 = Multiply(x=w285, y=1000.0) -> (x*y=w293:dbl)
                    n203 = Divide(x=w293, y=0.05) -> (x/y=w291:dbl)
                    n204 = Divide(x=w291, y="PRF (kHz)") -> (x/y=→"Online Pulse Energy":dbl)
                  }
                  frame #2 {
                    # "Waiting 'Scalar Wait Time'"
                    # "Wait 'Scalar Wait Time' for the next available batch of scalar card data"
                    n205 = Wait (ms)(milliseconds to wait="Scalar Wait Time") -> ()  [unwired: 1 out]
                  }
                  frame #3 {
                    # "convert time per range bin to meters\nand calculate smoothed bins using\nsmoothing range"
                    # "Plotting online cross section and smoothed online data"
                    # "Calculate the bin by bin mean of the data"
                    # "Collect 'Integration Period (Seconds)' number\nof scalar data"
                    # "Reading, processing, and plotting the online data"
                    n206 = local read "Data Reads (number of loops)"() -> (w324:i32)
                    n207 = for {
                      N: w324 -> [_]
                      tunnel: [w345] -> w336 mode=indexing
                      tunnel: [w344] -> w316 mode=indexing
                      # "Scalar Data is retrieved from Global \nVariable that scaler.vi is writing to,"
                      n208 = global read "Scalar_Data.vi" "Scalar Data"() -> (w345:u16[])
                      n209 = global read "Scalar_Data.vi" "Scalar Data  3"() -> (w344:u16[])
                    }
                    n210 = Transpose 2D Array(2D array=w336) -> (transposed array=w340:u16[][])
                    n211 = Transpose 2D Array(2D array=w316) -> (transposed array=w322:u16[][])
                    n212 = for {
                      tunnel: w340 -> [w347] mode=indexing
                      tunnel: [w346] -> w341 mode=indexing
                      n213 = call-poly <vilib>:"Mean.vi"("X"=w347) -> ("mean"=w346:dbl)  [unwired: 1 out]
                    }
                    n214 = for {
                      tunnel: w322 -> [w343] mode=indexing
                      tunnel: [w342] -> w323 mode=indexing
                      n215 = call-poly <vilib>:"Mean.vi"("X"=w343) -> ("mean"=w342:dbl)  [unwired: 1 out]
                    }
                    n216 = local read "bins"() -> (w315:u32)
                    n217 = Array Subset(array=w341, index=1 ("dimension size"), length=w315) -> (w328:dbl[])
                    n218 = Array Subset(array=w323, index=1 ("dimension size"), length=w315) -> (w320:dbl[])
                    n219 = local read "background length"() -> (w305:i32)
                    n220 = local read "background start"() -> (w306:u32)
                    n221 = Array Size(array=w328) -> (size(s)=w325:i32)
                    n222 = Array Size(array=w320) -> (size(s)=w317:i32)
                    n223 = Initialize Array(1.0 ("element"), w325) -> (w327:dbl[])
                    n224 = Initialize Array(1.0 ("element"), w317) -> (w319:dbl[])
                    n225 = Multiply(x=w328, y=w327) -> (x*y=w329:dbl[])
                    "On-Line Bin Readings" <- w329
                    n226 = Multiply(x=w320, y=w319) -> (x*y=w309:dbl[])
                    "On-Line Bin Readings 2" <- w309
                    n227 = local read "Total DIAL Integration Time (Minutes)"() -> (w332:i32)
                    n228 = local read "Time Resolution Per Bin(ns)"() -> (w301:u32)
                    n229 = Array Subset(array=w329, index=w306, length=w305) -> (w338:dbl[])
                    n230 = Array Subset(array=w309, index=w306, length=w305) -> (w311:dbl[])
                    n231 = call-poly <vilib>:"Mean.vi"("X"=w338) -> ("mean"=w337:dbl)  [unwired: 1 out]
                    n232 = call-poly <vilib>:"Mean.vi"("X"=w311) -> ("mean"=w312:dbl)  [unwired: 1 out]
                    n233 = Divide(x=w332, y=w324) -> (x/y=w330:dbl)
                    n234 = local read "Index"() -> (w310:i32)
                    n235 = Subtract(x=w329, y=w337) -> (x-y=w334:dbl[])
                    n236 = Subtract(x=w309, y=w312) -> (x-y=w313:dbl[])
                    n237 = To Double Precision Float(number=w301) -> (double precision float=w302:dbl)
                    n238 = Multiply(x=w330, y=60.0) -> (x*y=w307:dbl)
                    n239 = Multiply(x=w302, y=0.15) -> (x*y=w304:dbl)
                    n240 = call "Ring Buffer Online Far.vi"("Index"=w310, "Profiles to Average"=w307, "Input Array"=w334) -> ("AvgArray"=w333:dbl[])  [unwired: 7 in, 1 out]
                    n241 = call "Ring Buffer Online Near.vi"("Index"=w310, "Profiles to Average"=w307, "Input Array"=w313) -> ("AvgArray"=w314:dbl[])  [unwired: 7 in, 1 out]
                    n242 = Divide(x="Smoothing Range", y=w304) -> (x/y=w299:dbl)
                    "Smoothed Bins" <- w299
                    n243 = call "Smooth Arrray.vi"("smooth size"=w299, "Raw Array"=w333) -> ("Smoothed Array"=→"On-Line  Smoothed":dbl[])  [unwired: 9 in]
                    n244 = call "Smooth Arrray.vi"("smooth size"=w299, "Raw Array"=w314) -> ("Smoothed Array"=→"On-Line Smoothed 2":dbl[])  [unwired: 9 in]
                    n245 = disable-structure shown="Disabled" {
                      frame Disabled {
                        n246 = script code="format long;\ncounts=sum(Online);\nif counts >=0.5e6\ntime=time;\nelse\ntime=time\nend"() -> ()  [unwired: 3 in, 2 out]
                      }
                      frame Enabled {
                      }
                    }
                  }
                  frame #4 {
                    # "Toggling the Agiltron switch to the offline DBR seed laser"
                    n247 = disable-structure shown="Disabled" {
                      frame Disabled {
                        n248 = flat-sequence {
                          frame #0 {
                            # "Second one"
                            # "Command the switch to switch to position 2\ncorresponding to the offline DBR"
                            # "Hex string command \ncorrespond to offline"
                            n249 = VISA Write(VISA resource name="Switch Comm Port", write buffer="\u0001\u0012\u0000\u0001") -> ()  [unwired: 1 in, 3 out]
                          }
                        }
                      }
                      frame Enabled {
                      }
                    }
                  }
                  frame #5 {
                    # "Save the recently collected online data if 'Save Data?' is true"
                    n250 = case shown="True" "Save Data?" {
                      frame False {
                        # "'Save Data?' is false, do nothing"
                      }
                      frame True {
                        # "'Save Data?' is true, save onfline data to the Data Disk"
                        # "Write only one copy of data at this time"
                        # "Retrieve Julian Date"
                        n251 = local read "Readings"() -> (w358:T6)
                        n252 = local read "Time Resolution Per Bin(ns)"() -> (w356:u32)
                        n253 = local read "Number of Accumulates"() -> (w354:u32)
                        n254 = local read "Number of Bins"() -> (w355:u32)
                        n255 = local write "DataOpen"(TRUE ("DataOpen")) -> ()
                        n256 = local read "Lambda On Read (nm)"() -> (w380:dbl)
                        n257 = local read "On-Line Bin Readings 2"() -> (w378:dbl[])
                        n258 = local read "On-Line Bin Readings"() -> (w382:dbl[])
                        n259 = local read "Online Pulse Energy"() -> (w379:dbl)
                        n260 = Unbundle By Name(w358) -> ("OnLineLD"=w357:dbl)
                        n261 = To Double Precision Float(number=w356) -> (double precision float=w353:dbl)
                        n262 = To Double Precision Float(number=w355) -> (double precision float=w352:dbl)
                        n263 = To Double Precision Float(number=w354) -> (double precision float=w351:dbl)
                        n264 = call "Julian_Date_2.vi"() -> ("Julian Date"=w381:dbl)  [unwired: 11 in]
                        n265 = Build Array (concatenate)(w381, w380, w357, w379, w353, w352, w351, w382) -> (w373:dbl[])
                        n266 = Build Array (concatenate)(w381, w380, w357, w379, w353, w352, w351, w378) -> (w363:dbl[])
                        n267 = local read "NF_On_Ref"() -> (w361:refnum<file>)
                        n268 = local read "FF_On_Ref"() -> (w377:refnum<file>)
                        n269 = local read "NF_On_Ptr"() -> (w362:i64)
                        n270 = local read "FF_On_Ptr"() -> (w376:i64)
                        n271 = Set File Position(offset (in bytes) (0)=w376, refnum=w377) -> (refnum out=w374:refnum<file>, error out=w371:errorcluster)  [unwired: 2 in]
                        n272 = Set File Position(offset (in bytes) (0)=w362, refnum=w361) -> (refnum out=w367:refnum<file>, error out=w365:errorcluster)  [unwired: 2 in]
                        n273 = Write to Binary File(file (use dialog)=w367, data=w363, error in=w365, 5:FALSE ("prepend array or string size? (T)")) -> (refnum out=w366:refnum<file>, error out=w364:errorcluster)  [unwired: 2 in, 1 out]
                        n274 = Write to Binary File(file (use dialog)=w374, data=w373, error in=w371, 5:FALSE ("prepend array or string size? (T)")) -> (refnum out=w372:refnum<file>, error out=w370:errorcluster)  [unwired: 2 in, 1 out]
                        n275 = Get File Position(4:w364, 7:w366) -> (2:w360:i64)  [unwired: 2 out]
                        n276 = Get File Position(4:w370, 7:w372) -> (2:w369:i64)  [unwired: 2 out]
                        n277 = local write "NF_On_Ptr"(w360) -> ()
                        n278 = local write "FF_On_Ptr"(w369) -> ()
                      }
                    }
                  }
                }
              }
              frame #3 {
                # "Frame 3: Read offline data, calculate aerosol data, and plot offline and normalized relative backscatter\nFrame 4: Swich to online DBR\nFrame 5: Save the offline data and related information"
                # "Frame 0: Read the offline wavelength and lock if necessary, though code is not finished to do so\nFrame 1: Read the output power from the Newport power meter\nFrame 2: Wait 'Scalar Wait Time' for buffers to clear of online contiminated data"
                # "offline"
                n279 = stacked-sequence {
                  frame #0 {
                    # "Every 60 data collection cycles, read the offline DBR wavelength, and if outside of wavelength tolerance, adjust DBR current until within tolerance"
                    n280 = local read "L_Count"() -> (w384:i32)
                    n281 = Quotient & Remainder(x=w384, y=60.0) -> (x-y*floor(x/y)=w385:dbl)  [unwired: 1 out]
                    n282 = Equal To 0?(x=w385) -> (x = 0?=w383:bool)
                    n283 = case shown="True" w383 {
                      frame False {
                      }
                      frame True {
                        n284 = while {
                          i -> [w390]
                          stop <- w388 stop-if-true
                          # "Frame 5 Increment ofline DBR current if below tolerance\nFrame 6: update ILX settings to front pannel"
                          # "Frame 3: Calculating the wavelength difference\nFrame 4:Decrement offline DBR current if above tolerance"
                          # "Frame 0: Read the offline laser wavelength (settle if t=0)"
                          n285 = stacked-sequence {
                            tunnel: w390 -> [w392 _ _ _ _]
                            tunnel: [_ _ w402 _ _] -> w389
                            frame #0 {
                              n286 = Equal To 0?(x=w392) -> (x = 0?=w391:bool)
                              n287 = case shown="True" w391 {
                                frame False {
                                }
                                frame True {
                                # "SWITCH to NON-ABSORBING and wait to settle"
                                n288 = Build Array(TRUE ("Boolean")) -> (w397:bool[])
                                n289 = call-poly <vilib>:"DAQmx Write.vi"("task/channels in"=refnum<k21> "BristolWM", "data"=w397) -> ()  [unwired: 11 in, 3 out]
                                n290 = call "TL_Driver.vi"("Device In"=refnum<visa-resource-name> "ThorLabs", "Commands"=T8."Read_Status") -> ("Readings"=w395:T6)  [unwired: 10 in, 3 out]
                                n291 = local write "Readings"(w395) -> ()
                                n292 = Wait (ms)(milliseconds to wait=u32 3200) -> ()  [unwired: 1 out]
                                }
                              }
                            }
                            frame #1 {
                              # "Read Bristol WM"
                              n293 = local read "Bristol Out"() -> (w400:i32)
                              n294 = dll-call lib="C:/H2O_DIAL/LabVIEW-2012/Bristol WM V2_31b/CLDevIface.dll" fn="CLGetLambdaReading"("devHandle"=w400) -> ("return type"=→"Lambda Off Read (nm)":dbl)  [unwired: 4 in, 2 out]
                            }
                            frame #2 {
                              # "Once locked, stop looping and illuminate 'Wavelength Lock Offline'"
                              # "While loop continues locking process until the wavelength is within tolerance"
                              # "Calculating the difference between the actual and desired \noffline wavelength"
                              n295 = local read "Lambda Off Read (nm)"() -> (w410:dbl)
                              n296 = Subtract(x=w410, y="Lambda Off Set (nm)") -> (x-y=w403:dbl)
                              "WL Difference off" <- w403
                              n297 = local read "NONAB_DIF"() -> (w407:dbl)
                              n298 = Multiply(x=-1.0, y=w407) -> (x*y=w408:dbl)
                              n299 = Greater?(x=w403, y=w408) -> (0:w404:bool)
                              n300 = Less?(x=w403, y=w407) -> (x < y?=w405:bool)
                              n301 = And(x=w404, y=w405) -> (x .and. y?=w402:bool)
                              "Wavelength Lock Offline" <- w402
                              n302 = case shown="True" w402 {
                                frame False {
                                }
                                frame True {
                                # "SWITCH back to ABSORBING and wait to settle"
                                n303 = Build Array(FALSE ("Boolean")) -> (w412:bool[])
                                n304 = call-poly <vilib>:"DAQmx Write.vi"("task/channels in"=refnum<k21> "BristolWM", "data"=w412) -> ()  [unwired: 11 in, 3 out]
                                n305 = Wait (ms)(milliseconds to wait=u32 3000) -> ()  [unwired: 1 out]
                                }
                              }
                            }
                            frame #3 {
                              # "Would adjust the offline wavelength if code was finished"
                              n306 = local read "WL Difference off"() -> (w417:dbl)
                              n307 = Greater Or Equal?(x=w417, y="NONAB_DIF") -> (x >= y?=w415:bool)
                              n308 = case shown="True" w415 {
                                frame False {
                                # "WL difference is not out of range, do nothing"
                                }
                                frame True {
                                # "Generating a command string\nto decrement the current"
                                # "WL difference is greater than 0.0002 nm,\ndecrement the DBR current by 0.01 mA"
                                # "WL difference is out of range, this is where you would decrement\nthe laser current"
                                n309 = local read "Settings"() -> (w422:T7)
                                n310 = Unbundle By Name(w422) -> ("OffLineLD"=w423:dbl)
                                n311 = Subtract(x=w423, y=3e-06) -> (x-y=w424:dbl)
                                n312 = Bundle By Name(cluster=w422, "OffLineLD"=w424, "Module"=T11."Off Line LD") -> (w421:T7)
                                n313 = call "TL_Driver.vi"("Device In"=refnum<visa-resource-name> "ThorLabs", "Commands"=T8."SET", "Settings"=w421) -> ("Readings"=w418:T6)  [unwired: 9 in, 3 out]
                                n314 = local write "Settings"(w421) -> ()
                                n315 = local write "Readings"(w418) -> ()
                                }
                              }
                            }
                            frame #4 {
                              # "This is where you would increment the offline current if below tolerance"
                              n316 = local read "NONAB_DIF"() -> (w428:dbl)
                              n317 = local read "WL Difference off"() -> (w431:dbl)
                              n318 = Multiply(x=-1.0, y=w428) -> (x*y=w427:dbl)
                              n319 = Less Or Equal?(x=w431, y=w427) -> (x <= y?=w430:bool)
                              n320 = case shown="True" w430 {
                                frame False {
                                # "WL difference is not outisde tolerance, do nothing"
                                }
                                frame True {
                                # "Generating a command string\nto decrement the current"
                                # "WL difference is less than 0.0002 nm,\nincrement the DBR current by 0.01 mA"
                                # "Incrementing the current if below tolerance"
                                n321 = local read "Settings"() -> (w435:T7)
                                n322 = Unbundle By Name(w435) -> ("OffLineLD"=w437:dbl)
                                n323 = Add(x=w437, y=3e-06) -> (x+y=w438:dbl)
                                n324 = Bundle By Name(cluster=w435, "OffLineLD"=w438, "Module"=T11."Off Line LD") -> (w436:T7)
                                n325 = call "TL_Driver.vi"("Device In"=refnum<visa-resource-name> "ThorLabs", "Commands"=T8."SET", "Settings"=w436) -> ("Readings"=w432:T6)  [unwired: 9 in, 3 out]
                                n326 = local write "Settings"(w436) -> ()
                                n327 = local write "Readings"(w432) -> ()
                                }
                              }
                            }
                          }
                          n328 = Or(x=w389, y="Cancel Offline") -> (x .or. y?=w388:bool)
                        }
                      }
                    }
                  }
                  frame #1 {
                    # "Reading the power meter"
                    # "Updating the pulse energy plot"
                    # "Converting to pulse energy"
                    # "Reading the offline output power, converting to pulse energy,  and updating the Pulse energy plot"
                    n329 = local read "SampleSize"() -> (w444:i32)
                    n330 = local read "Newport Device Key"() -> (w445:string)
                    n331 = local read "Online Pulse Energy"() -> (w451:dbl)
                    n332 = local read "Offline Pulse Energy"() -> (w450:dbl)
                    n333 = local read "NewportRef"() -> (w442:refnum<k24>)
                    n334 = Number To Decimal String(number=w444) -> (decimal integer string=w446:string)  [unwired: 1 in]
                    n335 = invoke class="PowerMeterCommands" method="PerformDAQ"(reference=w442, "deviceKey"=w445, "interval"="1", "sampleSize"=w446) -> ("PerformDAQ"=w447:dbl[])  [unwired: 2 in, 5 out]
                    n336 = Bundle("Online Pulse Energy"=w451, "Offline Pulse Energy"=w450) -> (w449:T13)  [unwired: 1 in]
                    n337 = local write "Pulse Energy (Micro Joule)"(w449) -> ()
                    n338 = call-poly <vilib>:"Mean.vi"("X"=w447) -> ("mean"=w443:dbl)  [unwired: 1 out]
                    n339 = local read "PRF (kHz)"() -> (w441:dbl)
                    n340 = Multiply(x=w443, y=1000.0) -> (x*y=w455:dbl)
                    n341 = Divide(x=w455, y=0.05) -> (x/y=w453:dbl)
                    n342 = Divide(x=w453, y=w441) -> (x/y=→"Offline Pulse Energy":dbl)
                  }
                  frame #2 {
                    # "Wait 'Scalar Wait Time' for buffers to clear of online contiminated offline data"
                    n343 = disable-structure shown="Disabled" {
                      frame Disabled {
                        # "Wait 'Scalar Wait Time'"
                        n344 = local read "Scalar Wait Time"() -> (w457:u32)
                        n345 = Wait (ms)(milliseconds to wait=w457) -> ()  [unwired: 1 out]
                      }
                      frame Enabled {
                      }
                    }
                  }
                  frame #3 {
                    w489 = 1 ("dimension size")
                    w493 = 1
                    # "Plotting the normalized relative \nbackscatter"
                    # "Calculating the normalized relative backscatter"
                    # "Calculating/Plotting smoothed data,\ncross sections etc."
                    # "Pick off data with\nout header"
                    # "Calculate mean bin by bin mean"
                    # "Reading in 'Integration Period (Seconds)' of data"
                    # "Read the offline data from the scalar card, perform smoothing, calculate normalized relative backscatter, and plot"
                    # "File path in MATLAB script is of old dial is:\nF:\\Micropulse DIAL\\Micropulse DIAL Matlab\\\nFinal Overlap Function.mat')];"
                    # "Collects Data From Card,\nSends It To The Chart,\nAnd Saves A Copy As A\nFile If Option Selected On\nFront Panel"
                    n346 = for {
                      N: "Data Reads (number of loops)" -> [_]
                      tunnel: [w527] -> w524 mode=indexing
                      tunnel: [w526] -> w506 mode=indexing
                      # "Read in latest scalar card data from \n'Scalar Data' global variable that \nscaler.vi is writing to, then wait 1 sec\nfor next batch of data"
                      n347 = global read "Scalar_Data.vi" "Scalar Data  4"() -> (w526:u16[])
                      n348 = global read "Scalar_Data.vi" "Scalar Data  2"() -> (w527:u16[])
                    }
                    n349 = local read "Total DIAL Integration Time (Minutes)"() -> (w515:i32)
                    n350 = Divide(x=w515, y="Data Reads (number of loops)") -> (x/y=w513:dbl)
                    n351 = local read "Total Aerosol Integration Time (Minutes)"() -> (w517:dbl)
                    n352 = local read "background length"() -> (w461:i32)
                    n353 = Multiply(x=w513, y=60.0) -> (x*y=w499:dbl)
                    n354 = local read "background start"() -> (w462:u32)
                    n355 = Transpose 2D Array(2D array=w524) -> (transposed array=w523:u16[][])
                    n356 = Transpose 2D Array(2D array=w506) -> (transposed array=w505:u16[][])
                    n357 = Divide(x=w517, y="Data Reads (number of loops)") -> (x/y=w518:dbl)
                    n358 = for {
                      tunnel: w523 -> [w531] mode=indexing
                      tunnel: [w530] -> w525 mode=indexing
                      tunnel: w505 -> [w529] mode=indexing
                      tunnel: [w528] -> _ mode=indexing
                      tunnel: [w528] -> w502 mode=indexing
                      n359 = call-poly <vilib>:"Mean.vi"("X"=w531) -> ("mean"=w530:dbl)  [unwired: 1 out]
                      n360 = call-poly <vilib>:"Mean.vi"("X"=w529) -> ("mean"=w528:dbl)  [unwired: 1 out]
                    }
                    n361 = local read "bins"() -> (w490:u32)
                    n362 = Multiply(x=w518, y=60.0) -> (x*y=w480:dbl)
                    n363 = Array Subset(array=w502, index=w489, length=w490) -> (w503:dbl[])
                    "Off-Line Bin Readings 2" <- w503
                    n364 = Array Subset(array=w525, index=w489, length=w490) -> (w501:dbl[])
                    "Off-Line  Bin Readings" <- w501
                    n365 = Array Subset(array=w503, index=w462, length=w461) -> (w504:dbl[])
                    n366 = Array Subset(array=w501, index=w462, length=w461) -> (w522:dbl[])
                    n367 = local read "Smoothed Bins"() -> (w458:dbl)
                    n368 = call-poly <vilib>:"Mean.vi"("X"=w504) -> ("mean"=w468:dbl)  [unwired: 1 out]
                    n369 = call-poly <vilib>:"Mean.vi"("X"=w522) -> ("mean"=w469:dbl)  [unwired: 1 out]
                    n370 = local read "Index"() -> (w479:i32)
                    n371 = Subtract(x=w503, y=w468) -> (x-y=w481:dbl[])
                    n372 = Subtract(x=w501, y=w469) -> (x-y=w497:dbl[])
                    n373 = call "Ring Buffer Offline Far.vi"("Index"=w479, "Profiles to Average"=w499, "Input Array"=w497) -> ("AvgArray"=w520:dbl[], "RingBufferOut"=→"RingBuffer offline far":dbl[][])  [unwired: 7 in]
                    n374 = call "Ring Buffer Aerosol Far.vi"("Index"=w479, "Profiles to Average"=w480, "Input Array"=w497) -> ("AvgArray"=w516:dbl[], "RingBufferOut"=→"RingBuffer aerosol far":dbl[][])  [unwired: 7 in]
                    n375 = call "Ring Buffer Offline Near.vi"("Index"=w479, "Profiles to Average"=w499, "Input Array"=w481) -> ("AvgArray"=w500:dbl[], "RingBufferOut"=→"RingBuffer offline near":dbl[][])  [unwired: 7 in]
                    n376 = call "Ring Buffer Aerosol Near.vi"("Index"=w479, "Profiles to Average"=w480, "Input Array"=w481) -> ("AvgArray"=w477:dbl[], "RingBufferOut"=→"RingBuffer aerosol near":dbl[][])  [unwired: 7 in]
                    n377 = Reshape Array(w497, w489, w490) -> (→"raw counts":dbl[][])
                    n378 = Reshape Array(w481, w489, w490) -> (→"raw counts near":dbl[][])
                    n379 = call "Smooth Arrray.vi"("smooth size"=w458, "Raw Array"=w520) -> ("Smoothed Array"=→"Off-Line Smoothed":dbl[])  [unwired: 9 in]
                    n380 = call "Smooth Arrray.vi"("smooth size"=w458, "Raw Array"=w516) -> ("Smoothed Array"=w488:dbl[])  [unwired: 9 in]
                    "Aerosol Smoothed" <- w488
                    n381 = call "Smooth Arrray.vi"("smooth size"=w458, "Raw Array"=w500) -> ("Smoothed Array"=→"Off-Line Smoothed 2":dbl[])  [unwired: 9 in]
                    n382 = call "Smooth Arrray.vi"("smooth size"=w458, "Raw Array"=w477) -> ("Smoothed Array"=w460:dbl[])  [unwired: 9 in]
                    "Aerosol Smoothed 2" <- w460
                    n383 = local read "Number of Accumulates"() -> (w464:u32)
                    n384 = local read "Temperature (C)"() -> (w512:dbl)
                    n385 = local read "Pressure (mb)"() -> (w511:dbl)
                    n386 = script code="%accum_num=10000;     % scaler card setting number of accumulations\nt_bin = 500e-9                 % scaler card setting time per bin\n%t_d = 37.3e-9;                % APD dead time from spec sheet\n\n% conversion from accumulated counts to count rate  (c/s)\nc_convert = 1./t_bin./accum_num;\nCR_far = p_raw_far.*c_convert;\nCR_near = p_raw_near.*c_convert;\nCR_total_far = (p_raw_far+b_far).*c_convert;\nCR_total_near = (p_raw_near+b_near).*c_convert;\nb_CR_far =b_far.*c_convert;\nb_CR_near =b_near.*c_convert;\n\n% create a range array\nsize_p =  size(p_raw_far,2);\nr = (75:75:size_p*75)./1e3; \n    \n%APD correction factor\n D_far = 1./(1-(t_d*CR_total_far));\n D_near = 1./(1-(t_d*CR_total_near));\n\n %Calculating normalize relative backscatter profile\n nrb_far = CR_far.*D_far.*r.^2./E.*1e-6;\n nrb_near = CR_near.*D_near.*r.^2./E.*1e-6;"("E"=6.0 ("Real"), "temp"=w512, "press"=w511, "p_raw_far"=w488, "b_far"=w469, "b_near"=w468, "p_raw_near"=w460, "accum_num"=w464, "t_d"="dead time") -> ("nrb_far"=w483:cdb[], "D_far"=w474:dbl[], "nrb_near"=w482:cdb[], "D_near"=w473:dbl[], "b_CR_far"=w466:dbl, "b_CR_near"=w465:dbl)  [unwired: 1 in, 1 out]
                    n387 = local read "bins"() -> (w492:u32)
                    n388 = local read "Altitude Array (km)"() -> (w485:dbl[])
                    n389 = Bundle(w466, w465) -> (→"?":cluster{dbl, dbl})  [unwired: 1 in]
                    n390 = Build Array(w483, w482) -> (w487:cdb[][])
                    n391 = Build Array(w474, w473) -> (w472:dbl[][])
                    n392 = Reshape Array(w482, w493, w492) -> (→"NRB 2":cdb[][])
                    n393 = Reshape Array(w483, w493, w492) -> (→"NRB":cdb[][])
                    n394 = Build Array(w485, w485) -> (w484:dbl[][])
                    n395 = call "Convert to Dynamic Data7"("2D Array"=w472) -> ("Dynamic Data Type"=w471:dynamicdata)  [unwired: 3 in]
                    n396 = call "Convert to Dynamic Data3"("2D Array"=w487) -> ("Dynamic Data Type"=w486:dynamicdata)  [unwired: 3 in]
                    n397 = call "Convert to Dynamic Data4"("2D Array"=w484) -> ("Dynamic Data Type"=w475:dynamicdata)  [unwired: 3 in]
                    n398 = call "Build XY Graph2"("Y Input"=w475, "X Input"=w486) -> ("XY Graph"=→"NRB plot":cluster{"Y":dbl[], "Y":dbl[]}[])  [unwired: 3 in, 6 out]
                    n399 = call "Build XY Graph4"("Y Input"=w475, "X Input"=w471) -> ("XY Graph"=→"Correction":cluster{"Y":dbl[], "Y":dbl[]}[])  [unwired: 3 in, 6 out]
                  }
                  frame #4 {
                    # "REPLACE WITH NEW AGILTRON TASK!"
                    # "Toggle Agiltron switch to online DBR"
                    n400 = disable-structure shown="Disabled" {
                      frame Disabled {
                        # "ABSORBING"
                        n401 = flat-sequence {
                          frame #0 {
                            # "Third one"
                            # "Command the switch to switch to position 1\ncorresponding to the online DBR"
                            # "Hex string command \ncorrespond to online"
                            n402 = local read "Switch Comm Port"() -> (w535:refnum<visa-resource-name>)
                            n403 = VISA Write(VISA resource name=w535, write buffer="\u0001\u0012\u0000\u0002") -> ()  [unwired: 1 in, 3 out]
                          }
                        }
                        n404 = Build Array(FALSE ("Boolean")) -> (w534:bool[])
                        n405 = call-poly <vilib>:"DAQmx Write.vi"("task/channels in"=refnum<k21> "AgiltronSwitch", "data"=w534) -> ()  [unwired: 11 in, 3 out]
                      }
                      frame Enabled {
                      }
                    }
                  }
                  frame #5 {
                    # "If 'Save Data?' is true, save all relavant offline info"
                    n406 = local read "Save Data?"() -> (w537:bool)
                    n407 = case shown="True" w537 {
                      frame False {
                        # "'Save Data?' is false, do nothing"
                      }
                      frame True {
                        # "Write only one data file at this time"
                        # "Retrive Julian Date"
                        # "'Save Data?' is true, save offline data to the Data Disk"
                        n408 = local read "Readings"() -> (w539:T6)
                        n409 = local read "Off-Line Bin Readings 2"() -> (w558:dbl[])
                        n410 = local read "Lambda Off Read (nm)"() -> (w560:dbl)
                        n411 = local read "Off-Line  Bin Readings"() -> (w565:dbl[])
                        n412 = local read "Relative Humdity (%)"() -> (w564:dbl)
                        n413 = local read "Offline Pulse Energy"() -> (w561:dbl)
                        n414 = local read "Temperature (C)"() -> (w562:dbl)
                        n415 = Unbundle By Name(w539) -> ("OffLineLD"=w538:dbl)
                        n416 = local read "Pressure (mb)"() -> (w563:dbl)
                        n417 = call "Julian_Date_2.vi"() -> ("Julian Date"=w559:dbl)  [unwired: 11 in]
                        n418 = Build Array (concatenate)(w559, w560, w538, w561, w562, w563, w564, w565) -> (w544:dbl[])
                        n419 = Build Array (concatenate)(w559, w560, w538, w561, w562, w563, w564, w558) -> (w541:dbl[])
                        n420 = local read "FF_Off_Ref"() -> (w546:refnum<file>)
                        n421 = local read "NF_Off_Ref"() -> (w543:refnum<file>)
                        n422 = local read "FF_Off_Ptr"() -> (w545:i64)
                        n423 = local read "NF_Off_Ptr"() -> (w542:i64)
                        n424 = Set File Position(offset (in bytes) (0)=w545, refnum=w546) -> (refnum out=w557:refnum<file>, error out=w555:errorcluster)  [unwired: 2 in]
                        n425 = Set File Position(offset (in bytes) (0)=w542, refnum=w543) -> (refnum out=w553:refnum<file>, error out=w551:errorcluster)  [unwired: 2 in]
                        n426 = Write to Binary File(file (use dialog)=w557, data=w544, error in=w555, 5:FALSE ("prepend array or string size? (T)")) -> (refnum out=w556:refnum<file>, error out=w554:errorcluster)  [unwired: 2 in, 1 out]
                        n427 = Write to Binary File(file (use dialog)=w553, data=w541, error in=w551, 5:FALSE ("prepend array or string size? (T)")) -> (refnum out=w552:refnum<file>, error out=w550:errorcluster)  [unwired: 2 in, 1 out]
                        n428 = Get File Position(4:w554, 7:w556) -> (2:w547:i64)  [unwired: 2 out]
                        n429 = Get File Position(4:w550, 7:w552) -> (2:w540:i64)  [unwired: 2 out]
                        n430 = local write "FF_Off_Ptr"(w547) -> ()
                        n431 = local write "NF_Off_Ptr"(w540) -> ()
                      }
                    }
                  }
                }
              }
              frame #4 {
                n432 = First Call?() -> (First Call?: T/F=w568:bool)
                n433 = Or(x="calculate absorption cross sections", y=w568) -> (x .or. y?=w566:bool)
                n434 = case shown="True" w566 {
                  frame False {
                  }
                  frame True {
                    # "calculate absorption cross sections from HITRAN data base"
                    n435 = local read "Off-Line Smoothed"() -> (w569:dbl[])
                    n436 = local read "Lambda On Read (nm)"() -> (w572:dbl)
                    n437 = local read "Lambda Off Set (nm)"() -> (w575:dbl)
                    n438 = local read "Temperature (C)"() -> (w573:dbl)
                    n439 = local read "Pressure (mb)"() -> (w574:dbl)
                    n440 = script code="hitran = dlmread('C:\\H2O_DIAL\\LabVIEW-2012\\Micropulse DIAL Matlab\\815nm_841nm_HITRAN_2008.csv', ',',[1 1 1676 8]);\n%hitran = dlmread('C:\\H2O_DIAL\\LabVIEW-2012\\Micropulse DIAL Matlab\\824nm_841nm_H2O_Spectral_Calc.csv', ',',[1 1 1209 7]);\n\n\n\n%Range vector in meters\nrange = ([75:75:size(Online,2)*75]);\n\nif lambda< 828\nlambda=828.195;\nelse\nlambda=lambda;\nend;\n\n%%\n\n%Voigt profile calculation\nWNmin = 1/(828+4)*1e7;  % 832.0 nm converted to wavenumber\nWNmax = 1/(828-4)*1e7;  % 824.0 nm converted to wavenumber\n\n%Find lines from WNmin to WNmax to calculate voigt profile\nline_indices = hitran(1:size(hitran,1),1)>WNmin & hitran(1:size(hitran,1),1)<WNmax;\n\nline = double(hitran(line_indices, 1:size(hitran,2)));\n\n%Calculate temperature and pressure profile\nT0 = 273+25; % surface temperature\nT0 = 273+T0_C;\nT = T0-0.0065.*range; % set to match the sounding\n\n% pressure in atmospheres\nP0  = 0.83; % surface pressure\nP0  = P0_mb/1000*0.986; %pressure in mb converted to atm\nP = P0.*(T0./T).^-5.5;   % set this value to match sounding\n\nT00 = 296;              % HITRAN reference temperature [K]\nP00 = 1;                % HITRAN reference pressure [atm]\nnu0_0 = line(:,1);      % absorption line center wavenumber from HITRAN [cm^-1]\nS0 = line(:,2);         % initial linestrength from HITRAN [cm^-1/(mol*cm^-2)]   \ngammal0 = line(:,4);    % air-broadened halfwidth at T_ref and P_ref from HITRAN [cm^-1/atm]\ngamma_s = line(:,5);    % self-broadened halfwidth at T_ref and P_ref from HITRAN [cm^-1/atm]\nE = line(:,6);          % ground state transition energy from HITRAN [cm^-1]  \nalpha = line(:,7);      % linewidth temperature dependence factor from HITRAN\ndelta = line(:,8);      % pressure shift from HiTRAN [cm^-1 atm^-1]\n\nnu_on = 1/(lambda)*1e7;\nnu_off = 1/(lambda_off)*1e7;\n\nfor i = 1:size(Online,2); % calculate the absorption cross section at each range\n  \n    nu0 = nu0_0+delta.*(P(i)./P00); % unclear if it should be Pi/P00  \n    gammal = gammal0.*(P(i)./P00).*((T00./T(i)).^alpha);    %Calculate Lorentz lineweidth at P(i) and T(i)\n\n    const.m = 18.015E-3./6.022E23; % mass of a single water molecule\n    const.k_B = 1.3806488e-23; % (J/K)\n    const.c = 299792458; % (m/s) (exact)\n \n    gammad = (nu0).*((2.0.*const.k_B.*T(i).*log(2.0))./(const.m.*const.c^2)).^(0.5);  %Calculate HWHM Doppler linewidth at T(i)\n     \n    % term 1 in the Voigt profile\n    y = (gammal./gammad).*((log(2.0)).^(0.5));\n    \n    % term 2 in the Voigt profile\n    x_on = ((nu_on-nu0)./gammad).*(log(2.0)).^(0.5);\n    x_off = ((nu_off-nu0)./gammad).*(log(2.0)).^(0.5);\n    \n    %setting up Voigt convolution\n    t = (-(size(line,1))/2:1:size(line,1)/2-1); %set up the integration spectral step size\n    t = repmat(t',1,length(x_on))';\n    x_on = repmat(x_on,1,length(t));\n    x_off = repmat(x_off,1,length(t));\n    y = repmat(y,1,length(t));\n    f_on = (exp(-t.^2.0))./(y.^2.0+(x_on-t).^2.0);  % combined Voigt term 1 and 2\n    f_off = (exp(-t.^2.0))./(y.^2.0+(x_off-t).^2.0);\n    %Voigt integration over all of the lines at the on and offline locations\n    z_on = trapz(t(1,:),f_on,2);\n    z_off =  trapz(t(1,:),f_off,2);\n    integral_on = z_on;\n    integral_off = z_off;\n    %Calculate linestrength at temperature T\n    S = S0.*((T00./T(i)).^(1.5)).*exp(1.439.*E.*((1./T00)-(1./T(i))));\n \n    %Calculate the Voigt profile\n    K_on = (y(:,1)./pi).*integral_on;\n    K_off = (y(:,1)./pi).*integral_off;\n    \n    %Calculate the Voigt profile absorption cross section [cm^2]\n    sigmav_on = S.*(1./gammad).*(((log(2.0))./pi).^(0.5)).*K_on; %.*far_wing_on;\n    sigmav_off = S.*(1./gammad).*(((log(2.0))./pi).^(0.5)).*K_off; %.*far_wing_off;\n    \n    %Sum contributions from all of the surrounding lines\n    sigma_on_total(i) = sum(sigmav_on);\n    sigma_off_total(i) = sum(sigmav_off);\n    \nend;"("lambda"=w572, "lambda_off"=w575, "P0_mb"=w574, "T0_C"=w573, "Online"=w569) -> ("sigma_on_total"=→"sigma_on_total":dbl[], "sigma_off_total"=→"sigma_off_total":dbl[])  [unwired: 1 in, 1 out]
                  }
                }
              }
              frame #5 {
                w586 = 1
                # "normalization factor\nfrom 300 to 450m"
                # "OPTICAL DEPTH PLOT"
                # "new rainbow color bar display"
                # "Data Processing Far Channel"
                # "new rainbow color bar display"
                # "Calculating the range resolved water vapor number density and plotting"
                n441 = local read "sigma_off_total"() -> (w609:dbl[])
                n442 = local read "sigma_on_total"() -> (w606:dbl[])
                n443 = local read "On-Line  Smoothed"() -> (w584:dbl[])
                n444 = local read "Off-Line Smoothed"() -> (w583:dbl[])
                n445 = local read "Off-Line Smoothed 2"() -> (w607:dbl[])
                n446 = local read "On-Line Smoothed 2"() -> (w608:dbl[])
                n447 = script code="%Time averaging in seconds.  180 Seconds =3 minutes\ntemporal_average = 180;\n\n%Spatial averaging in bins.  2 bins = 150 meters\nspatial_average = 2;\n\n%Creating r and r+deltar vectors..this can also be acsomplished using the\n%diff command\np_oni = Online(:,1:size(Online,2)-1);\n\np_onii = Online(:,2:size(Online,2));\n\np_offi = Offline(:,1:size(Offline,2)-1);\n\np_offii = Offline(:,2:size(Offline,2));\n\nInside = (p_oni.*p_offii)./(p_onii.*p_offi);\n\ndel_cross = 1./(2.*(sigma_on_total(1:size(Online,2)-1)-sigma_off_total(1:size(Offline,2)-1)).*75*100);\n\ndel_cross(isinf(del_cross)) = 0;\n\n%Calculating Number density\nN = del_cross.*log(Inside);\n\n%Spatial smoothing of the profiles\nfilter1 = ones(1,2)./2;\n\nN_1 = N;\n\nN_1_avg = filter2(filter1,N_1);\n\nfilter1 = ones(1,10)./10;\n\nN_2 = N;\n\nN_2_avg = filter2(filter1,N_2);\n\nN_new = zeros(size(N,1),size(N,2));\n \n%Using different averaging windows for different altitudes \nN_avg=[N_1_avg(:,1:40)';N_2_avg(:,41:size(N,2))']';\n\n\nw = N_avg.*1e6.*18.015./6.022e23"("Online"=w608, "Offline"=w607, "sigma_on_total"=w606, "sigma_off_total"=w609) -> ("N_avg"=w610:cdb[], "w"=w619:cdb[])  [unwired: 1 in, 1 out]
                n448 = script code="%Time averaging in seconds.  180 Seconds = 3 minutes\ntemporal_average = 180;\n\n%Spatial averaging in bins.  2 bins = 150 meters\nspatial_average = 2;\n\n%Creating r and r+deltar vectors..this can also be acsomplished using the\n%diff command\np_oni = Online(:,1:size(Online,2)-1);\n\np_onii = Online(:,2:size(Online,2));\n\np_offi = Offline(:,1:size(Offline,2)-1);\n\np_offii = Offline(:,2:size(Offline,2));\n\nInside = (p_oni.*p_offii)./(p_onii.*p_offi);\n\ndel_cross = 1./(2.*(sigma_on_total(1:size(Online,2)-1)-sigma_off_total(1:size(Offline,2)-1)).*75*100);\n\ndel_cross(isinf(del_cross)) = 0;\n\n%Calculating Number density\nN = del_cross.*log(Inside);\n\n%Spatial smoothing of the profiles\nfilter1 = ones(1,2)./2;\n\nN_1 = N;\n\nN_1_avg = filter2(filter1,N_1);\n\nfilter1 = ones(1,10)./10;\n\nN_2 = N;\n\nN_2_avg = filter2(filter1,N_2);\n\nN_new = zeros(size(N,1),size(N,2));\n \n%Using different averaging windows for different altitudes \nN_avg=[N_1_avg(:,1:40)';N_2_avg(:,41:size(N,2))']';\n\n \nw = N_avg.*1e6.*18.015./6.022e23"("Online"=w584, "Offline"=w583, "sigma_on_total"=w606, "sigma_off_total"=w609) -> ("N_avg"=w615:cdb[], "w"=w616:cdb[])  [unwired: 1 in, 1 out]
                n449 = local read "Time Resolution Per Bin(ns)"() -> (w585:u32)
                n450 = local read "bins"() -> (w611:u32)
                n451 = local read "Altitude Array (km)"() -> (w581:dbl[])
                n452 = Build Array(w616, w619) -> (w622:cdb[][])
                n453 = To Double Precision Float(number=w585) -> (double precision float=w604:dbl)
                n454 = Reshape Array(w615, w586, w611) -> (w626:cdb[][])
                n455 = Reshape Array(w610, w586, w611) -> (w613:cdb[][])
                n456 = Multiply(x=0.15, y=w604) -> (x*y=w602:dbl)
                n457 = Build Array(w615, w610) -> (w620:cdb[][])
                n458 = Divide(x=300.0, y=w602) -> (x/y=w599:dbl)
                n459 = Divide(x=450.0, y=w602) -> (x/y=w598:dbl)
                n460 = Build Array(w581, w581) -> (w605:dbl[][])
                n461 = call "Convert to Dynamic Data5"("2D Array"=w622) -> ("Dynamic Data Type"=w621:dynamicdata)  [unwired: 3 in]
                n462 = call "Convert to Dynamic Data2"("2D Array"=w620) -> ("Dynamic Data Type"=w617:dynamicdata)  [unwired: 3 in]
                n463 = Divide(x=w626, y=1e+17) -> (x/y=→"Water Vapor Number Density":cdb[][])
                n464 = Divide(x=w613, y=1e+17) -> (x/y=→"Water Vapor Number Density 2":cdb[][])
                n465 = call "Convert to Dynamic Data6"("Array"=w581) -> ("Dynamic Data Type"=w582:dynamicdata)  [unwired: 3 in]
                n466 = To Long Integer(number=w599) -> (32bit integer=w597:i32)
                n467 = To Long Integer(number=w598) -> (32bit integer=w596:i32)
                n468 = call "Convert to Dynamic Data"("2D Array"=w605) -> ("Dynamic Data Type"=w618:dynamicdata)  [unwired: 3 in]
                n469 = call "Convert to Dynamic Data8"("2D Array"=w605) -> ("Dynamic Data Type"=w623:dynamicdata)  [unwired: 3 in]
                n470 = Decrement(x=w597) -> (x-1=w594:i32)
                n471 = Decrement(x=w596) -> (x-1=w595:i32)
                n472 = call "Build XY Graph"("Y Input"=w618, "X Input"=w617) -> ("XY Graph"=→"Water Vapor Number Density  2":cluster{"Y":dbl[], "Y":dbl[]}[])  [unwired: 3 in, 6 out]
                n473 = call "Build XY Graph3"("Y Input"=w623, "X Input"=w621) -> ("XY Graph"=→"Absolute Humidity":cluster{"Y":dbl[], "Y":dbl[]}[])  [unwired: 3 in, 6 out]
                n474 = Array Subset(array=w584, index=w594, length=w595) -> (w593:dbl[])
                n475 = Array Subset(array=w583, index=w594, length=w595) -> (w592:dbl[])
                n476 = call-poly <vilib>:"Mean.vi"("X"=w593) -> ("mean"=w591:dbl)  [unwired: 1 out]
                n477 = call-poly <vilib>:"Mean.vi"("X"=w592) -> ("mean"=w590:dbl)  [unwired: 1 out]
                n478 = Divide(x=w591, y=w590) -> (x/y=w589:dbl)
                n479 = Multiply(x=w583, y=w589) -> (x*y=w588:dbl[])
                n480 = Divide(x=w584, y=w588) -> (x/y=w587:dbl[])
                n481 = Natural Logarithm(1:w587) -> (0:w578:dbl[])
                n482 = Multiply(x=-1.0, y=w578) -> (x*y=w577:dbl[])
                n483 = call "Convert to Dynamic Data9"("Array"=w577) -> ("Dynamic Data Type"=w580:dynamicdata)  [unwired: 3 in]
                n484 = call "Build OD Plot"("Y Input"=w582, "X Input"=w580) -> ("XY Graph"=→"Optical Depth":cluster{"Y":dbl[], "Y":dbl[]}[])  [unwired: 3 in, 6 out]
              }
            }
          }
        }
        "L_Count" <- w129
      }
    }
  }
  n485 = case shown="True" w3 {
    frame False {
    }
    frame True {
      # "close data files"
      # "Close Bristol WM"
      n486 = local read "Bristol Out"() -> (w633:i32)
      n487 = local read "NF_Off_Ref"() -> (w629:refnum<file>)
      n488 = local read "NF_On_Ref"() -> (w630:refnum<file>)
      n489 = local read "FF_Off_Ref"() -> (w631:refnum<file>)
      n490 = local read "FF_On_Ref"() -> (w632:refnum<file>)
      n491 = dll-call lib="C:/H2O_DIAL/LabVIEW-2012/Bristol WM V2_31b/CLDevIFace.dll" fn="CLCloseDevice"("CommPort"=w633) -> ()  [unwired: 5 in, 2 out]
      n492 = Close File(refnum=w632) -> ()  [unwired: 1 in, 2 out]
      n493 = Close File(refnum=w631) -> ()  [unwired: 1 in, 2 out]
      n494 = Close File(refnum=w630) -> ()  [unwired: 1 in, 2 out]
      n495 = Close File(refnum=w629) -> ()  [unwired: 1 in, 2 out]
    }
  }
  "FileHour" <- -1 ("FileHour")
  "DataOpen" <- FALSE
